vi "Control main.vi"(8 "New direction":string, 11 "Current Direction":string) -> ()   [LabVIEW 2015]
uses:
  <vilib>/myRIO/Instrument Drivers/Onboard IO/PWM/typedefs/PWM Reference.ctl
  <vilib>/myRIO/Common/Instrument Driver Framework/Utilities/typedefs/myRIO Generic Hardware Reference.ctl
  <vilib>/myRIO/Common/Instrument Driver Framework/Utilities/typedefs/Hardware Version Enum.ctl
  <vilib>/myRIO/Common/Instrument Driver Framework/Utilities/typedefs/myRIO v1.0 Reference.ctl
  <vilib>/myRIO/Common/Instrument Driver Framework/Utilities/typedefs/Generic FPGA Reference.ctl
  <vilib>/myRIO/Common/Instrument Driver Framework/myRIO v1.0/PWM/typedefs/PWM Channels Enum.ctl
  <vilib>/myRIO/Instrument Drivers/Onboard IO/PWM/typedefs/PWM Configuration.ctl
  <vilib>/userdefined/High Color/nirio_resource_hc.ctl
  <vilib>/myRIO/Common/Instrument Driver Framework/Utilities/vis/Is FPGA Ref Available.vi
  <vilib>/myRIO/Common/Instrument Driver Framework/myRIO v1.0/PWM/vis/myRIO v1.1 Open PWM.vi
  <vilib>/myRIO/Instrument Drivers/Onboard IO/PWM/vis/Set Duty Cycle and Frequency.vi
  <vilib>/myRIO/Common/Instrument Driver Framework/Utilities/vis/Validate Channels.vi
  <vilib>/myRIO/Common/Instrument Driver Framework/myRIO v1.0/PWM/vis/myRIO v1.0 Reserve PWM.vi
  <vilib>/myRIO/Common/Instrument Driver Framework/myRIO v1.0/PWM/vis/myRIO v1.0 Build MUX Configuration PWM.vi
  <vilib>/myRIO/Common/Instrument Driver Framework/myRIO v1.0/Resource Manager/vis/myRIO v1.0 Reserve Channel List.vi
  <vilib>/myRIO/Common/Instrument Driver Framework/myRIO v1.0/Resource Manager/vis/myRIO v1.0 Create Configuration List.vi
  <vilib>/myRIO/Common/Instrument Driver Framework/myRIO v1.0/Resource Manager/vis/myRIO v1.0 Reserve Channel.vi
  <vilib>/myRIO/Common/Instrument Driver Framework/myRIO v1.0/Resource Manager/vis/myRIO v1.0 Unreserve Channel.vi
  <vilib>/myRIO/Common/Instrument Driver Framework/myRIO v1.0/Resource Manager/vis/myRIO v1.0 Build Mutex Name.vi
  <vilib>/Utility/VariantDataType/GetNumericInfo.vi
  <vilib>/Utility/error.llb/Error Cluster From Error Code.vi
  <vilib>/myRIO/Common/Instrument Driver Framework/myRIO v1.0/myRIO v1.1 Open.vi
  <vilib>/myRIO/Common/Instrument Driver Framework/Utilities/vis/IO Manager.vi
  <vilib>/myRIO/Common/Instrument Driver Framework/Utilities/vis/Configuration Manager.vi
  <vilib>/myRIO/Common/Instrument Driver Framework/myRIO v1.0/Resource Manager/vis/myRIO v1.0 Configure IO.vi
  <vilib>/myRIO/Common/Instrument Driver Framework/myRIO v1.0/myRIO v1.0 Close.vi
  <vilib>/myRIO/Common/Instrument Driver Framework/myRIO v1.0/PWM/vis/myRIO v1.0 Write PWM.vi
  <vilib>/myRIO/Express VI/Onboard IO/PWM/PWM Express VI.xnode
  <vilib>/myRIO/Instrument Drivers/Onboard IO/PWM/vis/myRIO PWM Open.xnode
  <vilib>/myRIO/Instrument Drivers/Onboard IO/PWM/PWM.lvlib
panel:
  in  "error in (no error) 2":errorcluster
  out "error out 5":errorcluster
  out "error out 4":errorcluster
  out "Current location":dbl
  out "First location":dbl
  out "Final location":dbl
  out "remainder":dbl
  in  "chosen  distance":dbl
  out "error out":errorcluster
  in  "error in (no error)":errorcluster
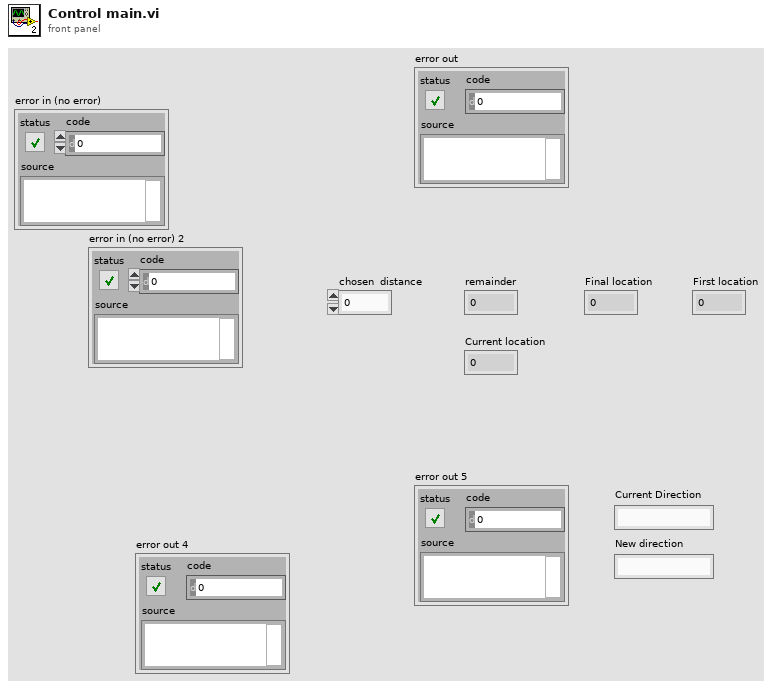
[diagram p1: front panel]
types:
  T1 = typedef "PWM.lvlib/PWM Reference.ctl" = cluster{"myRIO Reference":T2, "PWM Channels Enum":T6, "PWM Configuration":T7}
  T2 = typedef "myRIO Generic Hardware Reference.ctl" = cluster{"myRIO Model":T3, "myRIO Hardware Reference":T4}
  T3 = typedef "Hardware Version Enum.ctl" = enum16{"Unknown", "myRIO-1900", "myRIO-1950", "roboRIO"}
  T4 = typedef "myRIO v1.0 Reference.ctl" = cluster{"Generic FPGA Reference":T5, "Allow multiple opens":bool}
  T5 = typedef "Generic FPGA Reference.ctl" = refnum<k20>
  T6 = typedef "PWM Channels Enum.ctl" = enum16{"Not Connected", "C/PWM0", "C/PWM1", "A/PWM0", "A/PWM1", "A/PWM2", "B/PWM0", "B/PWM1", "B/PWM2", "PWM/PWM0", "PWM/PWM1", "PWM/PWM2", "PWM/PWM3", "PWM/PWM4", "PWM/PWM5", "PWM/PWM6", "PWM/PWM7", "PWM/PWM8", "PWM/PWM9"}
  T7 = typedef "PWM.lvlib/PWM Configuration.ctl" = cluster{"Frequency":dbl, "Duty Cycle":dbl}
  T8 = typedef "nirio_resource_hc.ctl" = tag
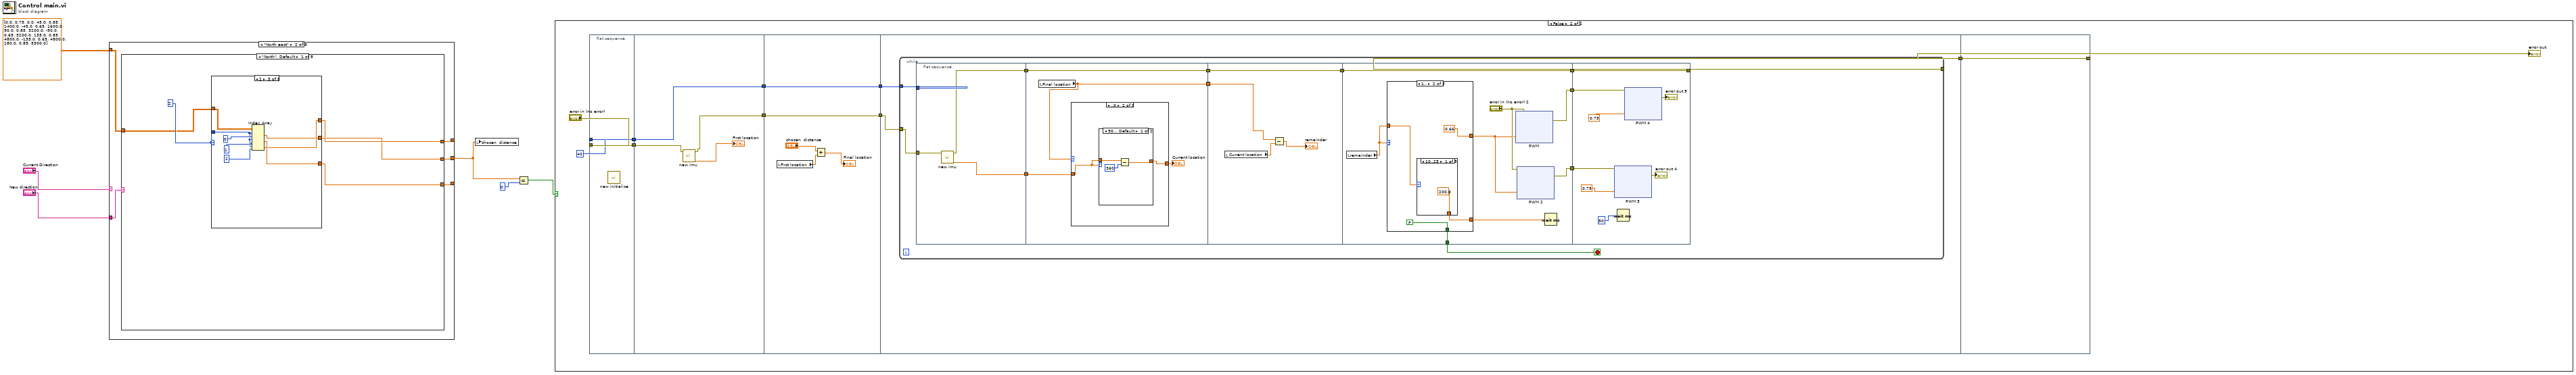
[diagram p0: block diagram]
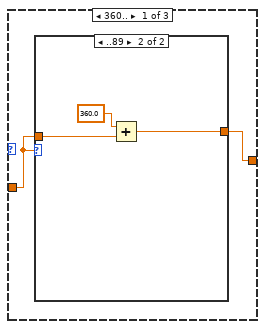
[diagram p3: hidden frame]
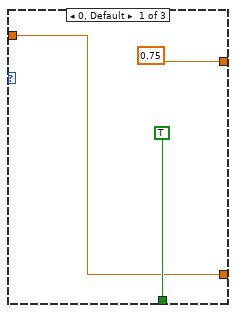
[diagram p7: hidden frame]
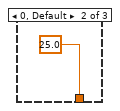
[diagram p8: hidden frame]
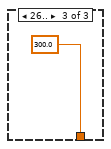
[diagram p9: hidden frame]
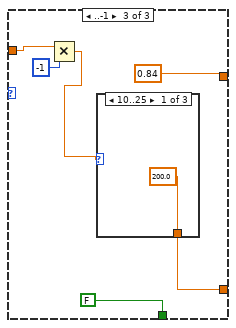
[diagram p10: hidden frame]
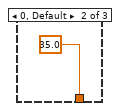
[diagram p11: hidden frame]
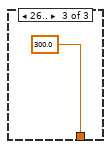
[diagram p12: hidden frame]
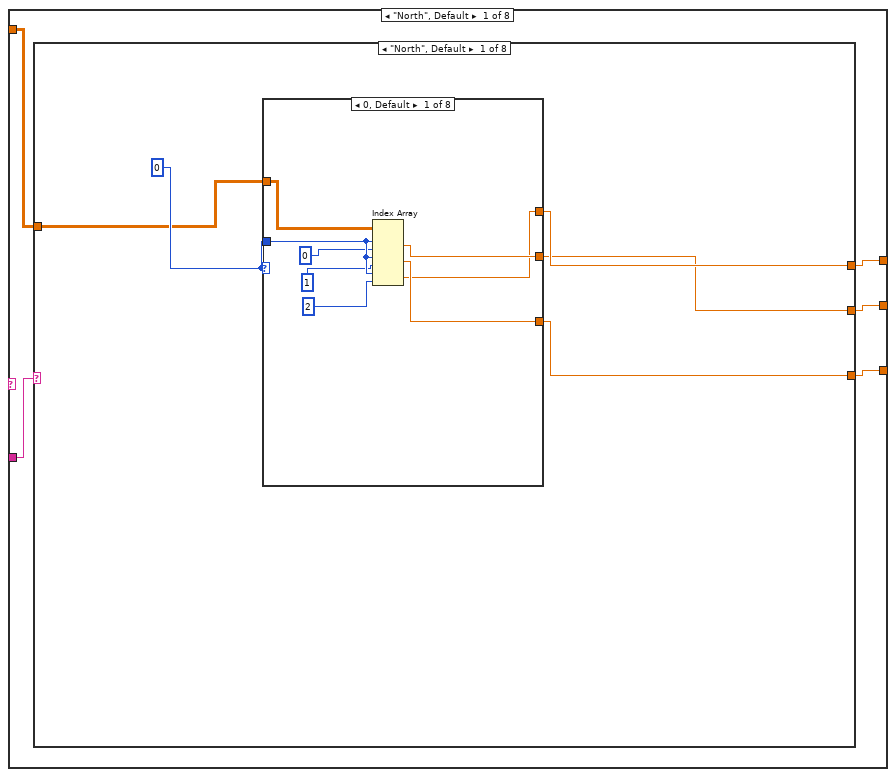
[diagram p13: hidden frame]
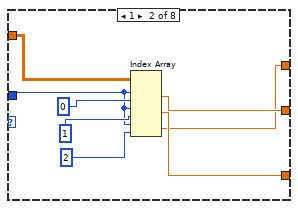
[diagram p14: hidden frame]
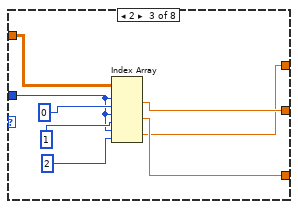
[diagram p15: hidden frame]
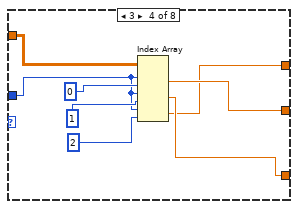
[diagram p16: hidden frame]
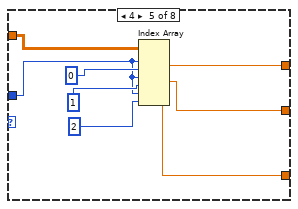
[diagram p17: hidden frame]
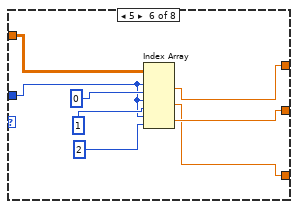
[diagram p18: hidden frame]
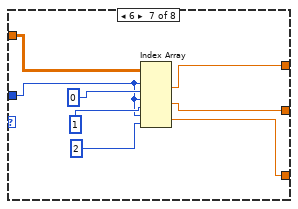
[diagram p19: hidden frame]
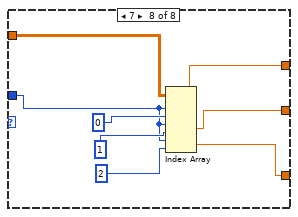
[diagram p20: hidden frame]
diagram:
  n1 = case shown="\"North east\"" "Current Direction" {
    tunnel: [w11 w568 w1125 w1682 w2239 w2796 w3353 w3910] -> _
    tunnel: [w10 w567 w1124 w1681 w2238 w2795 w3352 w3909] -> w2
    tunnel: [w9 w566 w1123 w1680 w2237 w2794 w3351 w3908] -> _
    tunnel: "New direction" -> [w7 w565 w1122 w1679 w2236 w2793 w3350 w3907]
    tunnel: dbl[][] [[0.0, 0.75, 0.0], [45.0, 0.85, 1400.0], [-45.0, 0.65, 1600.0], [90.0, 0.85, 3200.0], [-90.0, 0.65, 3200.0], [135.0, 0.85, 4800.0], [-135.0, 0.65, 4800.0], [180.0, 0.85, 5300.0]] -> [w8 w564 w1121 w1678 w2235 w2792 w3349 w3906]
    frame "North", Default {
      n2 = case shown="\"North\", Default" w7 {
        tunnel: [w15 w85 w153 w220 w290 w360 w428 w498] -> w11
        tunnel: [w14 w84 w152 w221 w289 w358 w427 w497] -> w10
        tunnel: [w13 w83 w151 w219 w288 w357 w426 w496] -> w9
        tunnel: w8 -> [w12 w81 w150 w222 w291 w359 w429 w495]
        frame "North", Default {
          w16 = 0
          n3 = case shown="0, Default" w16 {
            tunnel: [w20 w26 w34 w42 w50 w59 w66 w75] -> w15
            tunnel: [w22 w28 w36 w43 w52 w61 w68 w77] -> w14
            tunnel: [w21 w27 w35 w44 w51 w60 w67 w76] -> w13
            tunnel: w16 -> [w24 w29 w37 w45 w53 w58 w69 w74]
            tunnel: w12 -> [w17 w25 w33 w41 w49 w57 w65 w73]
            frame 0, Default {
              n4 = Index Array(array=w17, index (row) #1=w24, index (col) #1=0, index (row) #2=w24, index (col) #2=1, index (row) #3=w24, index (col) #3=2) -> (element #1=w22:dbl, element #2=w21:dbl, element #3=w20:dbl)
            }
            frame 1 {
              n5 = Index Array(array=w25, index (row) #1=w29, index (col) #1=0, index (row) #2=w29, index (col) #2=1, index (row) #3=w29, index (col) #3=2) -> (element #1=w28:dbl, element #2=w27:dbl, element #3=w26:dbl)
            }
            frame 2 {
              n6 = Index Array(array=w33, index (row) #1=w37, index (col) #1=0, index (row) #2=w37, index (col) #2=1, index (row) #3=w37, index (col) #3=2) -> (element #1=w36:dbl, element #2=w35:dbl, element #3=w34:dbl)
            }
            frame 3 {
              n7 = Index Array(array=w41, index (row) #1=w45, index (col) #1=0, index (row) #2=w45, index (col) #2=1, index (row) #3=w45, index (col) #3=2) -> (element #1=w43:dbl, element #2=w44:dbl, element #3=w42:dbl)
            }
            frame 4 {
              n8 = Index Array(array=w49, index (row) #1=w53, index (col) #1=0, index (row) #2=w53, index (col) #2=1, index (row) #3=w53, index (col) #3=2) -> (element #1=w50:dbl, element #2=w52:dbl, element #3=w51:dbl)
            }
            frame 5 {
              n9 = Index Array(array=w57, index (row) #1=w58, index (col) #1=0, index (row) #2=w58, index (col) #2=1, index (row) #3=w58, index (col) #3=2) -> (element #1=w59:dbl, element #2=w60:dbl, element #3=w61:dbl)
            }
            frame 6 {
              n10 = Index Array(array=w65, index (row) #1=w69, index (col) #1=0, index (row) #2=w69, index (col) #2=1, index (row) #3=w69, index (col) #3=2) -> (element #1=w66:dbl, element #2=w68:dbl, element #3=w67:dbl)
            }
            frame 7 {
              n11 = Index Array(array=w73, index (row) #1=w74, index (col) #1=0, index (row) #2=w74, index (col) #2=1, index (row) #3=w74, index (col) #3=2) -> (element #1=w75:dbl, element #2=w77:dbl, element #3=w76:dbl)
            }
          }
        }
        frame "North east" {
          w82 = 1
          n12 = case shown="2" w82 {
            tunnel: [w89 w95 w103 w111 w119 w128 w135 w144] -> w85
            tunnel: [w91 w97 w105 w112 w121 w130 w137 w146] -> w84
            tunnel: [w90 w96 w104 w113 w120 w129 w136 w145] -> w83
            tunnel: w82 -> [w93 w98 w106 w114 w122 w127 w138 w143]
            tunnel: w81 -> [w86 w94 w102 w110 w118 w126 w134 w142]
            frame 0, Default {
              n13 = Index Array(array=w86, index (row) #1=w93, index (col) #1=0, index (row) #2=w93, index (col) #2=1, index (row) #3=w93, index (col) #3=2) -> (element #1=w91:dbl, element #2=w90:dbl, element #3=w89:dbl)
            }
            frame 1 {
              n14 = Index Array(array=w94, index (row) #1=w98, index (col) #1=0, index (row) #2=w98, index (col) #2=1, index (row) #3=w98, index (col) #3=2) -> (element #1=w97:dbl, element #2=w96:dbl, element #3=w95:dbl)
            }
            frame 2 {
              n15 = Index Array(array=w102, index (row) #1=w106, index (col) #1=0, index (row) #2=w106, index (col) #2=1, index (row) #3=w106, index (col) #3=2) -> (element #1=w105:dbl, element #2=w104:dbl, element #3=w103:dbl)
            }
            frame 3 {
              n16 = Index Array(array=w110, index (row) #1=w114, index (col) #1=0, index (row) #2=w114, index (col) #2=1, index (row) #3=w114, index (col) #3=2) -> (element #1=w112:dbl, element #2=w113:dbl, element #3=w111:dbl)
            }
            frame 4 {
              n17 = Index Array(array=w118, index (row) #1=w122, index (col) #1=0, index (row) #2=w122, index (col) #2=1, index (row) #3=w122, index (col) #3=2) -> (element #1=w119:dbl, element #2=w121:dbl, element #3=w120:dbl)
            }
            frame 5 {
              n18 = Index Array(array=w126, index (row) #1=w127, index (col) #1=0, index (row) #2=w127, index (col) #2=1, index (row) #3=w127, index (col) #3=2) -> (element #1=w128:dbl, element #2=w129:dbl, element #3=w130:dbl)
            }
            frame 6 {
              n19 = Index Array(array=w134, index (row) #1=w138, index (col) #1=0, index (row) #2=w138, index (col) #2=1, index (row) #3=w138, index (col) #3=2) -> (element #1=w135:dbl, element #2=w137:dbl, element #3=w136:dbl)
            }
            frame 7 {
              n20 = Index Array(array=w142, index (row) #1=w143, index (col) #1=0, index (row) #2=w143, index (col) #2=1, index (row) #3=w143, index (col) #3=2) -> (element #1=w144:dbl, element #2=w146:dbl, element #3=w145:dbl)
            }
          }
        }
        frame "North west" {
          w154 = 2
          n21 = case shown="2" w154 {
            tunnel: [w158 w164 w172 w180 w188 w197 w204 w213] -> w153
            tunnel: [w160 w166 w174 w181 w190 w199 w206 w215] -> w152
            tunnel: [w159 w165 w173 w182 w189 w198 w205 w214] -> w151
            tunnel: w154 -> [w162 w167 w175 w183 w191 w196 w207 w212]
            tunnel: w150 -> [w155 w163 w171 w179 w187 w195 w203 w211]
            frame 0, Default {
              n22 = Index Array(array=w155, index (row) #1=w162, index (col) #1=0, index (row) #2=w162, index (col) #2=1, index (row) #3=w162, index (col) #3=2) -> (element #1=w160:dbl, element #2=w159:dbl, element #3=w158:dbl)
            }
            frame 1 {
              n23 = Index Array(array=w163, index (row) #1=w167, index (col) #1=0, index (row) #2=w167, index (col) #2=1, index (row) #3=w167, index (col) #3=2) -> (element #1=w166:dbl, element #2=w165:dbl, element #3=w164:dbl)
            }
            frame 2 {
              n24 = Index Array(array=w171, index (row) #1=w175, index (col) #1=0, index (row) #2=w175, index (col) #2=1, index (row) #3=w175, index (col) #3=2) -> (element #1=w174:dbl, element #2=w173:dbl, element #3=w172:dbl)
            }
            frame 3 {
              n25 = Index Array(array=w179, index (row) #1=w183, index (col) #1=0, index (row) #2=w183, index (col) #2=1, index (row) #3=w183, index (col) #3=2) -> (element #1=w181:dbl, element #2=w182:dbl, element #3=w180:dbl)
            }
            frame 4 {
              n26 = Index Array(array=w187, index (row) #1=w191, index (col) #1=0, index (row) #2=w191, index (col) #2=1, index (row) #3=w191, index (col) #3=2) -> (element #1=w188:dbl, element #2=w190:dbl, element #3=w189:dbl)
            }
            frame 5 {
              n27 = Index Array(array=w195, index (row) #1=w196, index (col) #1=0, index (row) #2=w196, index (col) #2=1, index (row) #3=w196, index (col) #3=2) -> (element #1=w197:dbl, element #2=w198:dbl, element #3=w199:dbl)
            }
            frame 6 {
              n28 = Index Array(array=w203, index (row) #1=w207, index (col) #1=0, index (row) #2=w207, index (col) #2=1, index (row) #3=w207, index (col) #3=2) -> (element #1=w204:dbl, element #2=w206:dbl, element #3=w205:dbl)
            }
            frame 7 {
              n29 = Index Array(array=w211, index (row) #1=w212, index (col) #1=0, index (row) #2=w212, index (col) #2=1, index (row) #3=w212, index (col) #3=2) -> (element #1=w213:dbl, element #2=w215:dbl, element #3=w214:dbl)
            }
          }
        }
        frame "West" {
          w223 = 4
          n30 = case shown="2" w223 {
            tunnel: [w227 w233 w241 w249 w257 w266 w273 w282] -> w220
            tunnel: [w229 w235 w243 w250 w259 w268 w275 w284] -> w221
            tunnel: [w228 w234 w242 w251 w258 w267 w274 w283] -> w219
            tunnel: w223 -> [w231 w236 w244 w252 w260 w265 w276 w281]
            tunnel: w222 -> [w224 w232 w240 w248 w256 w264 w272 w280]
            frame 0, Default {
              n31 = Index Array(array=w224, index (row) #1=w231, index (col) #1=0, index (row) #2=w231, index (col) #2=1, index (row) #3=w231, index (col) #3=2) -> (element #1=w229:dbl, element #2=w228:dbl, element #3=w227:dbl)
            }
            frame 1 {
              n32 = Index Array(array=w232, index (row) #1=w236, index (col) #1=0, index (row) #2=w236, index (col) #2=1, index (row) #3=w236, index (col) #3=2) -> (element #1=w235:dbl, element #2=w234:dbl, element #3=w233:dbl)
            }
            frame 2 {
              n33 = Index Array(array=w240, index (row) #1=w244, index (col) #1=0, index (row) #2=w244, index (col) #2=1, index (row) #3=w244, index (col) #3=2) -> (element #1=w243:dbl, element #2=w242:dbl, element #3=w241:dbl)
            }
            frame 3 {
              n34 = Index Array(array=w248, index (row) #1=w252, index (col) #1=0, index (row) #2=w252, index (col) #2=1, index (row) #3=w252, index (col) #3=2) -> (element #1=w250:dbl, element #2=w251:dbl, element #3=w249:dbl)
            }
            frame 4 {
              n35 = Index Array(array=w256, index (row) #1=w260, index (col) #1=0, index (row) #2=w260, index (col) #2=1, index (row) #3=w260, index (col) #3=2) -> (element #1=w257:dbl, element #2=w259:dbl, element #3=w258:dbl)
            }
            frame 5 {
              n36 = Index Array(array=w264, index (row) #1=w265, index (col) #1=0, index (row) #2=w265, index (col) #2=1, index (row) #3=w265, index (col) #3=2) -> (element #1=w266:dbl, element #2=w267:dbl, element #3=w268:dbl)
            }
            frame 6 {
              n37 = Index Array(array=w272, index (row) #1=w276, index (col) #1=0, index (row) #2=w276, index (col) #2=1, index (row) #3=w276, index (col) #3=2) -> (element #1=w273:dbl, element #2=w275:dbl, element #3=w274:dbl)
            }
            frame 7 {
              n38 = Index Array(array=w280, index (row) #1=w281, index (col) #1=0, index (row) #2=w281, index (col) #2=1, index (row) #3=w281, index (col) #3=2) -> (element #1=w282:dbl, element #2=w284:dbl, element #3=w283:dbl)
            }
          }
        }
        frame "East" {
          w292 = 3
          n39 = case shown="2" w292 {
            tunnel: [w296 w302 w310 w318 w326 w335 w342 w351] -> w290
            tunnel: [w298 w304 w312 w319 w328 w337 w344 w353] -> w289
            tunnel: [w297 w303 w311 w320 w327 w336 w343 w352] -> w288
            tunnel: w292 -> [w300 w305 w313 w321 w329 w334 w345 w350]
            tunnel: w291 -> [w293 w301 w309 w317 w325 w333 w341 w349]
            frame 0, Default {
              n40 = Index Array(array=w293, index (row) #1=w300, index (col) #1=0, index (row) #2=w300, index (col) #2=1, index (row) #3=w300, index (col) #3=2) -> (element #1=w298:dbl, element #2=w297:dbl, element #3=w296:dbl)
            }
            frame 1 {
              n41 = Index Array(array=w301, index (row) #1=w305, index (col) #1=0, index (row) #2=w305, index (col) #2=1, index (row) #3=w305, index (col) #3=2) -> (element #1=w304:dbl, element #2=w303:dbl, element #3=w302:dbl)
            }
            frame 2 {
              n42 = Index Array(array=w309, index (row) #1=w313, index (col) #1=0, index (row) #2=w313, index (col) #2=1, index (row) #3=w313, index (col) #3=2) -> (element #1=w312:dbl, element #2=w311:dbl, element #3=w310:dbl)
            }
            frame 3 {
              n43 = Index Array(array=w317, index (row) #1=w321, index (col) #1=0, index (row) #2=w321, index (col) #2=1, index (row) #3=w321, index (col) #3=2) -> (element #1=w319:dbl, element #2=w320:dbl, element #3=w318:dbl)
            }
            frame 4 {
              n44 = Index Array(array=w325, index (row) #1=w329, index (col) #1=0, index (row) #2=w329, index (col) #2=1, index (row) #3=w329, index (col) #3=2) -> (element #1=w326:dbl, element #2=w328:dbl, element #3=w327:dbl)
            }
            frame 5 {
              n45 = Index Array(array=w333, index (row) #1=w334, index (col) #1=0, index (row) #2=w334, index (col) #2=1, index (row) #3=w334, index (col) #3=2) -> (element #1=w335:dbl, element #2=w336:dbl, element #3=w337:dbl)
            }
            frame 6 {
              n46 = Index Array(array=w341, index (row) #1=w345, index (col) #1=0, index (row) #2=w345, index (col) #2=1, index (row) #3=w345, index (col) #3=2) -> (element #1=w342:dbl, element #2=w344:dbl, element #3=w343:dbl)
            }
            frame 7 {
              n47 = Index Array(array=w349, index (row) #1=w350, index (col) #1=0, index (row) #2=w350, index (col) #2=1, index (row) #3=w350, index (col) #3=2) -> (element #1=w351:dbl, element #2=w353:dbl, element #3=w352:dbl)
            }
          }
        }
        frame "South" {
          w361 = 7
          n48 = case shown="2" w361 {
            tunnel: [w365 w371 w379 w387 w395 w404 w411 w420] -> w360
            tunnel: [w367 w373 w381 w388 w397 w406 w413 w422] -> w358
            tunnel: [w366 w372 w380 w389 w396 w405 w412 w421] -> w357
            tunnel: w361 -> [w369 w374 w382 w390 w398 w403 w414 w419]
            tunnel: w359 -> [w362 w370 w378 w386 w394 w402 w410 w418]
            frame 0, Default {
              n49 = Index Array(array=w362, index (row) #1=w369, index (col) #1=0, index (row) #2=w369, index (col) #2=1, index (row) #3=w369, index (col) #3=2) -> (element #1=w367:dbl, element #2=w366:dbl, element #3=w365:dbl)
            }
            frame 1 {
              n50 = Index Array(array=w370, index (row) #1=w374, index (col) #1=0, index (row) #2=w374, index (col) #2=1, index (row) #3=w374, index (col) #3=2) -> (element #1=w373:dbl, element #2=w372:dbl, element #3=w371:dbl)
            }
            frame 2 {
              n51 = Index Array(array=w378, index (row) #1=w382, index (col) #1=0, index (row) #2=w382, index (col) #2=1, index (row) #3=w382, index (col) #3=2) -> (element #1=w381:dbl, element #2=w380:dbl, element #3=w379:dbl)
            }
            frame 3 {
              n52 = Index Array(array=w386, index (row) #1=w390, index (col) #1=0, index (row) #2=w390, index (col) #2=1, index (row) #3=w390, index (col) #3=2) -> (element #1=w388:dbl, element #2=w389:dbl, element #3=w387:dbl)
            }
            frame 4 {
              n53 = Index Array(array=w394, index (row) #1=w398, index (col) #1=0, index (row) #2=w398, index (col) #2=1, index (row) #3=w398, index (col) #3=2) -> (element #1=w395:dbl, element #2=w397:dbl, element #3=w396:dbl)
            }
            frame 5 {
              n54 = Index Array(array=w402, index (row) #1=w403, index (col) #1=0, index (row) #2=w403, index (col) #2=1, index (row) #3=w403, index (col) #3=2) -> (element #1=w404:dbl, element #2=w405:dbl, element #3=w406:dbl)
            }
            frame 6 {
              n55 = Index Array(array=w410, index (row) #1=w414, index (col) #1=0, index (row) #2=w414, index (col) #2=1, index (row) #3=w414, index (col) #3=2) -> (element #1=w411:dbl, element #2=w413:dbl, element #3=w412:dbl)
            }
            frame 7 {
              n56 = Index Array(array=w418, index (row) #1=w419, index (col) #1=0, index (row) #2=w419, index (col) #2=1, index (row) #3=w419, index (col) #3=2) -> (element #1=w420:dbl, element #2=w422:dbl, element #3=w421:dbl)
            }
          }
        }
        frame "South west" {
          w430 = 6
          n57 = case shown="2" w430 {
            tunnel: [w434 w440 w448 w456 w464 w473 w480 w489] -> w428
            tunnel: [w436 w442 w450 w457 w466 w475 w482 w491] -> w427
            tunnel: [w435 w441 w449 w458 w465 w474 w481 w490] -> w426
            tunnel: w430 -> [w438 w443 w451 w459 w467 w472 w483 w488]
            tunnel: w429 -> [w431 w439 w447 w455 w463 w471 w479 w487]
            frame 0, Default {
              n58 = Index Array(array=w431, index (row) #1=w438, index (col) #1=0, index (row) #2=w438, index (col) #2=1, index (row) #3=w438, index (col) #3=2) -> (element #1=w436:dbl, element #2=w435:dbl, element #3=w434:dbl)
            }
            frame 1 {
              n59 = Index Array(array=w439, index (row) #1=w443, index (col) #1=0, index (row) #2=w443, index (col) #2=1, index (row) #3=w443, index (col) #3=2) -> (element #1=w442:dbl, element #2=w441:dbl, element #3=w440:dbl)
            }
            frame 2 {
              n60 = Index Array(array=w447, index (row) #1=w451, index (col) #1=0, index (row) #2=w451, index (col) #2=1, index (row) #3=w451, index (col) #3=2) -> (element #1=w450:dbl, element #2=w449:dbl, element #3=w448:dbl)
            }
            frame 3 {
              n61 = Index Array(array=w455, index (row) #1=w459, index (col) #1=0, index (row) #2=w459, index (col) #2=1, index (row) #3=w459, index (col) #3=2) -> (element #1=w457:dbl, element #2=w458:dbl, element #3=w456:dbl)
            }
            frame 4 {
              n62 = Index Array(array=w463, index (row) #1=w467, index (col) #1=0, index (row) #2=w467, index (col) #2=1, index (row) #3=w467, index (col) #3=2) -> (element #1=w464:dbl, element #2=w466:dbl, element #3=w465:dbl)
            }
            frame 5 {
              n63 = Index Array(array=w471, index (row) #1=w472, index (col) #1=0, index (row) #2=w472, index (col) #2=1, index (row) #3=w472, index (col) #3=2) -> (element #1=w473:dbl, element #2=w474:dbl, element #3=w475:dbl)
            }
            frame 6 {
              n64 = Index Array(array=w479, index (row) #1=w483, index (col) #1=0, index (row) #2=w483, index (col) #2=1, index (row) #3=w483, index (col) #3=2) -> (element #1=w480:dbl, element #2=w482:dbl, element #3=w481:dbl)
            }
            frame 7 {
              n65 = Index Array(array=w487, index (row) #1=w488, index (col) #1=0, index (row) #2=w488, index (col) #2=1, index (row) #3=w488, index (col) #3=2) -> (element #1=w489:dbl, element #2=w491:dbl, element #3=w490:dbl)
            }
          }
        }
        frame "South east" {
          w499 = 5
          n66 = case shown="2" w499 {
            tunnel: [w503 w509 w517 w525 w533 w542 w549 w558] -> w498
            tunnel: [w505 w511 w519 w526 w535 w544 w551 w560] -> w497
            tunnel: [w504 w510 w518 w527 w534 w543 w550 w559] -> w496
            tunnel: w499 -> [w507 w512 w520 w528 w536 w541 w552 w557]
            tunnel: w495 -> [w500 w508 w516 w524 w532 w540 w548 w556]
            frame 0, Default {
              n67 = Index Array(array=w500, index (row) #1=w507, index (col) #1=0, index (row) #2=w507, index (col) #2=1, index (row) #3=w507, index (col) #3=2) -> (element #1=w505:dbl, element #2=w504:dbl, element #3=w503:dbl)
            }
            frame 1 {
              n68 = Index Array(array=w508, index (row) #1=w512, index (col) #1=0, index (row) #2=w512, index (col) #2=1, index (row) #3=w512, index (col) #3=2) -> (element #1=w511:dbl, element #2=w510:dbl, element #3=w509:dbl)
            }
            frame 2 {
              n69 = Index Array(array=w516, index (row) #1=w520, index (col) #1=0, index (row) #2=w520, index (col) #2=1, index (row) #3=w520, index (col) #3=2) -> (element #1=w519:dbl, element #2=w518:dbl, element #3=w517:dbl)
            }
            frame 3 {
              n70 = Index Array(array=w524, index (row) #1=w528, index (col) #1=0, index (row) #2=w528, index (col) #2=1, index (row) #3=w528, index (col) #3=2) -> (element #1=w526:dbl, element #2=w527:dbl, element #3=w525:dbl)
            }
            frame 4 {
              n71 = Index Array(array=w532, index (row) #1=w536, index (col) #1=0, index (row) #2=w536, index (col) #2=1, index (row) #3=w536, index (col) #3=2) -> (element #1=w533:dbl, element #2=w535:dbl, element #3=w534:dbl)
            }
            frame 5 {
              n72 = Index Array(array=w540, index (row) #1=w541, index (col) #1=0, index (row) #2=w541, index (col) #2=1, index (row) #3=w541, index (col) #3=2) -> (element #1=w542:dbl, element #2=w543:dbl, element #3=w544:dbl)
            }
            frame 6 {
              n73 = Index Array(array=w548, index (row) #1=w552, index (col) #1=0, index (row) #2=w552, index (col) #2=1, index (row) #3=w552, index (col) #3=2) -> (element #1=w549:dbl, element #2=w551:dbl, element #3=w550:dbl)
            }
            frame 7 {
              n74 = Index Array(array=w556, index (row) #1=w557, index (col) #1=0, index (row) #2=w557, index (col) #2=1, index (row) #3=w557, index (col) #3=2) -> (element #1=w558:dbl, element #2=w560:dbl, element #3=w559:dbl)
            }
          }
        }
      }
    }
    frame "North east" {
      n75 = case shown="\"North\", Default" w565 {
        tunnel: [w572 w642 w710 w777 w847 w917 w985 w1055] -> w568
        tunnel: [w571 w641 w709 w778 w846 w915 w984 w1054] -> w567
        tunnel: [w570 w640 w708 w776 w845 w914 w983 w1053] -> w566
        tunnel: w564 -> [w569 w638 w707 w779 w848 w916 w986 w1052]
        frame "North", Default {
          w573 = 2
          n76 = case shown="2" w573 {
            tunnel: [w577 w583 w591 w599 w607 w616 w623 w632] -> w572
            tunnel: [w579 w585 w593 w600 w609 w618 w625 w634] -> w571
            tunnel: [w578 w584 w592 w601 w608 w617 w624 w633] -> w570
            tunnel: w573 -> [w581 w586 w594 w602 w610 w615 w626 w631]
            tunnel: w569 -> [w574 w582 w590 w598 w606 w614 w622 w630]
            frame 0, Default {
              n77 = Index Array(array=w574, index (row) #1=w581, index (col) #1=0, index (row) #2=w581, index (col) #2=1, index (row) #3=w581, index (col) #3=2) -> (element #1=w579:dbl, element #2=w578:dbl, element #3=w577:dbl)
            }
            frame 1 {
              n78 = Index Array(array=w582, index (row) #1=w586, index (col) #1=0, index (row) #2=w586, index (col) #2=1, index (row) #3=w586, index (col) #3=2) -> (element #1=w585:dbl, element #2=w584:dbl, element #3=w583:dbl)
            }
            frame 2 {
              n79 = Index Array(array=w590, index (row) #1=w594, index (col) #1=0, index (row) #2=w594, index (col) #2=1, index (row) #3=w594, index (col) #3=2) -> (element #1=w593:dbl, element #2=w592:dbl, element #3=w591:dbl)
            }
            frame 3 {
              n80 = Index Array(array=w598, index (row) #1=w602, index (col) #1=0, index (row) #2=w602, index (col) #2=1, index (row) #3=w602, index (col) #3=2) -> (element #1=w600:dbl, element #2=w601:dbl, element #3=w599:dbl)
            }
            frame 4 {
              n81 = Index Array(array=w606, index (row) #1=w610, index (col) #1=0, index (row) #2=w610, index (col) #2=1, index (row) #3=w610, index (col) #3=2) -> (element #1=w607:dbl, element #2=w609:dbl, element #3=w608:dbl)
            }
            frame 5 {
              n82 = Index Array(array=w614, index (row) #1=w615, index (col) #1=0, index (row) #2=w615, index (col) #2=1, index (row) #3=w615, index (col) #3=2) -> (element #1=w616:dbl, element #2=w617:dbl, element #3=w618:dbl)
            }
            frame 6 {
              n83 = Index Array(array=w622, index (row) #1=w626, index (col) #1=0, index (row) #2=w626, index (col) #2=1, index (row) #3=w626, index (col) #3=2) -> (element #1=w623:dbl, element #2=w625:dbl, element #3=w624:dbl)
            }
            frame 7 {
              n84 = Index Array(array=w630, index (row) #1=w631, index (col) #1=0, index (row) #2=w631, index (col) #2=1, index (row) #3=w631, index (col) #3=2) -> (element #1=w632:dbl, element #2=w634:dbl, element #3=w633:dbl)
            }
          }
        }
        frame "North east" {
          w639 = 0
          n85 = case shown="2" w639 {
            tunnel: [w646 w652 w660 w668 w676 w685 w692 w701] -> w642
            tunnel: [w648 w654 w662 w669 w678 w687 w694 w703] -> w641
            tunnel: [w647 w653 w661 w670 w677 w686 w693 w702] -> w640
            tunnel: w639 -> [w650 w655 w663 w671 w679 w684 w695 w700]
            tunnel: w638 -> [w643 w651 w659 w667 w675 w683 w691 w699]
            frame 0, Default {
              n86 = Index Array(array=w643, index (row) #1=w650, index (col) #1=0, index (row) #2=w650, index (col) #2=1, index (row) #3=w650, index (col) #3=2) -> (element #1=w648:dbl, element #2=w647:dbl, element #3=w646:dbl)
            }
            frame 1 {
              n87 = Index Array(array=w651, index (row) #1=w655, index (col) #1=0, index (row) #2=w655, index (col) #2=1, index (row) #3=w655, index (col) #3=2) -> (element #1=w654:dbl, element #2=w653:dbl, element #3=w652:dbl)
            }
            frame 2 {
              n88 = Index Array(array=w659, index (row) #1=w663, index (col) #1=0, index (row) #2=w663, index (col) #2=1, index (row) #3=w663, index (col) #3=2) -> (element #1=w662:dbl, element #2=w661:dbl, element #3=w660:dbl)
            }
            frame 3 {
              n89 = Index Array(array=w667, index (row) #1=w671, index (col) #1=0, index (row) #2=w671, index (col) #2=1, index (row) #3=w671, index (col) #3=2) -> (element #1=w669:dbl, element #2=w670:dbl, element #3=w668:dbl)
            }
            frame 4 {
              n90 = Index Array(array=w675, index (row) #1=w679, index (col) #1=0, index (row) #2=w679, index (col) #2=1, index (row) #3=w679, index (col) #3=2) -> (element #1=w676:dbl, element #2=w678:dbl, element #3=w677:dbl)
            }
            frame 5 {
              n91 = Index Array(array=w683, index (row) #1=w684, index (col) #1=0, index (row) #2=w684, index (col) #2=1, index (row) #3=w684, index (col) #3=2) -> (element #1=w685:dbl, element #2=w686:dbl, element #3=w687:dbl)
            }
            frame 6 {
              n92 = Index Array(array=w691, index (row) #1=w695, index (col) #1=0, index (row) #2=w695, index (col) #2=1, index (row) #3=w695, index (col) #3=2) -> (element #1=w692:dbl, element #2=w694:dbl, element #3=w693:dbl)
            }
            frame 7 {
              n93 = Index Array(array=w699, index (row) #1=w700, index (col) #1=0, index (row) #2=w700, index (col) #2=1, index (row) #3=w700, index (col) #3=2) -> (element #1=w701:dbl, element #2=w703:dbl, element #3=w702:dbl)
            }
          }
        }
        frame "North west" {
          w711 = 4
          n94 = case shown="2" w711 {
            tunnel: [w715 w721 w729 w737 w745 w754 w761 w770] -> w710
            tunnel: [w717 w723 w731 w738 w747 w756 w763 w772] -> w709
            tunnel: [w716 w722 w730 w739 w746 w755 w762 w771] -> w708
            tunnel: w711 -> [w719 w724 w732 w740 w748 w753 w764 w769]
            tunnel: w707 -> [w712 w720 w728 w736 w744 w752 w760 w768]
            frame 0, Default {
              n95 = Index Array(array=w712, index (row) #1=w719, index (col) #1=0, index (row) #2=w719, index (col) #2=1, index (row) #3=w719, index (col) #3=2) -> (element #1=w717:dbl, element #2=w716:dbl, element #3=w715:dbl)
            }
            frame 1 {
              n96 = Index Array(array=w720, index (row) #1=w724, index (col) #1=0, index (row) #2=w724, index (col) #2=1, index (row) #3=w724, index (col) #3=2) -> (element #1=w723:dbl, element #2=w722:dbl, element #3=w721:dbl)
            }
            frame 2 {
              n97 = Index Array(array=w728, index (row) #1=w732, index (col) #1=0, index (row) #2=w732, index (col) #2=1, index (row) #3=w732, index (col) #3=2) -> (element #1=w731:dbl, element #2=w730:dbl, element #3=w729:dbl)
            }
            frame 3 {
              n98 = Index Array(array=w736, index (row) #1=w740, index (col) #1=0, index (row) #2=w740, index (col) #2=1, index (row) #3=w740, index (col) #3=2) -> (element #1=w738:dbl, element #2=w739:dbl, element #3=w737:dbl)
            }
            frame 4 {
              n99 = Index Array(array=w744, index (row) #1=w748, index (col) #1=0, index (row) #2=w748, index (col) #2=1, index (row) #3=w748, index (col) #3=2) -> (element #1=w745:dbl, element #2=w747:dbl, element #3=w746:dbl)
            }
            frame 5 {
              n100 = Index Array(array=w752, index (row) #1=w753, index (col) #1=0, index (row) #2=w753, index (col) #2=1, index (row) #3=w753, index (col) #3=2) -> (element #1=w754:dbl, element #2=w755:dbl, element #3=w756:dbl)
            }
            frame 6 {
              n101 = Index Array(array=w760, index (row) #1=w764, index (col) #1=0, index (row) #2=w764, index (col) #2=1, index (row) #3=w764, index (col) #3=2) -> (element #1=w761:dbl, element #2=w763:dbl, element #3=w762:dbl)
            }
            frame 7 {
              n102 = Index Array(array=w768, index (row) #1=w769, index (col) #1=0, index (row) #2=w769, index (col) #2=1, index (row) #3=w769, index (col) #3=2) -> (element #1=w770:dbl, element #2=w772:dbl, element #3=w771:dbl)
            }
          }
        }
        frame "West" {
          w780 = 6
          n103 = case shown="2" w780 {
            tunnel: [w784 w790 w798 w806 w814 w823 w830 w839] -> w777
            tunnel: [w786 w792 w800 w807 w816 w825 w832 w841] -> w778
            tunnel: [w785 w791 w799 w808 w815 w824 w831 w840] -> w776
            tunnel: w780 -> [w788 w793 w801 w809 w817 w822 w833 w838]
            tunnel: w779 -> [w781 w789 w797 w805 w813 w821 w829 w837]
            frame 0, Default {
              n104 = Index Array(array=w781, index (row) #1=w788, index (col) #1=0, index (row) #2=w788, index (col) #2=1, index (row) #3=w788, index (col) #3=2) -> (element #1=w786:dbl, element #2=w785:dbl, element #3=w784:dbl)
            }
            frame 1 {
              n105 = Index Array(array=w789, index (row) #1=w793, index (col) #1=0, index (row) #2=w793, index (col) #2=1, index (row) #3=w793, index (col) #3=2) -> (element #1=w792:dbl, element #2=w791:dbl, element #3=w790:dbl)
            }
            frame 2 {
              n106 = Index Array(array=w797, index (row) #1=w801, index (col) #1=0, index (row) #2=w801, index (col) #2=1, index (row) #3=w801, index (col) #3=2) -> (element #1=w800:dbl, element #2=w799:dbl, element #3=w798:dbl)
            }
            frame 3 {
              n107 = Index Array(array=w805, index (row) #1=w809, index (col) #1=0, index (row) #2=w809, index (col) #2=1, index (row) #3=w809, index (col) #3=2) -> (element #1=w807:dbl, element #2=w808:dbl, element #3=w806:dbl)
            }
            frame 4 {
              n108 = Index Array(array=w813, index (row) #1=w817, index (col) #1=0, index (row) #2=w817, index (col) #2=1, index (row) #3=w817, index (col) #3=2) -> (element #1=w814:dbl, element #2=w816:dbl, element #3=w815:dbl)
            }
            frame 5 {
              n109 = Index Array(array=w821, index (row) #1=w822, index (col) #1=0, index (row) #2=w822, index (col) #2=1, index (row) #3=w822, index (col) #3=2) -> (element #1=w823:dbl, element #2=w824:dbl, element #3=w825:dbl)
            }
            frame 6 {
              n110 = Index Array(array=w829, index (row) #1=w833, index (col) #1=0, index (row) #2=w833, index (col) #2=1, index (row) #3=w833, index (col) #3=2) -> (element #1=w830:dbl, element #2=w832:dbl, element #3=w831:dbl)
            }
            frame 7 {
              n111 = Index Array(array=w837, index (row) #1=w838, index (col) #1=0, index (row) #2=w838, index (col) #2=1, index (row) #3=w838, index (col) #3=2) -> (element #1=w839:dbl, element #2=w841:dbl, element #3=w840:dbl)
            }
          }
        }
        frame "East" {
          w849 = 1
          n112 = case shown="2" w849 {
            tunnel: [w853 w859 w867 w875 w883 w892 w899 w908] -> w847
            tunnel: [w855 w861 w869 w876 w885 w894 w901 w910] -> w846
            tunnel: [w854 w860 w868 w877 w884 w893 w900 w909] -> w845
            tunnel: w849 -> [w857 w862 w870 w878 w886 w891 w902 w907]
            tunnel: w848 -> [w850 w858 w866 w874 w882 w890 w898 w906]
            frame 0, Default {
              n113 = Index Array(array=w850, index (row) #1=w857, index (col) #1=0, index (row) #2=w857, index (col) #2=1, index (row) #3=w857, index (col) #3=2) -> (element #1=w855:dbl, element #2=w854:dbl, element #3=w853:dbl)
            }
            frame 1 {
              n114 = Index Array(array=w858, index (row) #1=w862, index (col) #1=0, index (row) #2=w862, index (col) #2=1, index (row) #3=w862, index (col) #3=2) -> (element #1=w861:dbl, element #2=w860:dbl, element #3=w859:dbl)
            }
            frame 2 {
              n115 = Index Array(array=w866, index (row) #1=w870, index (col) #1=0, index (row) #2=w870, index (col) #2=1, index (row) #3=w870, index (col) #3=2) -> (element #1=w869:dbl, element #2=w868:dbl, element #3=w867:dbl)
            }
            frame 3 {
              n116 = Index Array(array=w874, index (row) #1=w878, index (col) #1=0, index (row) #2=w878, index (col) #2=1, index (row) #3=w878, index (col) #3=2) -> (element #1=w876:dbl, element #2=w877:dbl, element #3=w875:dbl)
            }
            frame 4 {
              n117 = Index Array(array=w882, index (row) #1=w886, index (col) #1=0, index (row) #2=w886, index (col) #2=1, index (row) #3=w886, index (col) #3=2) -> (element #1=w883:dbl, element #2=w885:dbl, element #3=w884:dbl)
            }
            frame 5 {
              n118 = Index Array(array=w890, index (row) #1=w891, index (col) #1=0, index (row) #2=w891, index (col) #2=1, index (row) #3=w891, index (col) #3=2) -> (element #1=w892:dbl, element #2=w893:dbl, element #3=w894:dbl)
            }
            frame 6 {
              n119 = Index Array(array=w898, index (row) #1=w902, index (col) #1=0, index (row) #2=w902, index (col) #2=1, index (row) #3=w902, index (col) #3=2) -> (element #1=w899:dbl, element #2=w901:dbl, element #3=w900:dbl)
            }
            frame 7 {
              n120 = Index Array(array=w906, index (row) #1=w907, index (col) #1=0, index (row) #2=w907, index (col) #2=1, index (row) #3=w907, index (col) #3=2) -> (element #1=w908:dbl, element #2=w910:dbl, element #3=w909:dbl)
            }
          }
        }
        frame "South" {
          w918 = 5
          n121 = case shown="2" w918 {
            tunnel: [w922 w928 w936 w944 w952 w961 w968 w977] -> w917
            tunnel: [w924 w930 w938 w945 w954 w963 w970 w979] -> w915
            tunnel: [w923 w929 w937 w946 w953 w962 w969 w978] -> w914
            tunnel: w918 -> [w926 w931 w939 w947 w955 w960 w971 w976]
            tunnel: w916 -> [w919 w927 w935 w943 w951 w959 w967 w975]
            frame 0, Default {
              n122 = Index Array(array=w919, index (row) #1=w926, index (col) #1=0, index (row) #2=w926, index (col) #2=1, index (row) #3=w926, index (col) #3=2) -> (element #1=w924:dbl, element #2=w923:dbl, element #3=w922:dbl)
            }
            frame 1 {
              n123 = Index Array(array=w927, index (row) #1=w931, index (col) #1=0, index (row) #2=w931, index (col) #2=1, index (row) #3=w931, index (col) #3=2) -> (element #1=w930:dbl, element #2=w929:dbl, element #3=w928:dbl)
            }
            frame 2 {
              n124 = Index Array(array=w935, index (row) #1=w939, index (col) #1=0, index (row) #2=w939, index (col) #2=1, index (row) #3=w939, index (col) #3=2) -> (element #1=w938:dbl, element #2=w937:dbl, element #3=w936:dbl)
            }
            frame 3 {
              n125 = Index Array(array=w943, index (row) #1=w947, index (col) #1=0, index (row) #2=w947, index (col) #2=1, index (row) #3=w947, index (col) #3=2) -> (element #1=w945:dbl, element #2=w946:dbl, element #3=w944:dbl)
            }
            frame 4 {
              n126 = Index Array(array=w951, index (row) #1=w955, index (col) #1=0, index (row) #2=w955, index (col) #2=1, index (row) #3=w955, index (col) #3=2) -> (element #1=w952:dbl, element #2=w954:dbl, element #3=w953:dbl)
            }
            frame 5 {
              n127 = Index Array(array=w959, index (row) #1=w960, index (col) #1=0, index (row) #2=w960, index (col) #2=1, index (row) #3=w960, index (col) #3=2) -> (element #1=w961:dbl, element #2=w962:dbl, element #3=w963:dbl)
            }
            frame 6 {
              n128 = Index Array(array=w967, index (row) #1=w971, index (col) #1=0, index (row) #2=w971, index (col) #2=1, index (row) #3=w971, index (col) #3=2) -> (element #1=w968:dbl, element #2=w970:dbl, element #3=w969:dbl)
            }
            frame 7 {
              n129 = Index Array(array=w975, index (row) #1=w976, index (col) #1=0, index (row) #2=w976, index (col) #2=1, index (row) #3=w976, index (col) #3=2) -> (element #1=w977:dbl, element #2=w979:dbl, element #3=w978:dbl)
            }
          }
        }
        frame "South west" {
          w987 = 7
          n130 = case shown="2" w987 {
            tunnel: [w991 w997 w1005 w1013 w1021 w1030 w1037 w1046] -> w985
            tunnel: [w993 w999 w1007 w1014 w1023 w1032 w1039 w1048] -> w984
            tunnel: [w992 w998 w1006 w1015 w1022 w1031 w1038 w1047] -> w983
            tunnel: w987 -> [w995 w1000 w1008 w1016 w1024 w1029 w1040 w1045]
            tunnel: w986 -> [w988 w996 w1004 w1012 w1020 w1028 w1036 w1044]
            frame 0, Default {
              n131 = Index Array(array=w988, index (row) #1=w995, index (col) #1=0, index (row) #2=w995, index (col) #2=1, index (row) #3=w995, index (col) #3=2) -> (element #1=w993:dbl, element #2=w992:dbl, element #3=w991:dbl)
            }
            frame 1 {
              n132 = Index Array(array=w996, index (row) #1=w1000, index (col) #1=0, index (row) #2=w1000, index (col) #2=1, index (row) #3=w1000, index (col) #3=2) -> (element #1=w999:dbl, element #2=w998:dbl, element #3=w997:dbl)
            }
            frame 2 {
              n133 = Index Array(array=w1004, index (row) #1=w1008, index (col) #1=0, index (row) #2=w1008, index (col) #2=1, index (row) #3=w1008, index (col) #3=2) -> (element #1=w1007:dbl, element #2=w1006:dbl, element #3=w1005:dbl)
            }
            frame 3 {
              n134 = Index Array(array=w1012, index (row) #1=w1016, index (col) #1=0, index (row) #2=w1016, index (col) #2=1, index (row) #3=w1016, index (col) #3=2) -> (element #1=w1014:dbl, element #2=w1015:dbl, element #3=w1013:dbl)
            }
            frame 4 {
              n135 = Index Array(array=w1020, index (row) #1=w1024, index (col) #1=0, index (row) #2=w1024, index (col) #2=1, index (row) #3=w1024, index (col) #3=2) -> (element #1=w1021:dbl, element #2=w1023:dbl, element #3=w1022:dbl)
            }
            frame 5 {
              n136 = Index Array(array=w1028, index (row) #1=w1029, index (col) #1=0, index (row) #2=w1029, index (col) #2=1, index (row) #3=w1029, index (col) #3=2) -> (element #1=w1030:dbl, element #2=w1031:dbl, element #3=w1032:dbl)
            }
            frame 6 {
              n137 = Index Array(array=w1036, index (row) #1=w1040, index (col) #1=0, index (row) #2=w1040, index (col) #2=1, index (row) #3=w1040, index (col) #3=2) -> (element #1=w1037:dbl, element #2=w1039:dbl, element #3=w1038:dbl)
            }
            frame 7 {
              n138 = Index Array(array=w1044, index (row) #1=w1045, index (col) #1=0, index (row) #2=w1045, index (col) #2=1, index (row) #3=w1045, index (col) #3=2) -> (element #1=w1046:dbl, element #2=w1048:dbl, element #3=w1047:dbl)
            }
          }
        }
        frame "South east" {
          w1056 = 3
          n139 = case shown="2" w1056 {
            tunnel: [w1060 w1066 w1074 w1082 w1090 w1099 w1106 w1115] -> w1055
            tunnel: [w1062 w1068 w1076 w1083 w1092 w1101 w1108 w1117] -> w1054
            tunnel: [w1061 w1067 w1075 w1084 w1091 w1100 w1107 w1116] -> w1053
            tunnel: w1056 -> [w1064 w1069 w1077 w1085 w1093 w1098 w1109 w1114]
            tunnel: w1052 -> [w1057 w1065 w1073 w1081 w1089 w1097 w1105 w1113]
            frame 0, Default {
              n140 = Index Array(array=w1057, index (row) #1=w1064, index (col) #1=0, index (row) #2=w1064, index (col) #2=1, index (row) #3=w1064, index (col) #3=2) -> (element #1=w1062:dbl, element #2=w1061:dbl, element #3=w1060:dbl)
            }
            frame 1 {
              n141 = Index Array(array=w1065, index (row) #1=w1069, index (col) #1=0, index (row) #2=w1069, index (col) #2=1, index (row) #3=w1069, index (col) #3=2) -> (element #1=w1068:dbl, element #2=w1067:dbl, element #3=w1066:dbl)
            }
            frame 2 {
              n142 = Index Array(array=w1073, index (row) #1=w1077, index (col) #1=0, index (row) #2=w1077, index (col) #2=1, index (row) #3=w1077, index (col) #3=2) -> (element #1=w1076:dbl, element #2=w1075:dbl, element #3=w1074:dbl)
            }
            frame 3 {
              n143 = Index Array(array=w1081, index (row) #1=w1085, index (col) #1=0, index (row) #2=w1085, index (col) #2=1, index (row) #3=w1085, index (col) #3=2) -> (element #1=w1083:dbl, element #2=w1084:dbl, element #3=w1082:dbl)
            }
            frame 4 {
              n144 = Index Array(array=w1089, index (row) #1=w1093, index (col) #1=0, index (row) #2=w1093, index (col) #2=1, index (row) #3=w1093, index (col) #3=2) -> (element #1=w1090:dbl, element #2=w1092:dbl, element #3=w1091:dbl)
            }
            frame 5 {
              n145 = Index Array(array=w1097, index (row) #1=w1098, index (col) #1=0, index (row) #2=w1098, index (col) #2=1, index (row) #3=w1098, index (col) #3=2) -> (element #1=w1099:dbl, element #2=w1100:dbl, element #3=w1101:dbl)
            }
            frame 6 {
              n146 = Index Array(array=w1105, index (row) #1=w1109, index (col) #1=0, index (row) #2=w1109, index (col) #2=1, index (row) #3=w1109, index (col) #3=2) -> (element #1=w1106:dbl, element #2=w1108:dbl, element #3=w1107:dbl)
            }
            frame 7 {
              n147 = Index Array(array=w1113, index (row) #1=w1114, index (col) #1=0, index (row) #2=w1114, index (col) #2=1, index (row) #3=w1114, index (col) #3=2) -> (element #1=w1115:dbl, element #2=w1117:dbl, element #3=w1116:dbl)
            }
          }
        }
      }
    }
    frame "North west" {
      n148 = case shown="\"South east\"" w1122 {
        tunnel: [w1129 w1199 w1267 w1334 w1404 w1474 w1542 w1612] -> w1125
        tunnel: [w1128 w1198 w1266 w1335 w1403 w1472 w1541 w1611] -> w1124
        tunnel: [w1127 w1197 w1265 w1333 w1402 w1471 w1540 w1610] -> w1123
        tunnel: w1121 -> [w1126 w1195 w1264 w1336 w1405 w1473 w1543 w1609]
        frame "North", Default {
          w1130 = 1
          n149 = case shown="2" w1130 {
            tunnel: [w1134 w1140 w1148 w1156 w1164 w1173 w1180 w1189] -> w1129
            tunnel: [w1136 w1142 w1150 w1157 w1166 w1175 w1182 w1191] -> w1128
            tunnel: [w1135 w1141 w1149 w1158 w1165 w1174 w1181 w1190] -> w1127
            tunnel: w1130 -> [w1138 w1143 w1151 w1159 w1167 w1172 w1183 w1188]
            tunnel: w1126 -> [w1131 w1139 w1147 w1155 w1163 w1171 w1179 w1187]
            frame 0, Default {
              n150 = Index Array(array=w1131, index (row) #1=w1138, index (col) #1=0, index (row) #2=w1138, index (col) #2=1, index (row) #3=w1138, index (col) #3=2) -> (element #1=w1136:dbl, element #2=w1135:dbl, element #3=w1134:dbl)
            }
            frame 1 {
              n151 = Index Array(array=w1139, index (row) #1=w1143, index (col) #1=0, index (row) #2=w1143, index (col) #2=1, index (row) #3=w1143, index (col) #3=2) -> (element #1=w1142:dbl, element #2=w1141:dbl, element #3=w1140:dbl)
            }
            frame 2 {
              n152 = Index Array(array=w1147, index (row) #1=w1151, index (col) #1=0, index (row) #2=w1151, index (col) #2=1, index (row) #3=w1151, index (col) #3=2) -> (element #1=w1150:dbl, element #2=w1149:dbl, element #3=w1148:dbl)
            }
            frame 3 {
              n153 = Index Array(array=w1155, index (row) #1=w1159, index (col) #1=0, index (row) #2=w1159, index (col) #2=1, index (row) #3=w1159, index (col) #3=2) -> (element #1=w1157:dbl, element #2=w1158:dbl, element #3=w1156:dbl)
            }
            frame 4 {
              n154 = Index Array(array=w1163, index (row) #1=w1167, index (col) #1=0, index (row) #2=w1167, index (col) #2=1, index (row) #3=w1167, index (col) #3=2) -> (element #1=w1164:dbl, element #2=w1166:dbl, element #3=w1165:dbl)
            }
            frame 5 {
              n155 = Index Array(array=w1171, index (row) #1=w1172, index (col) #1=0, index (row) #2=w1172, index (col) #2=1, index (row) #3=w1172, index (col) #3=2) -> (element #1=w1173:dbl, element #2=w1174:dbl, element #3=w1175:dbl)
            }
            frame 6 {
              n156 = Index Array(array=w1179, index (row) #1=w1183, index (col) #1=0, index (row) #2=w1183, index (col) #2=1, index (row) #3=w1183, index (col) #3=2) -> (element #1=w1180:dbl, element #2=w1182:dbl, element #3=w1181:dbl)
            }
            frame 7 {
              n157 = Index Array(array=w1187, index (row) #1=w1188, index (col) #1=0, index (row) #2=w1188, index (col) #2=1, index (row) #3=w1188, index (col) #3=2) -> (element #1=w1189:dbl, element #2=w1191:dbl, element #3=w1190:dbl)
            }
          }
        }
        frame "North east" {
          w1196 = 3
          n158 = case shown="2" w1196 {
            tunnel: [w1203 w1209 w1217 w1225 w1233 w1242 w1249 w1258] -> w1199
            tunnel: [w1205 w1211 w1219 w1226 w1235 w1244 w1251 w1260] -> w1198
            tunnel: [w1204 w1210 w1218 w1227 w1234 w1243 w1250 w1259] -> w1197
            tunnel: w1196 -> [w1207 w1212 w1220 w1228 w1236 w1241 w1252 w1257]
            tunnel: w1195 -> [w1200 w1208 w1216 w1224 w1232 w1240 w1248 w1256]
            frame 0, Default {
              n159 = Index Array(array=w1200, index (row) #1=w1207, index (col) #1=0, index (row) #2=w1207, index (col) #2=1, index (row) #3=w1207, index (col) #3=2) -> (element #1=w1205:dbl, element #2=w1204:dbl, element #3=w1203:dbl)
            }
            frame 1 {
              n160 = Index Array(array=w1208, index (row) #1=w1212, index (col) #1=0, index (row) #2=w1212, index (col) #2=1, index (row) #3=w1212, index (col) #3=2) -> (element #1=w1211:dbl, element #2=w1210:dbl, element #3=w1209:dbl)
            }
            frame 2 {
              n161 = Index Array(array=w1216, index (row) #1=w1220, index (col) #1=0, index (row) #2=w1220, index (col) #2=1, index (row) #3=w1220, index (col) #3=2) -> (element #1=w1219:dbl, element #2=w1218:dbl, element #3=w1217:dbl)
            }
            frame 3 {
              n162 = Index Array(array=w1224, index (row) #1=w1228, index (col) #1=0, index (row) #2=w1228, index (col) #2=1, index (row) #3=w1228, index (col) #3=2) -> (element #1=w1226:dbl, element #2=w1227:dbl, element #3=w1225:dbl)
            }
            frame 4 {
              n163 = Index Array(array=w1232, index (row) #1=w1236, index (col) #1=0, index (row) #2=w1236, index (col) #2=1, index (row) #3=w1236, index (col) #3=2) -> (element #1=w1233:dbl, element #2=w1235:dbl, element #3=w1234:dbl)
            }
            frame 5 {
              n164 = Index Array(array=w1240, index (row) #1=w1241, index (col) #1=0, index (row) #2=w1241, index (col) #2=1, index (row) #3=w1241, index (col) #3=2) -> (element #1=w1242:dbl, element #2=w1243:dbl, element #3=w1244:dbl)
            }
            frame 6 {
              n165 = Index Array(array=w1248, index (row) #1=w1252, index (col) #1=0, index (row) #2=w1252, index (col) #2=1, index (row) #3=w1252, index (col) #3=2) -> (element #1=w1249:dbl, element #2=w1251:dbl, element #3=w1250:dbl)
            }
            frame 7 {
              n166 = Index Array(array=w1256, index (row) #1=w1257, index (col) #1=0, index (row) #2=w1257, index (col) #2=1, index (row) #3=w1257, index (col) #3=2) -> (element #1=w1258:dbl, element #2=w1260:dbl, element #3=w1259:dbl)
            }
          }
        }
        frame "North west" {
          w1268 = 0
          n167 = case shown="2" w1268 {
            tunnel: [w1272 w1278 w1286 w1294 w1302 w1311 w1318 w1327] -> w1267
            tunnel: [w1274 w1280 w1288 w1295 w1304 w1313 w1320 w1329] -> w1266
            tunnel: [w1273 w1279 w1287 w1296 w1303 w1312 w1319 w1328] -> w1265
            tunnel: w1268 -> [w1276 w1281 w1289 w1297 w1305 w1310 w1321 w1326]
            tunnel: w1264 -> [w1269 w1277 w1285 w1293 w1301 w1309 w1317 w1325]
            frame 0, Default {
              n168 = Index Array(array=w1269, index (row) #1=w1276, index (col) #1=0, index (row) #2=w1276, index (col) #2=1, index (row) #3=w1276, index (col) #3=2) -> (element #1=w1274:dbl, element #2=w1273:dbl, element #3=w1272:dbl)
            }
            frame 1 {
              n169 = Index Array(array=w1277, index (row) #1=w1281, index (col) #1=0, index (row) #2=w1281, index (col) #2=1, index (row) #3=w1281, index (col) #3=2) -> (element #1=w1280:dbl, element #2=w1279:dbl, element #3=w1278:dbl)
            }
            frame 2 {
              n170 = Index Array(array=w1285, index (row) #1=w1289, index (col) #1=0, index (row) #2=w1289, index (col) #2=1, index (row) #3=w1289, index (col) #3=2) -> (element #1=w1288:dbl, element #2=w1287:dbl, element #3=w1286:dbl)
            }
            frame 3 {
              n171 = Index Array(array=w1293, index (row) #1=w1297, index (col) #1=0, index (row) #2=w1297, index (col) #2=1, index (row) #3=w1297, index (col) #3=2) -> (element #1=w1295:dbl, element #2=w1296:dbl, element #3=w1294:dbl)
            }
            frame 4 {
              n172 = Index Array(array=w1301, index (row) #1=w1305, index (col) #1=0, index (row) #2=w1305, index (col) #2=1, index (row) #3=w1305, index (col) #3=2) -> (element #1=w1302:dbl, element #2=w1304:dbl, element #3=w1303:dbl)
            }
            frame 5 {
              n173 = Index Array(array=w1309, index (row) #1=w1310, index (col) #1=0, index (row) #2=w1310, index (col) #2=1, index (row) #3=w1310, index (col) #3=2) -> (element #1=w1311:dbl, element #2=w1312:dbl, element #3=w1313:dbl)
            }
            frame 6 {
              n174 = Index Array(array=w1317, index (row) #1=w1321, index (col) #1=0, index (row) #2=w1321, index (col) #2=1, index (row) #3=w1321, index (col) #3=2) -> (element #1=w1318:dbl, element #2=w1320:dbl, element #3=w1319:dbl)
            }
            frame 7 {
              n175 = Index Array(array=w1325, index (row) #1=w1326, index (col) #1=0, index (row) #2=w1326, index (col) #2=1, index (row) #3=w1326, index (col) #3=2) -> (element #1=w1327:dbl, element #2=w1329:dbl, element #3=w1328:dbl)
            }
          }
        }
        frame "West" {
          w1337 = 2
          n176 = case shown="2" w1337 {
            tunnel: [w1341 w1347 w1355 w1363 w1371 w1380 w1387 w1396] -> w1334
            tunnel: [w1343 w1349 w1357 w1364 w1373 w1382 w1389 w1398] -> w1335
            tunnel: [w1342 w1348 w1356 w1365 w1372 w1381 w1388 w1397] -> w1333
            tunnel: w1337 -> [w1345 w1350 w1358 w1366 w1374 w1379 w1390 w1395]
            tunnel: w1336 -> [w1338 w1346 w1354 w1362 w1370 w1378 w1386 w1394]
            frame 0, Default {
              n177 = Index Array(array=w1338, index (row) #1=w1345, index (col) #1=0, index (row) #2=w1345, index (col) #2=1, index (row) #3=w1345, index (col) #3=2) -> (element #1=w1343:dbl, element #2=w1342:dbl, element #3=w1341:dbl)
            }
            frame 1 {
              n178 = Index Array(array=w1346, index (row) #1=w1350, index (col) #1=0, index (row) #2=w1350, index (col) #2=1, index (row) #3=w1350, index (col) #3=2) -> (element #1=w1349:dbl, element #2=w1348:dbl, element #3=w1347:dbl)
            }
            frame 2 {
              n179 = Index Array(array=w1354, index (row) #1=w1358, index (col) #1=0, index (row) #2=w1358, index (col) #2=1, index (row) #3=w1358, index (col) #3=2) -> (element #1=w1357:dbl, element #2=w1356:dbl, element #3=w1355:dbl)
            }
            frame 3 {
              n180 = Index Array(array=w1362, index (row) #1=w1366, index (col) #1=0, index (row) #2=w1366, index (col) #2=1, index (row) #3=w1366, index (col) #3=2) -> (element #1=w1364:dbl, element #2=w1365:dbl, element #3=w1363:dbl)
            }
            frame 4 {
              n181 = Index Array(array=w1370, index (row) #1=w1374, index (col) #1=0, index (row) #2=w1374, index (col) #2=1, index (row) #3=w1374, index (col) #3=2) -> (element #1=w1371:dbl, element #2=w1373:dbl, element #3=w1372:dbl)
            }
            frame 5 {
              n182 = Index Array(array=w1378, index (row) #1=w1379, index (col) #1=0, index (row) #2=w1379, index (col) #2=1, index (row) #3=w1379, index (col) #3=2) -> (element #1=w1380:dbl, element #2=w1381:dbl, element #3=w1382:dbl)
            }
            frame 6 {
              n183 = Index Array(array=w1386, index (row) #1=w1390, index (col) #1=0, index (row) #2=w1390, index (col) #2=1, index (row) #3=w1390, index (col) #3=2) -> (element #1=w1387:dbl, element #2=w1389:dbl, element #3=w1388:dbl)
            }
            frame 7 {
              n184 = Index Array(array=w1394, index (row) #1=w1395, index (col) #1=0, index (row) #2=w1395, index (col) #2=1, index (row) #3=w1395, index (col) #3=2) -> (element #1=w1396:dbl, element #2=w1398:dbl, element #3=w1397:dbl)
            }
          }
        }
        frame "East" {
          w1406 = 5
          n185 = case shown="2" w1406 {
            tunnel: [w1410 w1416 w1424 w1432 w1440 w1449 w1456 w1465] -> w1404
            tunnel: [w1412 w1418 w1426 w1433 w1442 w1451 w1458 w1467] -> w1403
            tunnel: [w1411 w1417 w1425 w1434 w1441 w1450 w1457 w1466] -> w1402
            tunnel: w1406 -> [w1414 w1419 w1427 w1435 w1443 w1448 w1459 w1464]
            tunnel: w1405 -> [w1407 w1415 w1423 w1431 w1439 w1447 w1455 w1463]
            frame 0, Default {
              n186 = Index Array(array=w1407, index (row) #1=w1414, index (col) #1=0, index (row) #2=w1414, index (col) #2=1, index (row) #3=w1414, index (col) #3=2) -> (element #1=w1412:dbl, element #2=w1411:dbl, element #3=w1410:dbl)
            }
            frame 1 {
              n187 = Index Array(array=w1415, index (row) #1=w1419, index (col) #1=0, index (row) #2=w1419, index (col) #2=1, index (row) #3=w1419, index (col) #3=2) -> (element #1=w1418:dbl, element #2=w1417:dbl, element #3=w1416:dbl)
            }
            frame 2 {
              n188 = Index Array(array=w1423, index (row) #1=w1427, index (col) #1=0, index (row) #2=w1427, index (col) #2=1, index (row) #3=w1427, index (col) #3=2) -> (element #1=w1426:dbl, element #2=w1425:dbl, element #3=w1424:dbl)
            }
            frame 3 {
              n189 = Index Array(array=w1431, index (row) #1=w1435, index (col) #1=0, index (row) #2=w1435, index (col) #2=1, index (row) #3=w1435, index (col) #3=2) -> (element #1=w1433:dbl, element #2=w1434:dbl, element #3=w1432:dbl)
            }
            frame 4 {
              n190 = Index Array(array=w1439, index (row) #1=w1443, index (col) #1=0, index (row) #2=w1443, index (col) #2=1, index (row) #3=w1443, index (col) #3=2) -> (element #1=w1440:dbl, element #2=w1442:dbl, element #3=w1441:dbl)
            }
            frame 5 {
              n191 = Index Array(array=w1447, index (row) #1=w1448, index (col) #1=0, index (row) #2=w1448, index (col) #2=1, index (row) #3=w1448, index (col) #3=2) -> (element #1=w1449:dbl, element #2=w1450:dbl, element #3=w1451:dbl)
            }
            frame 6 {
              n192 = Index Array(array=w1455, index (row) #1=w1459, index (col) #1=0, index (row) #2=w1459, index (col) #2=1, index (row) #3=w1459, index (col) #3=2) -> (element #1=w1456:dbl, element #2=w1458:dbl, element #3=w1457:dbl)
            }
            frame 7 {
              n193 = Index Array(array=w1463, index (row) #1=w1464, index (col) #1=0, index (row) #2=w1464, index (col) #2=1, index (row) #3=w1464, index (col) #3=2) -> (element #1=w1465:dbl, element #2=w1467:dbl, element #3=w1466:dbl)
            }
          }
        }
        frame "South" {
          w1475 = 6
          n194 = case shown="2" w1475 {
            tunnel: [w1479 w1485 w1493 w1501 w1509 w1518 w1525 w1534] -> w1474
            tunnel: [w1481 w1487 w1495 w1502 w1511 w1520 w1527 w1536] -> w1472
            tunnel: [w1480 w1486 w1494 w1503 w1510 w1519 w1526 w1535] -> w1471
            tunnel: w1475 -> [w1483 w1488 w1496 w1504 w1512 w1517 w1528 w1533]
            tunnel: w1473 -> [w1476 w1484 w1492 w1500 w1508 w1516 w1524 w1532]
            frame 0, Default {
              n195 = Index Array(array=w1476, index (row) #1=w1483, index (col) #1=0, index (row) #2=w1483, index (col) #2=1, index (row) #3=w1483, index (col) #3=2) -> (element #1=w1481:dbl, element #2=w1480:dbl, element #3=w1479:dbl)
            }
            frame 1 {
              n196 = Index Array(array=w1484, index (row) #1=w1488, index (col) #1=0, index (row) #2=w1488, index (col) #2=1, index (row) #3=w1488, index (col) #3=2) -> (element #1=w1487:dbl, element #2=w1486:dbl, element #3=w1485:dbl)
            }
            frame 2 {
              n197 = Index Array(array=w1492, index (row) #1=w1496, index (col) #1=0, index (row) #2=w1496, index (col) #2=1, index (row) #3=w1496, index (col) #3=2) -> (element #1=w1495:dbl, element #2=w1494:dbl, element #3=w1493:dbl)
            }
            frame 3 {
              n198 = Index Array(array=w1500, index (row) #1=w1504, index (col) #1=0, index (row) #2=w1504, index (col) #2=1, index (row) #3=w1504, index (col) #3=2) -> (element #1=w1502:dbl, element #2=w1503:dbl, element #3=w1501:dbl)
            }
            frame 4 {
              n199 = Index Array(array=w1508, index (row) #1=w1512, index (col) #1=0, index (row) #2=w1512, index (col) #2=1, index (row) #3=w1512, index (col) #3=2) -> (element #1=w1509:dbl, element #2=w1511:dbl, element #3=w1510:dbl)
            }
            frame 5 {
              n200 = Index Array(array=w1516, index (row) #1=w1517, index (col) #1=0, index (row) #2=w1517, index (col) #2=1, index (row) #3=w1517, index (col) #3=2) -> (element #1=w1518:dbl, element #2=w1519:dbl, element #3=w1520:dbl)
            }
            frame 6 {
              n201 = Index Array(array=w1524, index (row) #1=w1528, index (col) #1=0, index (row) #2=w1528, index (col) #2=1, index (row) #3=w1528, index (col) #3=2) -> (element #1=w1525:dbl, element #2=w1527:dbl, element #3=w1526:dbl)
            }
            frame 7 {
              n202 = Index Array(array=w1532, index (row) #1=w1533, index (col) #1=0, index (row) #2=w1533, index (col) #2=1, index (row) #3=w1533, index (col) #3=2) -> (element #1=w1534:dbl, element #2=w1536:dbl, element #3=w1535:dbl)
            }
          }
        }
        frame "South west" {
          w1544 = 4
          n203 = case shown="2" w1544 {
            tunnel: [w1548 w1554 w1562 w1570 w1578 w1587 w1594 w1603] -> w1542
            tunnel: [w1550 w1556 w1564 w1571 w1580 w1589 w1596 w1605] -> w1541
            tunnel: [w1549 w1555 w1563 w1572 w1579 w1588 w1595 w1604] -> w1540
            tunnel: w1544 -> [w1552 w1557 w1565 w1573 w1581 w1586 w1597 w1602]
            tunnel: w1543 -> [w1545 w1553 w1561 w1569 w1577 w1585 w1593 w1601]
            frame 0, Default {
              n204 = Index Array(array=w1545, index (row) #1=w1552, index (col) #1=0, index (row) #2=w1552, index (col) #2=1, index (row) #3=w1552, index (col) #3=2) -> (element #1=w1550:dbl, element #2=w1549:dbl, element #3=w1548:dbl)
            }
            frame 1 {
              n205 = Index Array(array=w1553, index (row) #1=w1557, index (col) #1=0, index (row) #2=w1557, index (col) #2=1, index (row) #3=w1557, index (col) #3=2) -> (element #1=w1556:dbl, element #2=w1555:dbl, element #3=w1554:dbl)
            }
            frame 2 {
              n206 = Index Array(array=w1561, index (row) #1=w1565, index (col) #1=0, index (row) #2=w1565, index (col) #2=1, index (row) #3=w1565, index (col) #3=2) -> (element #1=w1564:dbl, element #2=w1563:dbl, element #3=w1562:dbl)
            }
            frame 3 {
              n207 = Index Array(array=w1569, index (row) #1=w1573, index (col) #1=0, index (row) #2=w1573, index (col) #2=1, index (row) #3=w1573, index (col) #3=2) -> (element #1=w1571:dbl, element #2=w1572:dbl, element #3=w1570:dbl)
            }
            frame 4 {
              n208 = Index Array(array=w1577, index (row) #1=w1581, index (col) #1=0, index (row) #2=w1581, index (col) #2=1, index (row) #3=w1581, index (col) #3=2) -> (element #1=w1578:dbl, element #2=w1580:dbl, element #3=w1579:dbl)
            }
            frame 5 {
              n209 = Index Array(array=w1585, index (row) #1=w1586, index (col) #1=0, index (row) #2=w1586, index (col) #2=1, index (row) #3=w1586, index (col) #3=2) -> (element #1=w1587:dbl, element #2=w1588:dbl, element #3=w1589:dbl)
            }
            frame 6 {
              n210 = Index Array(array=w1593, index (row) #1=w1597, index (col) #1=0, index (row) #2=w1597, index (col) #2=1, index (row) #3=w1597, index (col) #3=2) -> (element #1=w1594:dbl, element #2=w1596:dbl, element #3=w1595:dbl)
            }
            frame 7 {
              n211 = Index Array(array=w1601, index (row) #1=w1602, index (col) #1=0, index (row) #2=w1602, index (col) #2=1, index (row) #3=w1602, index (col) #3=2) -> (element #1=w1603:dbl, element #2=w1605:dbl, element #3=w1604:dbl)
            }
          }
        }
        frame "South east" {
          w1613 = 7
          n212 = case shown="2" w1613 {
            tunnel: [w1617 w1623 w1631 w1639 w1647 w1656 w1663 w1672] -> w1612
            tunnel: [w1619 w1625 w1633 w1640 w1649 w1658 w1665 w1674] -> w1611
            tunnel: [w1618 w1624 w1632 w1641 w1648 w1657 w1664 w1673] -> w1610
            tunnel: w1613 -> [w1621 w1626 w1634 w1642 w1650 w1655 w1666 w1671]
            tunnel: w1609 -> [w1614 w1622 w1630 w1638 w1646 w1654 w1662 w1670]
            frame 0, Default {
              n213 = Index Array(array=w1614, index (row) #1=w1621, index (col) #1=0, index (row) #2=w1621, index (col) #2=1, index (row) #3=w1621, index (col) #3=2) -> (element #1=w1619:dbl, element #2=w1618:dbl, element #3=w1617:dbl)
            }
            frame 1 {
              n214 = Index Array(array=w1622, index (row) #1=w1626, index (col) #1=0, index (row) #2=w1626, index (col) #2=1, index (row) #3=w1626, index (col) #3=2) -> (element #1=w1625:dbl, element #2=w1624:dbl, element #3=w1623:dbl)
            }
            frame 2 {
              n215 = Index Array(array=w1630, index (row) #1=w1634, index (col) #1=0, index (row) #2=w1634, index (col) #2=1, index (row) #3=w1634, index (col) #3=2) -> (element #1=w1633:dbl, element #2=w1632:dbl, element #3=w1631:dbl)
            }
            frame 3 {
              n216 = Index Array(array=w1638, index (row) #1=w1642, index (col) #1=0, index (row) #2=w1642, index (col) #2=1, index (row) #3=w1642, index (col) #3=2) -> (element #1=w1640:dbl, element #2=w1641:dbl, element #3=w1639:dbl)
            }
            frame 4 {
              n217 = Index Array(array=w1646, index (row) #1=w1650, index (col) #1=0, index (row) #2=w1650, index (col) #2=1, index (row) #3=w1650, index (col) #3=2) -> (element #1=w1647:dbl, element #2=w1649:dbl, element #3=w1648:dbl)
            }
            frame 5 {
              n218 = Index Array(array=w1654, index (row) #1=w1655, index (col) #1=0, index (row) #2=w1655, index (col) #2=1, index (row) #3=w1655, index (col) #3=2) -> (element #1=w1656:dbl, element #2=w1657:dbl, element #3=w1658:dbl)
            }
            frame 6 {
              n219 = Index Array(array=w1662, index (row) #1=w1666, index (col) #1=0, index (row) #2=w1666, index (col) #2=1, index (row) #3=w1666, index (col) #3=2) -> (element #1=w1663:dbl, element #2=w1665:dbl, element #3=w1664:dbl)
            }
            frame 7 {
              n220 = Index Array(array=w1670, index (row) #1=w1671, index (col) #1=0, index (row) #2=w1671, index (col) #2=1, index (row) #3=w1671, index (col) #3=2) -> (element #1=w1672:dbl, element #2=w1674:dbl, element #3=w1673:dbl)
            }
          }
        }
      }
    }
    frame "West" {
      n221 = case shown="\"North\", Default" w1679 {
        tunnel: [w1686 w1756 w1824 w1891 w1961 w2031 w2099 w2169] -> w1682
        tunnel: [w1685 w1755 w1823 w1892 w1960 w2029 w2098 w2168] -> w1681
        tunnel: [w1684 w1754 w1822 w1890 w1959 w2028 w2097 w2167] -> w1680
        tunnel: w1678 -> [w1683 w1752 w1821 w1893 w1962 w2030 w2100 w2166]
        frame "North", Default {
          w1687 = 3
          n222 = case shown="2" w1687 {
            tunnel: [w1691 w1697 w1705 w1713 w1721 w1730 w1737 w1746] -> w1686
            tunnel: [w1693 w1699 w1707 w1714 w1723 w1732 w1739 w1748] -> w1685
            tunnel: [w1692 w1698 w1706 w1715 w1722 w1731 w1738 w1747] -> w1684
            tunnel: w1687 -> [w1695 w1700 w1708 w1716 w1724 w1729 w1740 w1745]
            tunnel: w1683 -> [w1688 w1696 w1704 w1712 w1720 w1728 w1736 w1744]
            frame 0, Default {
              n223 = Index Array(array=w1688, index (row) #1=w1695, index (col) #1=0, index (row) #2=w1695, index (col) #2=1, index (row) #3=w1695, index (col) #3=2) -> (element #1=w1693:dbl, element #2=w1692:dbl, element #3=w1691:dbl)
            }
            frame 1 {
              n224 = Index Array(array=w1696, index (row) #1=w1700, index (col) #1=0, index (row) #2=w1700, index (col) #2=1, index (row) #3=w1700, index (col) #3=2) -> (element #1=w1699:dbl, element #2=w1698:dbl, element #3=w1697:dbl)
            }
            frame 2 {
              n225 = Index Array(array=w1704, index (row) #1=w1708, index (col) #1=0, index (row) #2=w1708, index (col) #2=1, index (row) #3=w1708, index (col) #3=2) -> (element #1=w1707:dbl, element #2=w1706:dbl, element #3=w1705:dbl)
            }
            frame 3 {
              n226 = Index Array(array=w1712, index (row) #1=w1716, index (col) #1=0, index (row) #2=w1716, index (col) #2=1, index (row) #3=w1716, index (col) #3=2) -> (element #1=w1714:dbl, element #2=w1715:dbl, element #3=w1713:dbl)
            }
            frame 4 {
              n227 = Index Array(array=w1720, index (row) #1=w1724, index (col) #1=0, index (row) #2=w1724, index (col) #2=1, index (row) #3=w1724, index (col) #3=2) -> (element #1=w1721:dbl, element #2=w1723:dbl, element #3=w1722:dbl)
            }
            frame 5 {
              n228 = Index Array(array=w1728, index (row) #1=w1729, index (col) #1=0, index (row) #2=w1729, index (col) #2=1, index (row) #3=w1729, index (col) #3=2) -> (element #1=w1730:dbl, element #2=w1731:dbl, element #3=w1732:dbl)
            }
            frame 6 {
              n229 = Index Array(array=w1736, index (row) #1=w1740, index (col) #1=0, index (row) #2=w1740, index (col) #2=1, index (row) #3=w1740, index (col) #3=2) -> (element #1=w1737:dbl, element #2=w1739:dbl, element #3=w1738:dbl)
            }
            frame 7 {
              n230 = Index Array(array=w1744, index (row) #1=w1745, index (col) #1=0, index (row) #2=w1745, index (col) #2=1, index (row) #3=w1745, index (col) #3=2) -> (element #1=w1746:dbl, element #2=w1748:dbl, element #3=w1747:dbl)
            }
          }
        }
        frame "North east" {
          w1753 = 5
          n231 = case shown="2" w1753 {
            tunnel: [w1760 w1766 w1774 w1782 w1790 w1799 w1806 w1815] -> w1756
            tunnel: [w1762 w1768 w1776 w1783 w1792 w1801 w1808 w1817] -> w1755
            tunnel: [w1761 w1767 w1775 w1784 w1791 w1800 w1807 w1816] -> w1754
            tunnel: w1753 -> [w1764 w1769 w1777 w1785 w1793 w1798 w1809 w1814]
            tunnel: w1752 -> [w1757 w1765 w1773 w1781 w1789 w1797 w1805 w1813]
            frame 0, Default {
              n232 = Index Array(array=w1757, index (row) #1=w1764, index (col) #1=0, index (row) #2=w1764, index (col) #2=1, index (row) #3=w1764, index (col) #3=2) -> (element #1=w1762:dbl, element #2=w1761:dbl, element #3=w1760:dbl)
            }
            frame 1 {
              n233 = Index Array(array=w1765, index (row) #1=w1769, index (col) #1=0, index (row) #2=w1769, index (col) #2=1, index (row) #3=w1769, index (col) #3=2) -> (element #1=w1768:dbl, element #2=w1767:dbl, element #3=w1766:dbl)
            }
            frame 2 {
              n234 = Index Array(array=w1773, index (row) #1=w1777, index (col) #1=0, index (row) #2=w1777, index (col) #2=1, index (row) #3=w1777, index (col) #3=2) -> (element #1=w1776:dbl, element #2=w1775:dbl, element #3=w1774:dbl)
            }
            frame 3 {
              n235 = Index Array(array=w1781, index (row) #1=w1785, index (col) #1=0, index (row) #2=w1785, index (col) #2=1, index (row) #3=w1785, index (col) #3=2) -> (element #1=w1783:dbl, element #2=w1784:dbl, element #3=w1782:dbl)
            }
            frame 4 {
              n236 = Index Array(array=w1789, index (row) #1=w1793, index (col) #1=0, index (row) #2=w1793, index (col) #2=1, index (row) #3=w1793, index (col) #3=2) -> (element #1=w1790:dbl, element #2=w1792:dbl, element #3=w1791:dbl)
            }
            frame 5 {
              n237 = Index Array(array=w1797, index (row) #1=w1798, index (col) #1=0, index (row) #2=w1798, index (col) #2=1, index (row) #3=w1798, index (col) #3=2) -> (element #1=w1799:dbl, element #2=w1800:dbl, element #3=w1801:dbl)
            }
            frame 6 {
              n238 = Index Array(array=w1805, index (row) #1=w1809, index (col) #1=0, index (row) #2=w1809, index (col) #2=1, index (row) #3=w1809, index (col) #3=2) -> (element #1=w1806:dbl, element #2=w1808:dbl, element #3=w1807:dbl)
            }
            frame 7 {
              n239 = Index Array(array=w1813, index (row) #1=w1814, index (col) #1=0, index (row) #2=w1814, index (col) #2=1, index (row) #3=w1814, index (col) #3=2) -> (element #1=w1815:dbl, element #2=w1817:dbl, element #3=w1816:dbl)
            }
          }
        }
        frame "North west" {
          w1825 = 1
          n240 = case shown="2" w1825 {
            tunnel: [w1829 w1835 w1843 w1851 w1859 w1868 w1875 w1884] -> w1824
            tunnel: [w1831 w1837 w1845 w1852 w1861 w1870 w1877 w1886] -> w1823
            tunnel: [w1830 w1836 w1844 w1853 w1860 w1869 w1876 w1885] -> w1822
            tunnel: w1825 -> [w1833 w1838 w1846 w1854 w1862 w1867 w1878 w1883]
            tunnel: w1821 -> [w1826 w1834 w1842 w1850 w1858 w1866 w1874 w1882]
            frame 0, Default {
              n241 = Index Array(array=w1826, index (row) #1=w1833, index (col) #1=0, index (row) #2=w1833, index (col) #2=1, index (row) #3=w1833, index (col) #3=2) -> (element #1=w1831:dbl, element #2=w1830:dbl, element #3=w1829:dbl)
            }
            frame 1 {
              n242 = Index Array(array=w1834, index (row) #1=w1838, index (col) #1=0, index (row) #2=w1838, index (col) #2=1, index (row) #3=w1838, index (col) #3=2) -> (element #1=w1837:dbl, element #2=w1836:dbl, element #3=w1835:dbl)
            }
            frame 2 {
              n243 = Index Array(array=w1842, index (row) #1=w1846, index (col) #1=0, index (row) #2=w1846, index (col) #2=1, index (row) #3=w1846, index (col) #3=2) -> (element #1=w1845:dbl, element #2=w1844:dbl, element #3=w1843:dbl)
            }
            frame 3 {
              n244 = Index Array(array=w1850, index (row) #1=w1854, index (col) #1=0, index (row) #2=w1854, index (col) #2=1, index (row) #3=w1854, index (col) #3=2) -> (element #1=w1852:dbl, element #2=w1853:dbl, element #3=w1851:dbl)
            }
            frame 4 {
              n245 = Index Array(array=w1858, index (row) #1=w1862, index (col) #1=0, index (row) #2=w1862, index (col) #2=1, index (row) #3=w1862, index (col) #3=2) -> (element #1=w1859:dbl, element #2=w1861:dbl, element #3=w1860:dbl)
            }
            frame 5 {
              n246 = Index Array(array=w1866, index (row) #1=w1867, index (col) #1=0, index (row) #2=w1867, index (col) #2=1, index (row) #3=w1867, index (col) #3=2) -> (element #1=w1868:dbl, element #2=w1869:dbl, element #3=w1870:dbl)
            }
            frame 6 {
              n247 = Index Array(array=w1874, index (row) #1=w1878, index (col) #1=0, index (row) #2=w1878, index (col) #2=1, index (row) #3=w1878, index (col) #3=2) -> (element #1=w1875:dbl, element #2=w1877:dbl, element #3=w1876:dbl)
            }
            frame 7 {
              n248 = Index Array(array=w1882, index (row) #1=w1883, index (col) #1=0, index (row) #2=w1883, index (col) #2=1, index (row) #3=w1883, index (col) #3=2) -> (element #1=w1884:dbl, element #2=w1886:dbl, element #3=w1885:dbl)
            }
          }
        }
        frame "West" {
          w1894 = 0
          n249 = case shown="2" w1894 {
            tunnel: [w1898 w1904 w1912 w1920 w1928 w1937 w1944 w1953] -> w1891
            tunnel: [w1900 w1906 w1914 w1921 w1930 w1939 w1946 w1955] -> w1892
            tunnel: [w1899 w1905 w1913 w1922 w1929 w1938 w1945 w1954] -> w1890
            tunnel: w1894 -> [w1902 w1907 w1915 w1923 w1931 w1936 w1947 w1952]
            tunnel: w1893 -> [w1895 w1903 w1911 w1919 w1927 w1935 w1943 w1951]
            frame 0, Default {
              n250 = Index Array(array=w1895, index (row) #1=w1902, index (col) #1=0, index (row) #2=w1902, index (col) #2=1, index (row) #3=w1902, index (col) #3=2) -> (element #1=w1900:dbl, element #2=w1899:dbl, element #3=w1898:dbl)
            }
            frame 1 {
              n251 = Index Array(array=w1903, index (row) #1=w1907, index (col) #1=0, index (row) #2=w1907, index (col) #2=1, index (row) #3=w1907, index (col) #3=2) -> (element #1=w1906:dbl, element #2=w1905:dbl, element #3=w1904:dbl)
            }
            frame 2 {
              n252 = Index Array(array=w1911, index (row) #1=w1915, index (col) #1=0, index (row) #2=w1915, index (col) #2=1, index (row) #3=w1915, index (col) #3=2) -> (element #1=w1914:dbl, element #2=w1913:dbl, element #3=w1912:dbl)
            }
            frame 3 {
              n253 = Index Array(array=w1919, index (row) #1=w1923, index (col) #1=0, index (row) #2=w1923, index (col) #2=1, index (row) #3=w1923, index (col) #3=2) -> (element #1=w1921:dbl, element #2=w1922:dbl, element #3=w1920:dbl)
            }
            frame 4 {
              n254 = Index Array(array=w1927, index (row) #1=w1931, index (col) #1=0, index (row) #2=w1931, index (col) #2=1, index (row) #3=w1931, index (col) #3=2) -> (element #1=w1928:dbl, element #2=w1930:dbl, element #3=w1929:dbl)
            }
            frame 5 {
              n255 = Index Array(array=w1935, index (row) #1=w1936, index (col) #1=0, index (row) #2=w1936, index (col) #2=1, index (row) #3=w1936, index (col) #3=2) -> (element #1=w1937:dbl, element #2=w1938:dbl, element #3=w1939:dbl)
            }
            frame 6 {
              n256 = Index Array(array=w1943, index (row) #1=w1947, index (col) #1=0, index (row) #2=w1947, index (col) #2=1, index (row) #3=w1947, index (col) #3=2) -> (element #1=w1944:dbl, element #2=w1946:dbl, element #3=w1945:dbl)
            }
            frame 7 {
              n257 = Index Array(array=w1951, index (row) #1=w1952, index (col) #1=0, index (row) #2=w1952, index (col) #2=1, index (row) #3=w1952, index (col) #3=2) -> (element #1=w1953:dbl, element #2=w1955:dbl, element #3=w1954:dbl)
            }
          }
        }
        frame "East" {
          w1963 = 7
          n258 = case shown="2" w1963 {
            tunnel: [w1967 w1973 w1981 w1989 w1997 w2006 w2013 w2022] -> w1961
            tunnel: [w1969 w1975 w1983 w1990 w1999 w2008 w2015 w2024] -> w1960
            tunnel: [w1968 w1974 w1982 w1991 w1998 w2007 w2014 w2023] -> w1959
            tunnel: w1963 -> [w1971 w1976 w1984 w1992 w2000 w2005 w2016 w2021]
            tunnel: w1962 -> [w1964 w1972 w1980 w1988 w1996 w2004 w2012 w2020]
            frame 0, Default {
              n259 = Index Array(array=w1964, index (row) #1=w1971, index (col) #1=0, index (row) #2=w1971, index (col) #2=1, index (row) #3=w1971, index (col) #3=2) -> (element #1=w1969:dbl, element #2=w1968:dbl, element #3=w1967:dbl)
            }
            frame 1 {
              n260 = Index Array(array=w1972, index (row) #1=w1976, index (col) #1=0, index (row) #2=w1976, index (col) #2=1, index (row) #3=w1976, index (col) #3=2) -> (element #1=w1975:dbl, element #2=w1974:dbl, element #3=w1973:dbl)
            }
            frame 2 {
              n261 = Index Array(array=w1980, index (row) #1=w1984, index (col) #1=0, index (row) #2=w1984, index (col) #2=1, index (row) #3=w1984, index (col) #3=2) -> (element #1=w1983:dbl, element #2=w1982:dbl, element #3=w1981:dbl)
            }
            frame 3 {
              n262 = Index Array(array=w1988, index (row) #1=w1992, index (col) #1=0, index (row) #2=w1992, index (col) #2=1, index (row) #3=w1992, index (col) #3=2) -> (element #1=w1990:dbl, element #2=w1991:dbl, element #3=w1989:dbl)
            }
            frame 4 {
              n263 = Index Array(array=w1996, index (row) #1=w2000, index (col) #1=0, index (row) #2=w2000, index (col) #2=1, index (row) #3=w2000, index (col) #3=2) -> (element #1=w1997:dbl, element #2=w1999:dbl, element #3=w1998:dbl)
            }
            frame 5 {
              n264 = Index Array(array=w2004, index (row) #1=w2005, index (col) #1=0, index (row) #2=w2005, index (col) #2=1, index (row) #3=w2005, index (col) #3=2) -> (element #1=w2006:dbl, element #2=w2007:dbl, element #3=w2008:dbl)
            }
            frame 6 {
              n265 = Index Array(array=w2012, index (row) #1=w2016, index (col) #1=0, index (row) #2=w2016, index (col) #2=1, index (row) #3=w2016, index (col) #3=2) -> (element #1=w2013:dbl, element #2=w2015:dbl, element #3=w2014:dbl)
            }
            frame 7 {
              n266 = Index Array(array=w2020, index (row) #1=w2021, index (col) #1=0, index (row) #2=w2021, index (col) #2=1, index (row) #3=w2021, index (col) #3=2) -> (element #1=w2022:dbl, element #2=w2024:dbl, element #3=w2023:dbl)
            }
          }
        }
        frame "South" {
          w2032 = 4
          n267 = case shown="2" w2032 {
            tunnel: [w2036 w2042 w2050 w2058 w2066 w2075 w2082 w2091] -> w2031
            tunnel: [w2038 w2044 w2052 w2059 w2068 w2077 w2084 w2093] -> w2029
            tunnel: [w2037 w2043 w2051 w2060 w2067 w2076 w2083 w2092] -> w2028
            tunnel: w2032 -> [w2040 w2045 w2053 w2061 w2069 w2074 w2085 w2090]
            tunnel: w2030 -> [w2033 w2041 w2049 w2057 w2065 w2073 w2081 w2089]
            frame 0, Default {
              n268 = Index Array(array=w2033, index (row) #1=w2040, index (col) #1=0, index (row) #2=w2040, index (col) #2=1, index (row) #3=w2040, index (col) #3=2) -> (element #1=w2038:dbl, element #2=w2037:dbl, element #3=w2036:dbl)
            }
            frame 1 {
              n269 = Index Array(array=w2041, index (row) #1=w2045, index (col) #1=0, index (row) #2=w2045, index (col) #2=1, index (row) #3=w2045, index (col) #3=2) -> (element #1=w2044:dbl, element #2=w2043:dbl, element #3=w2042:dbl)
            }
            frame 2 {
              n270 = Index Array(array=w2049, index (row) #1=w2053, index (col) #1=0, index (row) #2=w2053, index (col) #2=1, index (row) #3=w2053, index (col) #3=2) -> (element #1=w2052:dbl, element #2=w2051:dbl, element #3=w2050:dbl)
            }
            frame 3 {
              n271 = Index Array(array=w2057, index (row) #1=w2061, index (col) #1=0, index (row) #2=w2061, index (col) #2=1, index (row) #3=w2061, index (col) #3=2) -> (element #1=w2059:dbl, element #2=w2060:dbl, element #3=w2058:dbl)
            }
            frame 4 {
              n272 = Index Array(array=w2065, index (row) #1=w2069, index (col) #1=0, index (row) #2=w2069, index (col) #2=1, index (row) #3=w2069, index (col) #3=2) -> (element #1=w2066:dbl, element #2=w2068:dbl, element #3=w2067:dbl)
            }
            frame 5 {
              n273 = Index Array(array=w2073, index (row) #1=w2074, index (col) #1=0, index (row) #2=w2074, index (col) #2=1, index (row) #3=w2074, index (col) #3=2) -> (element #1=w2075:dbl, element #2=w2076:dbl, element #3=w2077:dbl)
            }
            frame 6 {
              n274 = Index Array(array=w2081, index (row) #1=w2085, index (col) #1=0, index (row) #2=w2085, index (col) #2=1, index (row) #3=w2085, index (col) #3=2) -> (element #1=w2082:dbl, element #2=w2084:dbl, element #3=w2083:dbl)
            }
            frame 7 {
              n275 = Index Array(array=w2089, index (row) #1=w2090, index (col) #1=0, index (row) #2=w2090, index (col) #2=1, index (row) #3=w2090, index (col) #3=2) -> (element #1=w2091:dbl, element #2=w2093:dbl, element #3=w2092:dbl)
            }
          }
        }
        frame "South west" {
          w2101 = 2
          n276 = case shown="2" w2101 {
            tunnel: [w2105 w2111 w2119 w2127 w2135 w2144 w2151 w2160] -> w2099
            tunnel: [w2107 w2113 w2121 w2128 w2137 w2146 w2153 w2162] -> w2098
            tunnel: [w2106 w2112 w2120 w2129 w2136 w2145 w2152 w2161] -> w2097
            tunnel: w2101 -> [w2109 w2114 w2122 w2130 w2138 w2143 w2154 w2159]
            tunnel: w2100 -> [w2102 w2110 w2118 w2126 w2134 w2142 w2150 w2158]
            frame 0, Default {
              n277 = Index Array(array=w2102, index (row) #1=w2109, index (col) #1=0, index (row) #2=w2109, index (col) #2=1, index (row) #3=w2109, index (col) #3=2) -> (element #1=w2107:dbl, element #2=w2106:dbl, element #3=w2105:dbl)
            }
            frame 1 {
              n278 = Index Array(array=w2110, index (row) #1=w2114, index (col) #1=0, index (row) #2=w2114, index (col) #2=1, index (row) #3=w2114, index (col) #3=2) -> (element #1=w2113:dbl, element #2=w2112:dbl, element #3=w2111:dbl)
            }
            frame 2 {
              n279 = Index Array(array=w2118, index (row) #1=w2122, index (col) #1=0, index (row) #2=w2122, index (col) #2=1, index (row) #3=w2122, index (col) #3=2) -> (element #1=w2121:dbl, element #2=w2120:dbl, element #3=w2119:dbl)
            }
            frame 3 {
              n280 = Index Array(array=w2126, index (row) #1=w2130, index (col) #1=0, index (row) #2=w2130, index (col) #2=1, index (row) #3=w2130, index (col) #3=2) -> (element #1=w2128:dbl, element #2=w2129:dbl, element #3=w2127:dbl)
            }
            frame 4 {
              n281 = Index Array(array=w2134, index (row) #1=w2138, index (col) #1=0, index (row) #2=w2138, index (col) #2=1, index (row) #3=w2138, index (col) #3=2) -> (element #1=w2135:dbl, element #2=w2137:dbl, element #3=w2136:dbl)
            }
            frame 5 {
              n282 = Index Array(array=w2142, index (row) #1=w2143, index (col) #1=0, index (row) #2=w2143, index (col) #2=1, index (row) #3=w2143, index (col) #3=2) -> (element #1=w2144:dbl, element #2=w2145:dbl, element #3=w2146:dbl)
            }
            frame 6 {
              n283 = Index Array(array=w2150, index (row) #1=w2154, index (col) #1=0, index (row) #2=w2154, index (col) #2=1, index (row) #3=w2154, index (col) #3=2) -> (element #1=w2151:dbl, element #2=w2153:dbl, element #3=w2152:dbl)
            }
            frame 7 {
              n284 = Index Array(array=w2158, index (row) #1=w2159, index (col) #1=0, index (row) #2=w2159, index (col) #2=1, index (row) #3=w2159, index (col) #3=2) -> (element #1=w2160:dbl, element #2=w2162:dbl, element #3=w2161:dbl)
            }
          }
        }
        frame "South east" {
          w2170 = 6
          n285 = case shown="2" w2170 {
            tunnel: [w2174 w2180 w2188 w2196 w2204 w2213 w2220 w2229] -> w2169
            tunnel: [w2176 w2182 w2190 w2197 w2206 w2215 w2222 w2231] -> w2168
            tunnel: [w2175 w2181 w2189 w2198 w2205 w2214 w2221 w2230] -> w2167
            tunnel: w2170 -> [w2178 w2183 w2191 w2199 w2207 w2212 w2223 w2228]
            tunnel: w2166 -> [w2171 w2179 w2187 w2195 w2203 w2211 w2219 w2227]
            frame 0, Default {
              n286 = Index Array(array=w2171, index (row) #1=w2178, index (col) #1=0, index (row) #2=w2178, index (col) #2=1, index (row) #3=w2178, index (col) #3=2) -> (element #1=w2176:dbl, element #2=w2175:dbl, element #3=w2174:dbl)
            }
            frame 1 {
              n287 = Index Array(array=w2179, index (row) #1=w2183, index (col) #1=0, index (row) #2=w2183, index (col) #2=1, index (row) #3=w2183, index (col) #3=2) -> (element #1=w2182:dbl, element #2=w2181:dbl, element #3=w2180:dbl)
            }
            frame 2 {
              n288 = Index Array(array=w2187, index (row) #1=w2191, index (col) #1=0, index (row) #2=w2191, index (col) #2=1, index (row) #3=w2191, index (col) #3=2) -> (element #1=w2190:dbl, element #2=w2189:dbl, element #3=w2188:dbl)
            }
            frame 3 {
              n289 = Index Array(array=w2195, index (row) #1=w2199, index (col) #1=0, index (row) #2=w2199, index (col) #2=1, index (row) #3=w2199, index (col) #3=2) -> (element #1=w2197:dbl, element #2=w2198:dbl, element #3=w2196:dbl)
            }
            frame 4 {
              n290 = Index Array(array=w2203, index (row) #1=w2207, index (col) #1=0, index (row) #2=w2207, index (col) #2=1, index (row) #3=w2207, index (col) #3=2) -> (element #1=w2204:dbl, element #2=w2206:dbl, element #3=w2205:dbl)
            }
            frame 5 {
              n291 = Index Array(array=w2211, index (row) #1=w2212, index (col) #1=0, index (row) #2=w2212, index (col) #2=1, index (row) #3=w2212, index (col) #3=2) -> (element #1=w2213:dbl, element #2=w2214:dbl, element #3=w2215:dbl)
            }
            frame 6 {
              n292 = Index Array(array=w2219, index (row) #1=w2223, index (col) #1=0, index (row) #2=w2223, index (col) #2=1, index (row) #3=w2223, index (col) #3=2) -> (element #1=w2220:dbl, element #2=w2222:dbl, element #3=w2221:dbl)
            }
            frame 7 {
              n293 = Index Array(array=w2227, index (row) #1=w2228, index (col) #1=0, index (row) #2=w2228, index (col) #2=1, index (row) #3=w2228, index (col) #3=2) -> (element #1=w2229:dbl, element #2=w2231:dbl, element #3=w2230:dbl)
            }
          }
        }
      }
    }
    frame "East" {
      n294 = case shown="\"North\", Default" w2236 {
        tunnel: [w2243 w2313 w2381 w2448 w2518 w2588 w2656 w2726] -> w2239
        tunnel: [w2242 w2312 w2380 w2449 w2517 w2586 w2655 w2725] -> w2238
        tunnel: [w2241 w2311 w2379 w2447 w2516 w2585 w2654 w2724] -> w2237
        tunnel: w2235 -> [w2240 w2309 w2378 w2450 w2519 w2587 w2657 w2723]
        frame "North", Default {
          w2244 = 4
          n295 = case shown="2" w2244 {
            tunnel: [w2248 w2254 w2262 w2270 w2278 w2287 w2294 w2303] -> w2243
            tunnel: [w2250 w2256 w2264 w2271 w2280 w2289 w2296 w2305] -> w2242
            tunnel: [w2249 w2255 w2263 w2272 w2279 w2288 w2295 w2304] -> w2241
            tunnel: w2244 -> [w2252 w2257 w2265 w2273 w2281 w2286 w2297 w2302]
            tunnel: w2240 -> [w2245 w2253 w2261 w2269 w2277 w2285 w2293 w2301]
            frame 0, Default {
              n296 = Index Array(array=w2245, index (row) #1=w2252, index (col) #1=0, index (row) #2=w2252, index (col) #2=1, index (row) #3=w2252, index (col) #3=2) -> (element #1=w2250:dbl, element #2=w2249:dbl, element #3=w2248:dbl)
            }
            frame 1 {
              n297 = Index Array(array=w2253, index (row) #1=w2257, index (col) #1=0, index (row) #2=w2257, index (col) #2=1, index (row) #3=w2257, index (col) #3=2) -> (element #1=w2256:dbl, element #2=w2255:dbl, element #3=w2254:dbl)
            }
            frame 2 {
              n298 = Index Array(array=w2261, index (row) #1=w2265, index (col) #1=0, index (row) #2=w2265, index (col) #2=1, index (row) #3=w2265, index (col) #3=2) -> (element #1=w2264:dbl, element #2=w2263:dbl, element #3=w2262:dbl)
            }
            frame 3 {
              n299 = Index Array(array=w2269, index (row) #1=w2273, index (col) #1=0, index (row) #2=w2273, index (col) #2=1, index (row) #3=w2273, index (col) #3=2) -> (element #1=w2271:dbl, element #2=w2272:dbl, element #3=w2270:dbl)
            }
            frame 4 {
              n300 = Index Array(array=w2277, index (row) #1=w2281, index (col) #1=0, index (row) #2=w2281, index (col) #2=1, index (row) #3=w2281, index (col) #3=2) -> (element #1=w2278:dbl, element #2=w2280:dbl, element #3=w2279:dbl)
            }
            frame 5 {
              n301 = Index Array(array=w2285, index (row) #1=w2286, index (col) #1=0, index (row) #2=w2286, index (col) #2=1, index (row) #3=w2286, index (col) #3=2) -> (element #1=w2287:dbl, element #2=w2288:dbl, element #3=w2289:dbl)
            }
            frame 6 {
              n302 = Index Array(array=w2293, index (row) #1=w2297, index (col) #1=0, index (row) #2=w2297, index (col) #2=1, index (row) #3=w2297, index (col) #3=2) -> (element #1=w2294:dbl, element #2=w2296:dbl, element #3=w2295:dbl)
            }
            frame 7 {
              n303 = Index Array(array=w2301, index (row) #1=w2302, index (col) #1=0, index (row) #2=w2302, index (col) #2=1, index (row) #3=w2302, index (col) #3=2) -> (element #1=w2303:dbl, element #2=w2305:dbl, element #3=w2304:dbl)
            }
          }
        }
        frame "North east" {
          w2310 = 2
          n304 = case shown="2" w2310 {
            tunnel: [w2317 w2323 w2331 w2339 w2347 w2356 w2363 w2372] -> w2313
            tunnel: [w2319 w2325 w2333 w2340 w2349 w2358 w2365 w2374] -> w2312
            tunnel: [w2318 w2324 w2332 w2341 w2348 w2357 w2364 w2373] -> w2311
            tunnel: w2310 -> [w2321 w2326 w2334 w2342 w2350 w2355 w2366 w2371]
            tunnel: w2309 -> [w2314 w2322 w2330 w2338 w2346 w2354 w2362 w2370]
            frame 0, Default {
              n305 = Index Array(array=w2314, index (row) #1=w2321, index (col) #1=0, index (row) #2=w2321, index (col) #2=1, index (row) #3=w2321, index (col) #3=2) -> (element #1=w2319:dbl, element #2=w2318:dbl, element #3=w2317:dbl)
            }
            frame 1 {
              n306 = Index Array(array=w2322, index (row) #1=w2326, index (col) #1=0, index (row) #2=w2326, index (col) #2=1, index (row) #3=w2326, index (col) #3=2) -> (element #1=w2325:dbl, element #2=w2324:dbl, element #3=w2323:dbl)
            }
            frame 2 {
              n307 = Index Array(array=w2330, index (row) #1=w2334, index (col) #1=0, index (row) #2=w2334, index (col) #2=1, index (row) #3=w2334, index (col) #3=2) -> (element #1=w2333:dbl, element #2=w2332:dbl, element #3=w2331:dbl)
            }
            frame 3 {
              n308 = Index Array(array=w2338, index (row) #1=w2342, index (col) #1=0, index (row) #2=w2342, index (col) #2=1, index (row) #3=w2342, index (col) #3=2) -> (element #1=w2340:dbl, element #2=w2341:dbl, element #3=w2339:dbl)
            }
            frame 4 {
              n309 = Index Array(array=w2346, index (row) #1=w2350, index (col) #1=0, index (row) #2=w2350, index (col) #2=1, index (row) #3=w2350, index (col) #3=2) -> (element #1=w2347:dbl, element #2=w2349:dbl, element #3=w2348:dbl)
            }
            frame 5 {
              n310 = Index Array(array=w2354, index (row) #1=w2355, index (col) #1=0, index (row) #2=w2355, index (col) #2=1, index (row) #3=w2355, index (col) #3=2) -> (element #1=w2356:dbl, element #2=w2357:dbl, element #3=w2358:dbl)
            }
            frame 6 {
              n311 = Index Array(array=w2362, index (row) #1=w2366, index (col) #1=0, index (row) #2=w2366, index (col) #2=1, index (row) #3=w2366, index (col) #3=2) -> (element #1=w2363:dbl, element #2=w2365:dbl, element #3=w2364:dbl)
            }
            frame 7 {
              n312 = Index Array(array=w2370, index (row) #1=w2371, index (col) #1=0, index (row) #2=w2371, index (col) #2=1, index (row) #3=w2371, index (col) #3=2) -> (element #1=w2372:dbl, element #2=w2374:dbl, element #3=w2373:dbl)
            }
          }
        }
        frame "North west" {
          w2382 = 6
          n313 = case shown="2" w2382 {
            tunnel: [w2386 w2392 w2400 w2408 w2416 w2425 w2432 w2441] -> w2381
            tunnel: [w2388 w2394 w2402 w2409 w2418 w2427 w2434 w2443] -> w2380
            tunnel: [w2387 w2393 w2401 w2410 w2417 w2426 w2433 w2442] -> w2379
            tunnel: w2382 -> [w2390 w2395 w2403 w2411 w2419 w2424 w2435 w2440]
            tunnel: w2378 -> [w2383 w2391 w2399 w2407 w2415 w2423 w2431 w2439]
            frame 0, Default {
              n314 = Index Array(array=w2383, index (row) #1=w2390, index (col) #1=0, index (row) #2=w2390, index (col) #2=1, index (row) #3=w2390, index (col) #3=2) -> (element #1=w2388:dbl, element #2=w2387:dbl, element #3=w2386:dbl)
            }
            frame 1 {
              n315 = Index Array(array=w2391, index (row) #1=w2395, index (col) #1=0, index (row) #2=w2395, index (col) #2=1, index (row) #3=w2395, index (col) #3=2) -> (element #1=w2394:dbl, element #2=w2393:dbl, element #3=w2392:dbl)
            }
            frame 2 {
              n316 = Index Array(array=w2399, index (row) #1=w2403, index (col) #1=0, index (row) #2=w2403, index (col) #2=1, index (row) #3=w2403, index (col) #3=2) -> (element #1=w2402:dbl, element #2=w2401:dbl, element #3=w2400:dbl)
            }
            frame 3 {
              n317 = Index Array(array=w2407, index (row) #1=w2411, index (col) #1=0, index (row) #2=w2411, index (col) #2=1, index (row) #3=w2411, index (col) #3=2) -> (element #1=w2409:dbl, element #2=w2410:dbl, element #3=w2408:dbl)
            }
            frame 4 {
              n318 = Index Array(array=w2415, index (row) #1=w2419, index (col) #1=0, index (row) #2=w2419, index (col) #2=1, index (row) #3=w2419, index (col) #3=2) -> (element #1=w2416:dbl, element #2=w2418:dbl, element #3=w2417:dbl)
            }
            frame 5 {
              n319 = Index Array(array=w2423, index (row) #1=w2424, index (col) #1=0, index (row) #2=w2424, index (col) #2=1, index (row) #3=w2424, index (col) #3=2) -> (element #1=w2425:dbl, element #2=w2426:dbl, element #3=w2427:dbl)
            }
            frame 6 {
              n320 = Index Array(array=w2431, index (row) #1=w2435, index (col) #1=0, index (row) #2=w2435, index (col) #2=1, index (row) #3=w2435, index (col) #3=2) -> (element #1=w2432:dbl, element #2=w2434:dbl, element #3=w2433:dbl)
            }
            frame 7 {
              n321 = Index Array(array=w2439, index (row) #1=w2440, index (col) #1=0, index (row) #2=w2440, index (col) #2=1, index (row) #3=w2440, index (col) #3=2) -> (element #1=w2441:dbl, element #2=w2443:dbl, element #3=w2442:dbl)
            }
          }
        }
        frame "West" {
          w2451 = 7
          n322 = case shown="2" w2451 {
            tunnel: [w2455 w2461 w2469 w2477 w2485 w2494 w2501 w2510] -> w2448
            tunnel: [w2457 w2463 w2471 w2478 w2487 w2496 w2503 w2512] -> w2449
            tunnel: [w2456 w2462 w2470 w2479 w2486 w2495 w2502 w2511] -> w2447
            tunnel: w2451 -> [w2459 w2464 w2472 w2480 w2488 w2493 w2504 w2509]
            tunnel: w2450 -> [w2452 w2460 w2468 w2476 w2484 w2492 w2500 w2508]
            frame 0, Default {
              n323 = Index Array(array=w2452, index (row) #1=w2459, index (col) #1=0, index (row) #2=w2459, index (col) #2=1, index (row) #3=w2459, index (col) #3=2) -> (element #1=w2457:dbl, element #2=w2456:dbl, element #3=w2455:dbl)
            }
            frame 1 {
              n324 = Index Array(array=w2460, index (row) #1=w2464, index (col) #1=0, index (row) #2=w2464, index (col) #2=1, index (row) #3=w2464, index (col) #3=2) -> (element #1=w2463:dbl, element #2=w2462:dbl, element #3=w2461:dbl)
            }
            frame 2 {
              n325 = Index Array(array=w2468, index (row) #1=w2472, index (col) #1=0, index (row) #2=w2472, index (col) #2=1, index (row) #3=w2472, index (col) #3=2) -> (element #1=w2471:dbl, element #2=w2470:dbl, element #3=w2469:dbl)
            }
            frame 3 {
              n326 = Index Array(array=w2476, index (row) #1=w2480, index (col) #1=0, index (row) #2=w2480, index (col) #2=1, index (row) #3=w2480, index (col) #3=2) -> (element #1=w2478:dbl, element #2=w2479:dbl, element #3=w2477:dbl)
            }
            frame 4 {
              n327 = Index Array(array=w2484, index (row) #1=w2488, index (col) #1=0, index (row) #2=w2488, index (col) #2=1, index (row) #3=w2488, index (col) #3=2) -> (element #1=w2485:dbl, element #2=w2487:dbl, element #3=w2486:dbl)
            }
            frame 5 {
              n328 = Index Array(array=w2492, index (row) #1=w2493, index (col) #1=0, index (row) #2=w2493, index (col) #2=1, index (row) #3=w2493, index (col) #3=2) -> (element #1=w2494:dbl, element #2=w2495:dbl, element #3=w2496:dbl)
            }
            frame 6 {
              n329 = Index Array(array=w2500, index (row) #1=w2504, index (col) #1=0, index (row) #2=w2504, index (col) #2=1, index (row) #3=w2504, index (col) #3=2) -> (element #1=w2501:dbl, element #2=w2503:dbl, element #3=w2502:dbl)
            }
            frame 7 {
              n330 = Index Array(array=w2508, index (row) #1=w2509, index (col) #1=0, index (row) #2=w2509, index (col) #2=1, index (row) #3=w2509, index (col) #3=2) -> (element #1=w2510:dbl, element #2=w2512:dbl, element #3=w2511:dbl)
            }
          }
        }
        frame "East" {
          w2520 = 0
          n331 = case shown="2" w2520 {
            tunnel: [w2524 w2530 w2538 w2546 w2554 w2563 w2570 w2579] -> w2518
            tunnel: [w2526 w2532 w2540 w2547 w2556 w2565 w2572 w2581] -> w2517
            tunnel: [w2525 w2531 w2539 w2548 w2555 w2564 w2571 w2580] -> w2516
            tunnel: w2520 -> [w2528 w2533 w2541 w2549 w2557 w2562 w2573 w2578]
            tunnel: w2519 -> [w2521 w2529 w2537 w2545 w2553 w2561 w2569 w2577]
            frame 0, Default {
              n332 = Index Array(array=w2521, index (row) #1=w2528, index (col) #1=0, index (row) #2=w2528, index (col) #2=1, index (row) #3=w2528, index (col) #3=2) -> (element #1=w2526:dbl, element #2=w2525:dbl, element #3=w2524:dbl)
            }
            frame 1 {
              n333 = Index Array(array=w2529, index (row) #1=w2533, index (col) #1=0, index (row) #2=w2533, index (col) #2=1, index (row) #3=w2533, index (col) #3=2) -> (element #1=w2532:dbl, element #2=w2531:dbl, element #3=w2530:dbl)
            }
            frame 2 {
              n334 = Index Array(array=w2537, index (row) #1=w2541, index (col) #1=0, index (row) #2=w2541, index (col) #2=1, index (row) #3=w2541, index (col) #3=2) -> (element #1=w2540:dbl, element #2=w2539:dbl, element #3=w2538:dbl)
            }
            frame 3 {
              n335 = Index Array(array=w2545, index (row) #1=w2549, index (col) #1=0, index (row) #2=w2549, index (col) #2=1, index (row) #3=w2549, index (col) #3=2) -> (element #1=w2547:dbl, element #2=w2548:dbl, element #3=w2546:dbl)
            }
            frame 4 {
              n336 = Index Array(array=w2553, index (row) #1=w2557, index (col) #1=0, index (row) #2=w2557, index (col) #2=1, index (row) #3=w2557, index (col) #3=2) -> (element #1=w2554:dbl, element #2=w2556:dbl, element #3=w2555:dbl)
            }
            frame 5 {
              n337 = Index Array(array=w2561, index (row) #1=w2562, index (col) #1=0, index (row) #2=w2562, index (col) #2=1, index (row) #3=w2562, index (col) #3=2) -> (element #1=w2563:dbl, element #2=w2564:dbl, element #3=w2565:dbl)
            }
            frame 6 {
              n338 = Index Array(array=w2569, index (row) #1=w2573, index (col) #1=0, index (row) #2=w2573, index (col) #2=1, index (row) #3=w2573, index (col) #3=2) -> (element #1=w2570:dbl, element #2=w2572:dbl, element #3=w2571:dbl)
            }
            frame 7 {
              n339 = Index Array(array=w2577, index (row) #1=w2578, index (col) #1=0, index (row) #2=w2578, index (col) #2=1, index (row) #3=w2578, index (col) #3=2) -> (element #1=w2579:dbl, element #2=w2581:dbl, element #3=w2580:dbl)
            }
          }
        }
        frame "South" {
          w2589 = 3
          n340 = case shown="2" w2589 {
            tunnel: [w2593 w2599 w2607 w2615 w2623 w2632 w2639 w2648] -> w2588
            tunnel: [w2595 w2601 w2609 w2616 w2625 w2634 w2641 w2650] -> w2586
            tunnel: [w2594 w2600 w2608 w2617 w2624 w2633 w2640 w2649] -> w2585
            tunnel: w2589 -> [w2597 w2602 w2610 w2618 w2626 w2631 w2642 w2647]
            tunnel: w2587 -> [w2590 w2598 w2606 w2614 w2622 w2630 w2638 w2646]
            frame 0, Default {
              n341 = Index Array(array=w2590, index (row) #1=w2597, index (col) #1=0, index (row) #2=w2597, index (col) #2=1, index (row) #3=w2597, index (col) #3=2) -> (element #1=w2595:dbl, element #2=w2594:dbl, element #3=w2593:dbl)
            }
            frame 1 {
              n342 = Index Array(array=w2598, index (row) #1=w2602, index (col) #1=0, index (row) #2=w2602, index (col) #2=1, index (row) #3=w2602, index (col) #3=2) -> (element #1=w2601:dbl, element #2=w2600:dbl, element #3=w2599:dbl)
            }
            frame 2 {
              n343 = Index Array(array=w2606, index (row) #1=w2610, index (col) #1=0, index (row) #2=w2610, index (col) #2=1, index (row) #3=w2610, index (col) #3=2) -> (element #1=w2609:dbl, element #2=w2608:dbl, element #3=w2607:dbl)
            }
            frame 3 {
              n344 = Index Array(array=w2614, index (row) #1=w2618, index (col) #1=0, index (row) #2=w2618, index (col) #2=1, index (row) #3=w2618, index (col) #3=2) -> (element #1=w2616:dbl, element #2=w2617:dbl, element #3=w2615:dbl)
            }
            frame 4 {
              n345 = Index Array(array=w2622, index (row) #1=w2626, index (col) #1=0, index (row) #2=w2626, index (col) #2=1, index (row) #3=w2626, index (col) #3=2) -> (element #1=w2623:dbl, element #2=w2625:dbl, element #3=w2624:dbl)
            }
            frame 5 {
              n346 = Index Array(array=w2630, index (row) #1=w2631, index (col) #1=0, index (row) #2=w2631, index (col) #2=1, index (row) #3=w2631, index (col) #3=2) -> (element #1=w2632:dbl, element #2=w2633:dbl, element #3=w2634:dbl)
            }
            frame 6 {
              n347 = Index Array(array=w2638, index (row) #1=w2642, index (col) #1=0, index (row) #2=w2642, index (col) #2=1, index (row) #3=w2642, index (col) #3=2) -> (element #1=w2639:dbl, element #2=w2641:dbl, element #3=w2640:dbl)
            }
            frame 7 {
              n348 = Index Array(array=w2646, index (row) #1=w2647, index (col) #1=0, index (row) #2=w2647, index (col) #2=1, index (row) #3=w2647, index (col) #3=2) -> (element #1=w2648:dbl, element #2=w2650:dbl, element #3=w2649:dbl)
            }
          }
        }
        frame "South west" {
          w2658 = 5
          n349 = case shown="2" w2658 {
            tunnel: [w2662 w2668 w2676 w2684 w2692 w2701 w2708 w2717] -> w2656
            tunnel: [w2664 w2670 w2678 w2685 w2694 w2703 w2710 w2719] -> w2655
            tunnel: [w2663 w2669 w2677 w2686 w2693 w2702 w2709 w2718] -> w2654
            tunnel: w2658 -> [w2666 w2671 w2679 w2687 w2695 w2700 w2711 w2716]
            tunnel: w2657 -> [w2659 w2667 w2675 w2683 w2691 w2699 w2707 w2715]
            frame 0, Default {
              n350 = Index Array(array=w2659, index (row) #1=w2666, index (col) #1=0, index (row) #2=w2666, index (col) #2=1, index (row) #3=w2666, index (col) #3=2) -> (element #1=w2664:dbl, element #2=w2663:dbl, element #3=w2662:dbl)
            }
            frame 1 {
              n351 = Index Array(array=w2667, index (row) #1=w2671, index (col) #1=0, index (row) #2=w2671, index (col) #2=1, index (row) #3=w2671, index (col) #3=2) -> (element #1=w2670:dbl, element #2=w2669:dbl, element #3=w2668:dbl)
            }
            frame 2 {
              n352 = Index Array(array=w2675, index (row) #1=w2679, index (col) #1=0, index (row) #2=w2679, index (col) #2=1, index (row) #3=w2679, index (col) #3=2) -> (element #1=w2678:dbl, element #2=w2677:dbl, element #3=w2676:dbl)
            }
            frame 3 {
              n353 = Index Array(array=w2683, index (row) #1=w2687, index (col) #1=0, index (row) #2=w2687, index (col) #2=1, index (row) #3=w2687, index (col) #3=2) -> (element #1=w2685:dbl, element #2=w2686:dbl, element #3=w2684:dbl)
            }
            frame 4 {
              n354 = Index Array(array=w2691, index (row) #1=w2695, index (col) #1=0, index (row) #2=w2695, index (col) #2=1, index (row) #3=w2695, index (col) #3=2) -> (element #1=w2692:dbl, element #2=w2694:dbl, element #3=w2693:dbl)
            }
            frame 5 {
              n355 = Index Array(array=w2699, index (row) #1=w2700, index (col) #1=0, index (row) #2=w2700, index (col) #2=1, index (row) #3=w2700, index (col) #3=2) -> (element #1=w2701:dbl, element #2=w2702:dbl, element #3=w2703:dbl)
            }
            frame 6 {
              n356 = Index Array(array=w2707, index (row) #1=w2711, index (col) #1=0, index (row) #2=w2711, index (col) #2=1, index (row) #3=w2711, index (col) #3=2) -> (element #1=w2708:dbl, element #2=w2710:dbl, element #3=w2709:dbl)
            }
            frame 7 {
              n357 = Index Array(array=w2715, index (row) #1=w2716, index (col) #1=0, index (row) #2=w2716, index (col) #2=1, index (row) #3=w2716, index (col) #3=2) -> (element #1=w2717:dbl, element #2=w2719:dbl, element #3=w2718:dbl)
            }
          }
        }
        frame "South east" {
          w2727 = 1
          n358 = case shown="2" w2727 {
            tunnel: [w2731 w2737 w2745 w2753 w2761 w2770 w2777 w2786] -> w2726
            tunnel: [w2733 w2739 w2747 w2754 w2763 w2772 w2779 w2788] -> w2725
            tunnel: [w2732 w2738 w2746 w2755 w2762 w2771 w2778 w2787] -> w2724
            tunnel: w2727 -> [w2735 w2740 w2748 w2756 w2764 w2769 w2780 w2785]
            tunnel: w2723 -> [w2728 w2736 w2744 w2752 w2760 w2768 w2776 w2784]
            frame 0, Default {
              n359 = Index Array(array=w2728, index (row) #1=w2735, index (col) #1=0, index (row) #2=w2735, index (col) #2=1, index (row) #3=w2735, index (col) #3=2) -> (element #1=w2733:dbl, element #2=w2732:dbl, element #3=w2731:dbl)
            }
            frame 1 {
              n360 = Index Array(array=w2736, index (row) #1=w2740, index (col) #1=0, index (row) #2=w2740, index (col) #2=1, index (row) #3=w2740, index (col) #3=2) -> (element #1=w2739:dbl, element #2=w2738:dbl, element #3=w2737:dbl)
            }
            frame 2 {
              n361 = Index Array(array=w2744, index (row) #1=w2748, index (col) #1=0, index (row) #2=w2748, index (col) #2=1, index (row) #3=w2748, index (col) #3=2) -> (element #1=w2747:dbl, element #2=w2746:dbl, element #3=w2745:dbl)
            }
            frame 3 {
              n362 = Index Array(array=w2752, index (row) #1=w2756, index (col) #1=0, index (row) #2=w2756, index (col) #2=1, index (row) #3=w2756, index (col) #3=2) -> (element #1=w2754:dbl, element #2=w2755:dbl, element #3=w2753:dbl)
            }
            frame 4 {
              n363 = Index Array(array=w2760, index (row) #1=w2764, index (col) #1=0, index (row) #2=w2764, index (col) #2=1, index (row) #3=w2764, index (col) #3=2) -> (element #1=w2761:dbl, element #2=w2763:dbl, element #3=w2762:dbl)
            }
            frame 5 {
              n364 = Index Array(array=w2768, index (row) #1=w2769, index (col) #1=0, index (row) #2=w2769, index (col) #2=1, index (row) #3=w2769, index (col) #3=2) -> (element #1=w2770:dbl, element #2=w2771:dbl, element #3=w2772:dbl)
            }
            frame 6 {
              n365 = Index Array(array=w2776, index (row) #1=w2780, index (col) #1=0, index (row) #2=w2780, index (col) #2=1, index (row) #3=w2780, index (col) #3=2) -> (element #1=w2777:dbl, element #2=w2779:dbl, element #3=w2778:dbl)
            }
            frame 7 {
              n366 = Index Array(array=w2784, index (row) #1=w2785, index (col) #1=0, index (row) #2=w2785, index (col) #2=1, index (row) #3=w2785, index (col) #3=2) -> (element #1=w2786:dbl, element #2=w2788:dbl, element #3=w2787:dbl)
            }
          }
        }
      }
    }
    frame "South" {
      n367 = case shown="\"North\", Default" w2793 {
        tunnel: [w2800 w2870 w2938 w3005 w3075 w3145 w3213 w3283] -> w2796
        tunnel: [w2799 w2869 w2937 w3006 w3074 w3143 w3212 w3282] -> w2795
        tunnel: [w2798 w2868 w2936 w3004 w3073 w3142 w3211 w3281] -> w2794
        tunnel: w2792 -> [w2797 w2866 w2935 w3007 w3076 w3144 w3214 w3280]
        frame "North", Default {
          w2801 = 7
          n368 = case shown="2" w2801 {
            tunnel: [w2805 w2811 w2819 w2827 w2835 w2844 w2851 w2860] -> w2800
            tunnel: [w2807 w2813 w2821 w2828 w2837 w2846 w2853 w2862] -> w2799
            tunnel: [w2806 w2812 w2820 w2829 w2836 w2845 w2852 w2861] -> w2798
            tunnel: w2801 -> [w2809 w2814 w2822 w2830 w2838 w2843 w2854 w2859]
            tunnel: w2797 -> [w2802 w2810 w2818 w2826 w2834 w2842 w2850 w2858]
            frame 0, Default {
              n369 = Index Array(array=w2802, index (row) #1=w2809, index (col) #1=0, index (row) #2=w2809, index (col) #2=1, index (row) #3=w2809, index (col) #3=2) -> (element #1=w2807:dbl, element #2=w2806:dbl, element #3=w2805:dbl)
            }
            frame 1 {
              n370 = Index Array(array=w2810, index (row) #1=w2814, index (col) #1=0, index (row) #2=w2814, index (col) #2=1, index (row) #3=w2814, index (col) #3=2) -> (element #1=w2813:dbl, element #2=w2812:dbl, element #3=w2811:dbl)
            }
            frame 2 {
              n371 = Index Array(array=w2818, index (row) #1=w2822, index (col) #1=0, index (row) #2=w2822, index (col) #2=1, index (row) #3=w2822, index (col) #3=2) -> (element #1=w2821:dbl, element #2=w2820:dbl, element #3=w2819:dbl)
            }
            frame 3 {
              n372 = Index Array(array=w2826, index (row) #1=w2830, index (col) #1=0, index (row) #2=w2830, index (col) #2=1, index (row) #3=w2830, index (col) #3=2) -> (element #1=w2828:dbl, element #2=w2829:dbl, element #3=w2827:dbl)
            }
            frame 4 {
              n373 = Index Array(array=w2834, index (row) #1=w2838, index (col) #1=0, index (row) #2=w2838, index (col) #2=1, index (row) #3=w2838, index (col) #3=2) -> (element #1=w2835:dbl, element #2=w2837:dbl, element #3=w2836:dbl)
            }
            frame 5 {
              n374 = Index Array(array=w2842, index (row) #1=w2843, index (col) #1=0, index (row) #2=w2843, index (col) #2=1, index (row) #3=w2843, index (col) #3=2) -> (element #1=w2844:dbl, element #2=w2845:dbl, element #3=w2846:dbl)
            }
            frame 6 {
              n375 = Index Array(array=w2850, index (row) #1=w2854, index (col) #1=0, index (row) #2=w2854, index (col) #2=1, index (row) #3=w2854, index (col) #3=2) -> (element #1=w2851:dbl, element #2=w2853:dbl, element #3=w2852:dbl)
            }
            frame 7 {
              n376 = Index Array(array=w2858, index (row) #1=w2859, index (col) #1=0, index (row) #2=w2859, index (col) #2=1, index (row) #3=w2859, index (col) #3=2) -> (element #1=w2860:dbl, element #2=w2862:dbl, element #3=w2861:dbl)
            }
          }
        }
        frame "North east" {
          w2867 = 6
          n377 = case shown="2" w2867 {
            tunnel: [w2874 w2880 w2888 w2896 w2904 w2913 w2920 w2929] -> w2870
            tunnel: [w2876 w2882 w2890 w2897 w2906 w2915 w2922 w2931] -> w2869
            tunnel: [w2875 w2881 w2889 w2898 w2905 w2914 w2921 w2930] -> w2868
            tunnel: w2867 -> [w2878 w2883 w2891 w2899 w2907 w2912 w2923 w2928]
            tunnel: w2866 -> [w2871 w2879 w2887 w2895 w2903 w2911 w2919 w2927]
            frame 0, Default {
              n378 = Index Array(array=w2871, index (row) #1=w2878, index (col) #1=0, index (row) #2=w2878, index (col) #2=1, index (row) #3=w2878, index (col) #3=2) -> (element #1=w2876:dbl, element #2=w2875:dbl, element #3=w2874:dbl)
            }
            frame 1 {
              n379 = Index Array(array=w2879, index (row) #1=w2883, index (col) #1=0, index (row) #2=w2883, index (col) #2=1, index (row) #3=w2883, index (col) #3=2) -> (element #1=w2882:dbl, element #2=w2881:dbl, element #3=w2880:dbl)
            }
            frame 2 {
              n380 = Index Array(array=w2887, index (row) #1=w2891, index (col) #1=0, index (row) #2=w2891, index (col) #2=1, index (row) #3=w2891, index (col) #3=2) -> (element #1=w2890:dbl, element #2=w2889:dbl, element #3=w2888:dbl)
            }
            frame 3 {
              n381 = Index Array(array=w2895, index (row) #1=w2899, index (col) #1=0, index (row) #2=w2899, index (col) #2=1, index (row) #3=w2899, index (col) #3=2) -> (element #1=w2897:dbl, element #2=w2898:dbl, element #3=w2896:dbl)
            }
            frame 4 {
              n382 = Index Array(array=w2903, index (row) #1=w2907, index (col) #1=0, index (row) #2=w2907, index (col) #2=1, index (row) #3=w2907, index (col) #3=2) -> (element #1=w2904:dbl, element #2=w2906:dbl, element #3=w2905:dbl)
            }
            frame 5 {
              n383 = Index Array(array=w2911, index (row) #1=w2912, index (col) #1=0, index (row) #2=w2912, index (col) #2=1, index (row) #3=w2912, index (col) #3=2) -> (element #1=w2913:dbl, element #2=w2914:dbl, element #3=w2915:dbl)
            }
            frame 6 {
              n384 = Index Array(array=w2919, index (row) #1=w2923, index (col) #1=0, index (row) #2=w2923, index (col) #2=1, index (row) #3=w2923, index (col) #3=2) -> (element #1=w2920:dbl, element #2=w2922:dbl, element #3=w2921:dbl)
            }
            frame 7 {
              n385 = Index Array(array=w2927, index (row) #1=w2928, index (col) #1=0, index (row) #2=w2928, index (col) #2=1, index (row) #3=w2928, index (col) #3=2) -> (element #1=w2929:dbl, element #2=w2931:dbl, element #3=w2930:dbl)
            }
          }
        }
        frame "North west" {
          w2939 = 5
          n386 = case shown="2" w2939 {
            tunnel: [w2943 w2949 w2957 w2965 w2973 w2982 w2989 w2998] -> w2938
            tunnel: [w2945 w2951 w2959 w2966 w2975 w2984 w2991 w3000] -> w2937
            tunnel: [w2944 w2950 w2958 w2967 w2974 w2983 w2990 w2999] -> w2936
            tunnel: w2939 -> [w2947 w2952 w2960 w2968 w2976 w2981 w2992 w2997]
            tunnel: w2935 -> [w2940 w2948 w2956 w2964 w2972 w2980 w2988 w2996]
            frame 0, Default {
              n387 = Index Array(array=w2940, index (row) #1=w2947, index (col) #1=0, index (row) #2=w2947, index (col) #2=1, index (row) #3=w2947, index (col) #3=2) -> (element #1=w2945:dbl, element #2=w2944:dbl, element #3=w2943:dbl)
            }
            frame 1 {
              n388 = Index Array(array=w2948, index (row) #1=w2952, index (col) #1=0, index (row) #2=w2952, index (col) #2=1, index (row) #3=w2952, index (col) #3=2) -> (element #1=w2951:dbl, element #2=w2950:dbl, element #3=w2949:dbl)
            }
            frame 2 {
              n389 = Index Array(array=w2956, index (row) #1=w2960, index (col) #1=0, index (row) #2=w2960, index (col) #2=1, index (row) #3=w2960, index (col) #3=2) -> (element #1=w2959:dbl, element #2=w2958:dbl, element #3=w2957:dbl)
            }
            frame 3 {
              n390 = Index Array(array=w2964, index (row) #1=w2968, index (col) #1=0, index (row) #2=w2968, index (col) #2=1, index (row) #3=w2968, index (col) #3=2) -> (element #1=w2966:dbl, element #2=w2967:dbl, element #3=w2965:dbl)
            }
            frame 4 {
              n391 = Index Array(array=w2972, index (row) #1=w2976, index (col) #1=0, index (row) #2=w2976, index (col) #2=1, index (row) #3=w2976, index (col) #3=2) -> (element #1=w2973:dbl, element #2=w2975:dbl, element #3=w2974:dbl)
            }
            frame 5 {
              n392 = Index Array(array=w2980, index (row) #1=w2981, index (col) #1=0, index (row) #2=w2981, index (col) #2=1, index (row) #3=w2981, index (col) #3=2) -> (element #1=w2982:dbl, element #2=w2983:dbl, element #3=w2984:dbl)
            }
            frame 6 {
              n393 = Index Array(array=w2988, index (row) #1=w2992, index (col) #1=0, index (row) #2=w2992, index (col) #2=1, index (row) #3=w2992, index (col) #3=2) -> (element #1=w2989:dbl, element #2=w2991:dbl, element #3=w2990:dbl)
            }
            frame 7 {
              n394 = Index Array(array=w2996, index (row) #1=w2997, index (col) #1=0, index (row) #2=w2997, index (col) #2=1, index (row) #3=w2997, index (col) #3=2) -> (element #1=w2998:dbl, element #2=w3000:dbl, element #3=w2999:dbl)
            }
          }
        }
        frame "West" {
          w3008 = 3
          n395 = case shown="2" w3008 {
            tunnel: [w3012 w3018 w3026 w3034 w3042 w3051 w3058 w3067] -> w3005
            tunnel: [w3014 w3020 w3028 w3035 w3044 w3053 w3060 w3069] -> w3006
            tunnel: [w3013 w3019 w3027 w3036 w3043 w3052 w3059 w3068] -> w3004
            tunnel: w3008 -> [w3016 w3021 w3029 w3037 w3045 w3050 w3061 w3066]
            tunnel: w3007 -> [w3009 w3017 w3025 w3033 w3041 w3049 w3057 w3065]
            frame 0, Default {
              n396 = Index Array(array=w3009, index (row) #1=w3016, index (col) #1=0, index (row) #2=w3016, index (col) #2=1, index (row) #3=w3016, index (col) #3=2) -> (element #1=w3014:dbl, element #2=w3013:dbl, element #3=w3012:dbl)
            }
            frame 1 {
              n397 = Index Array(array=w3017, index (row) #1=w3021, index (col) #1=0, index (row) #2=w3021, index (col) #2=1, index (row) #3=w3021, index (col) #3=2) -> (element #1=w3020:dbl, element #2=w3019:dbl, element #3=w3018:dbl)
            }
            frame 2 {
              n398 = Index Array(array=w3025, index (row) #1=w3029, index (col) #1=0, index (row) #2=w3029, index (col) #2=1, index (row) #3=w3029, index (col) #3=2) -> (element #1=w3028:dbl, element #2=w3027:dbl, element #3=w3026:dbl)
            }
            frame 3 {
              n399 = Index Array(array=w3033, index (row) #1=w3037, index (col) #1=0, index (row) #2=w3037, index (col) #2=1, index (row) #3=w3037, index (col) #3=2) -> (element #1=w3035:dbl, element #2=w3036:dbl, element #3=w3034:dbl)
            }
            frame 4 {
              n400 = Index Array(array=w3041, index (row) #1=w3045, index (col) #1=0, index (row) #2=w3045, index (col) #2=1, index (row) #3=w3045, index (col) #3=2) -> (element #1=w3042:dbl, element #2=w3044:dbl, element #3=w3043:dbl)
            }
            frame 5 {
              n401 = Index Array(array=w3049, index (row) #1=w3050, index (col) #1=0, index (row) #2=w3050, index (col) #2=1, index (row) #3=w3050, index (col) #3=2) -> (element #1=w3051:dbl, element #2=w3052:dbl, element #3=w3053:dbl)
            }
            frame 6 {
              n402 = Index Array(array=w3057, index (row) #1=w3061, index (col) #1=0, index (row) #2=w3061, index (col) #2=1, index (row) #3=w3061, index (col) #3=2) -> (element #1=w3058:dbl, element #2=w3060:dbl, element #3=w3059:dbl)
            }
            frame 7 {
              n403 = Index Array(array=w3065, index (row) #1=w3066, index (col) #1=0, index (row) #2=w3066, index (col) #2=1, index (row) #3=w3066, index (col) #3=2) -> (element #1=w3067:dbl, element #2=w3069:dbl, element #3=w3068:dbl)
            }
          }
        }
        frame "East" {
          w3077 = 4
          n404 = case shown="2" w3077 {
            tunnel: [w3081 w3087 w3095 w3103 w3111 w3120 w3127 w3136] -> w3075
            tunnel: [w3083 w3089 w3097 w3104 w3113 w3122 w3129 w3138] -> w3074
            tunnel: [w3082 w3088 w3096 w3105 w3112 w3121 w3128 w3137] -> w3073
            tunnel: w3077 -> [w3085 w3090 w3098 w3106 w3114 w3119 w3130 w3135]
            tunnel: w3076 -> [w3078 w3086 w3094 w3102 w3110 w3118 w3126 w3134]
            frame 0, Default {
              n405 = Index Array(array=w3078, index (row) #1=w3085, index (col) #1=0, index (row) #2=w3085, index (col) #2=1, index (row) #3=w3085, index (col) #3=2) -> (element #1=w3083:dbl, element #2=w3082:dbl, element #3=w3081:dbl)
            }
            frame 1 {
              n406 = Index Array(array=w3086, index (row) #1=w3090, index (col) #1=0, index (row) #2=w3090, index (col) #2=1, index (row) #3=w3090, index (col) #3=2) -> (element #1=w3089:dbl, element #2=w3088:dbl, element #3=w3087:dbl)
            }
            frame 2 {
              n407 = Index Array(array=w3094, index (row) #1=w3098, index (col) #1=0, index (row) #2=w3098, index (col) #2=1, index (row) #3=w3098, index (col) #3=2) -> (element #1=w3097:dbl, element #2=w3096:dbl, element #3=w3095:dbl)
            }
            frame 3 {
              n408 = Index Array(array=w3102, index (row) #1=w3106, index (col) #1=0, index (row) #2=w3106, index (col) #2=1, index (row) #3=w3106, index (col) #3=2) -> (element #1=w3104:dbl, element #2=w3105:dbl, element #3=w3103:dbl)
            }
            frame 4 {
              n409 = Index Array(array=w3110, index (row) #1=w3114, index (col) #1=0, index (row) #2=w3114, index (col) #2=1, index (row) #3=w3114, index (col) #3=2) -> (element #1=w3111:dbl, element #2=w3113:dbl, element #3=w3112:dbl)
            }
            frame 5 {
              n410 = Index Array(array=w3118, index (row) #1=w3119, index (col) #1=0, index (row) #2=w3119, index (col) #2=1, index (row) #3=w3119, index (col) #3=2) -> (element #1=w3120:dbl, element #2=w3121:dbl, element #3=w3122:dbl)
            }
            frame 6 {
              n411 = Index Array(array=w3126, index (row) #1=w3130, index (col) #1=0, index (row) #2=w3130, index (col) #2=1, index (row) #3=w3130, index (col) #3=2) -> (element #1=w3127:dbl, element #2=w3129:dbl, element #3=w3128:dbl)
            }
            frame 7 {
              n412 = Index Array(array=w3134, index (row) #1=w3135, index (col) #1=0, index (row) #2=w3135, index (col) #2=1, index (row) #3=w3135, index (col) #3=2) -> (element #1=w3136:dbl, element #2=w3138:dbl, element #3=w3137:dbl)
            }
          }
        }
        frame "South" {
          w3146 = 0
          n413 = case shown="2" w3146 {
            tunnel: [w3150 w3156 w3164 w3172 w3180 w3189 w3196 w3205] -> w3145
            tunnel: [w3152 w3158 w3166 w3173 w3182 w3191 w3198 w3207] -> w3143
            tunnel: [w3151 w3157 w3165 w3174 w3181 w3190 w3197 w3206] -> w3142
            tunnel: w3146 -> [w3154 w3159 w3167 w3175 w3183 w3188 w3199 w3204]
            tunnel: w3144 -> [w3147 w3155 w3163 w3171 w3179 w3187 w3195 w3203]
            frame 0, Default {
              n414 = Index Array(array=w3147, index (row) #1=w3154, index (col) #1=0, index (row) #2=w3154, index (col) #2=1, index (row) #3=w3154, index (col) #3=2) -> (element #1=w3152:dbl, element #2=w3151:dbl, element #3=w3150:dbl)
            }
            frame 1 {
              n415 = Index Array(array=w3155, index (row) #1=w3159, index (col) #1=0, index (row) #2=w3159, index (col) #2=1, index (row) #3=w3159, index (col) #3=2) -> (element #1=w3158:dbl, element #2=w3157:dbl, element #3=w3156:dbl)
            }
            frame 2 {
              n416 = Index Array(array=w3163, index (row) #1=w3167, index (col) #1=0, index (row) #2=w3167, index (col) #2=1, index (row) #3=w3167, index (col) #3=2) -> (element #1=w3166:dbl, element #2=w3165:dbl, element #3=w3164:dbl)
            }
            frame 3 {
              n417 = Index Array(array=w3171, index (row) #1=w3175, index (col) #1=0, index (row) #2=w3175, index (col) #2=1, index (row) #3=w3175, index (col) #3=2) -> (element #1=w3173:dbl, element #2=w3174:dbl, element #3=w3172:dbl)
            }
            frame 4 {
              n418 = Index Array(array=w3179, index (row) #1=w3183, index (col) #1=0, index (row) #2=w3183, index (col) #2=1, index (row) #3=w3183, index (col) #3=2) -> (element #1=w3180:dbl, element #2=w3182:dbl, element #3=w3181:dbl)
            }
            frame 5 {
              n419 = Index Array(array=w3187, index (row) #1=w3188, index (col) #1=0, index (row) #2=w3188, index (col) #2=1, index (row) #3=w3188, index (col) #3=2) -> (element #1=w3189:dbl, element #2=w3190:dbl, element #3=w3191:dbl)
            }
            frame 6 {
              n420 = Index Array(array=w3195, index (row) #1=w3199, index (col) #1=0, index (row) #2=w3199, index (col) #2=1, index (row) #3=w3199, index (col) #3=2) -> (element #1=w3196:dbl, element #2=w3198:dbl, element #3=w3197:dbl)
            }
            frame 7 {
              n421 = Index Array(array=w3203, index (row) #1=w3204, index (col) #1=0, index (row) #2=w3204, index (col) #2=1, index (row) #3=w3204, index (col) #3=2) -> (element #1=w3205:dbl, element #2=w3207:dbl, element #3=w3206:dbl)
            }
          }
        }
        frame "South west" {
          w3215 = 1
          n422 = case shown="2" w3215 {
            tunnel: [w3219 w3225 w3233 w3241 w3249 w3258 w3265 w3274] -> w3213
            tunnel: [w3221 w3227 w3235 w3242 w3251 w3260 w3267 w3276] -> w3212
            tunnel: [w3220 w3226 w3234 w3243 w3250 w3259 w3266 w3275] -> w3211
            tunnel: w3215 -> [w3223 w3228 w3236 w3244 w3252 w3257 w3268 w3273]
            tunnel: w3214 -> [w3216 w3224 w3232 w3240 w3248 w3256 w3264 w3272]
            frame 0, Default {
              n423 = Index Array(array=w3216, index (row) #1=w3223, index (col) #1=0, index (row) #2=w3223, index (col) #2=1, index (row) #3=w3223, index (col) #3=2) -> (element #1=w3221:dbl, element #2=w3220:dbl, element #3=w3219:dbl)
            }
            frame 1 {
              n424 = Index Array(array=w3224, index (row) #1=w3228, index (col) #1=0, index (row) #2=w3228, index (col) #2=1, index (row) #3=w3228, index (col) #3=2) -> (element #1=w3227:dbl, element #2=w3226:dbl, element #3=w3225:dbl)
            }
            frame 2 {
              n425 = Index Array(array=w3232, index (row) #1=w3236, index (col) #1=0, index (row) #2=w3236, index (col) #2=1, index (row) #3=w3236, index (col) #3=2) -> (element #1=w3235:dbl, element #2=w3234:dbl, element #3=w3233:dbl)
            }
            frame 3 {
              n426 = Index Array(array=w3240, index (row) #1=w3244, index (col) #1=0, index (row) #2=w3244, index (col) #2=1, index (row) #3=w3244, index (col) #3=2) -> (element #1=w3242:dbl, element #2=w3243:dbl, element #3=w3241:dbl)
            }
            frame 4 {
              n427 = Index Array(array=w3248, index (row) #1=w3252, index (col) #1=0, index (row) #2=w3252, index (col) #2=1, index (row) #3=w3252, index (col) #3=2) -> (element #1=w3249:dbl, element #2=w3251:dbl, element #3=w3250:dbl)
            }
            frame 5 {
              n428 = Index Array(array=w3256, index (row) #1=w3257, index (col) #1=0, index (row) #2=w3257, index (col) #2=1, index (row) #3=w3257, index (col) #3=2) -> (element #1=w3258:dbl, element #2=w3259:dbl, element #3=w3260:dbl)
            }
            frame 6 {
              n429 = Index Array(array=w3264, index (row) #1=w3268, index (col) #1=0, index (row) #2=w3268, index (col) #2=1, index (row) #3=w3268, index (col) #3=2) -> (element #1=w3265:dbl, element #2=w3267:dbl, element #3=w3266:dbl)
            }
            frame 7 {
              n430 = Index Array(array=w3272, index (row) #1=w3273, index (col) #1=0, index (row) #2=w3273, index (col) #2=1, index (row) #3=w3273, index (col) #3=2) -> (element #1=w3274:dbl, element #2=w3276:dbl, element #3=w3275:dbl)
            }
          }
        }
        frame "South east" {
          w3284 = 2
          n431 = case shown="2" w3284 {
            tunnel: [w3288 w3294 w3302 w3310 w3318 w3327 w3334 w3343] -> w3283
            tunnel: [w3290 w3296 w3304 w3311 w3320 w3329 w3336 w3345] -> w3282
            tunnel: [w3289 w3295 w3303 w3312 w3319 w3328 w3335 w3344] -> w3281
            tunnel: w3284 -> [w3292 w3297 w3305 w3313 w3321 w3326 w3337 w3342]
            tunnel: w3280 -> [w3285 w3293 w3301 w3309 w3317 w3325 w3333 w3341]
            frame 0, Default {
              n432 = Index Array(array=w3285, index (row) #1=w3292, index (col) #1=0, index (row) #2=w3292, index (col) #2=1, index (row) #3=w3292, index (col) #3=2) -> (element #1=w3290:dbl, element #2=w3289:dbl, element #3=w3288:dbl)
            }
            frame 1 {
              n433 = Index Array(array=w3293, index (row) #1=w3297, index (col) #1=0, index (row) #2=w3297, index (col) #2=1, index (row) #3=w3297, index (col) #3=2) -> (element #1=w3296:dbl, element #2=w3295:dbl, element #3=w3294:dbl)
            }
            frame 2 {
              n434 = Index Array(array=w3301, index (row) #1=w3305, index (col) #1=0, index (row) #2=w3305, index (col) #2=1, index (row) #3=w3305, index (col) #3=2) -> (element #1=w3304:dbl, element #2=w3303:dbl, element #3=w3302:dbl)
            }
            frame 3 {
              n435 = Index Array(array=w3309, index (row) #1=w3313, index (col) #1=0, index (row) #2=w3313, index (col) #2=1, index (row) #3=w3313, index (col) #3=2) -> (element #1=w3311:dbl, element #2=w3312:dbl, element #3=w3310:dbl)
            }
            frame 4 {
              n436 = Index Array(array=w3317, index (row) #1=w3321, index (col) #1=0, index (row) #2=w3321, index (col) #2=1, index (row) #3=w3321, index (col) #3=2) -> (element #1=w3318:dbl, element #2=w3320:dbl, element #3=w3319:dbl)
            }
            frame 5 {
              n437 = Index Array(array=w3325, index (row) #1=w3326, index (col) #1=0, index (row) #2=w3326, index (col) #2=1, index (row) #3=w3326, index (col) #3=2) -> (element #1=w3327:dbl, element #2=w3328:dbl, element #3=w3329:dbl)
            }
            frame 6 {
              n438 = Index Array(array=w3333, index (row) #1=w3337, index (col) #1=0, index (row) #2=w3337, index (col) #2=1, index (row) #3=w3337, index (col) #3=2) -> (element #1=w3334:dbl, element #2=w3336:dbl, element #3=w3335:dbl)
            }
            frame 7 {
              n439 = Index Array(array=w3341, index (row) #1=w3342, index (col) #1=0, index (row) #2=w3342, index (col) #2=1, index (row) #3=w3342, index (col) #3=2) -> (element #1=w3343:dbl, element #2=w3345:dbl, element #3=w3344:dbl)
            }
          }
        }
      }
    }
    frame "South west" {
      n440 = case shown="\"North\", Default" w3350 {
        tunnel: [w3357 w3427 w3495 w3562 w3632 w3702 w3770 w3840] -> w3353
        tunnel: [w3356 w3426 w3494 w3563 w3631 w3700 w3769 w3839] -> w3352
        tunnel: [w3355 w3425 w3493 w3561 w3630 w3699 w3768 w3838] -> w3351
        tunnel: w3349 -> [w3354 w3423 w3492 w3564 w3633 w3701 w3771 w3837]
        frame "North", Default {
          w3358 = 6
          n441 = case shown="2" w3358 {
            tunnel: [w3362 w3368 w3376 w3384 w3392 w3401 w3408 w3417] -> w3357
            tunnel: [w3364 w3370 w3378 w3385 w3394 w3403 w3410 w3419] -> w3356
            tunnel: [w3363 w3369 w3377 w3386 w3393 w3402 w3409 w3418] -> w3355
            tunnel: w3358 -> [w3366 w3371 w3379 w3387 w3395 w3400 w3411 w3416]
            tunnel: w3354 -> [w3359 w3367 w3375 w3383 w3391 w3399 w3407 w3415]
            frame 0, Default {
              n442 = Index Array(array=w3359, index (row) #1=w3366, index (col) #1=0, index (row) #2=w3366, index (col) #2=1, index (row) #3=w3366, index (col) #3=2) -> (element #1=w3364:dbl, element #2=w3363:dbl, element #3=w3362:dbl)
            }
            frame 1 {
              n443 = Index Array(array=w3367, index (row) #1=w3371, index (col) #1=0, index (row) #2=w3371, index (col) #2=1, index (row) #3=w3371, index (col) #3=2) -> (element #1=w3370:dbl, element #2=w3369:dbl, element #3=w3368:dbl)
            }
            frame 2 {
              n444 = Index Array(array=w3375, index (row) #1=w3379, index (col) #1=0, index (row) #2=w3379, index (col) #2=1, index (row) #3=w3379, index (col) #3=2) -> (element #1=w3378:dbl, element #2=w3377:dbl, element #3=w3376:dbl)
            }
            frame 3 {
              n445 = Index Array(array=w3383, index (row) #1=w3387, index (col) #1=0, index (row) #2=w3387, index (col) #2=1, index (row) #3=w3387, index (col) #3=2) -> (element #1=w3385:dbl, element #2=w3386:dbl, element #3=w3384:dbl)
            }
            frame 4 {
              n446 = Index Array(array=w3391, index (row) #1=w3395, index (col) #1=0, index (row) #2=w3395, index (col) #2=1, index (row) #3=w3395, index (col) #3=2) -> (element #1=w3392:dbl, element #2=w3394:dbl, element #3=w3393:dbl)
            }
            frame 5 {
              n447 = Index Array(array=w3399, index (row) #1=w3400, index (col) #1=0, index (row) #2=w3400, index (col) #2=1, index (row) #3=w3400, index (col) #3=2) -> (element #1=w3401:dbl, element #2=w3402:dbl, element #3=w3403:dbl)
            }
            frame 6 {
              n448 = Index Array(array=w3407, index (row) #1=w3411, index (col) #1=0, index (row) #2=w3411, index (col) #2=1, index (row) #3=w3411, index (col) #3=2) -> (element #1=w3408:dbl, element #2=w3410:dbl, element #3=w3409:dbl)
            }
            frame 7 {
              n449 = Index Array(array=w3415, index (row) #1=w3416, index (col) #1=0, index (row) #2=w3416, index (col) #2=1, index (row) #3=w3416, index (col) #3=2) -> (element #1=w3417:dbl, element #2=w3419:dbl, element #3=w3418:dbl)
            }
          }
        }
        frame "North east" {
          w3424 = 7
          n450 = case shown="2" w3424 {
            tunnel: [w3431 w3437 w3445 w3453 w3461 w3470 w3477 w3486] -> w3427
            tunnel: [w3433 w3439 w3447 w3454 w3463 w3472 w3479 w3488] -> w3426
            tunnel: [w3432 w3438 w3446 w3455 w3462 w3471 w3478 w3487] -> w3425
            tunnel: w3424 -> [w3435 w3440 w3448 w3456 w3464 w3469 w3480 w3485]
            tunnel: w3423 -> [w3428 w3436 w3444 w3452 w3460 w3468 w3476 w3484]
            frame 0, Default {
              n451 = Index Array(array=w3428, index (row) #1=w3435, index (col) #1=0, index (row) #2=w3435, index (col) #2=1, index (row) #3=w3435, index (col) #3=2) -> (element #1=w3433:dbl, element #2=w3432:dbl, element #3=w3431:dbl)
            }
            frame 1 {
              n452 = Index Array(array=w3436, index (row) #1=w3440, index (col) #1=0, index (row) #2=w3440, index (col) #2=1, index (row) #3=w3440, index (col) #3=2) -> (element #1=w3439:dbl, element #2=w3438:dbl, element #3=w3437:dbl)
            }
            frame 2 {
              n453 = Index Array(array=w3444, index (row) #1=w3448, index (col) #1=0, index (row) #2=w3448, index (col) #2=1, index (row) #3=w3448, index (col) #3=2) -> (element #1=w3447:dbl, element #2=w3446:dbl, element #3=w3445:dbl)
            }
            frame 3 {
              n454 = Index Array(array=w3452, index (row) #1=w3456, index (col) #1=0, index (row) #2=w3456, index (col) #2=1, index (row) #3=w3456, index (col) #3=2) -> (element #1=w3454:dbl, element #2=w3455:dbl, element #3=w3453:dbl)
            }
            frame 4 {
              n455 = Index Array(array=w3460, index (row) #1=w3464, index (col) #1=0, index (row) #2=w3464, index (col) #2=1, index (row) #3=w3464, index (col) #3=2) -> (element #1=w3461:dbl, element #2=w3463:dbl, element #3=w3462:dbl)
            }
            frame 5 {
              n456 = Index Array(array=w3468, index (row) #1=w3469, index (col) #1=0, index (row) #2=w3469, index (col) #2=1, index (row) #3=w3469, index (col) #3=2) -> (element #1=w3470:dbl, element #2=w3471:dbl, element #3=w3472:dbl)
            }
            frame 6 {
              n457 = Index Array(array=w3476, index (row) #1=w3480, index (col) #1=0, index (row) #2=w3480, index (col) #2=1, index (row) #3=w3480, index (col) #3=2) -> (element #1=w3477:dbl, element #2=w3479:dbl, element #3=w3478:dbl)
            }
            frame 7 {
              n458 = Index Array(array=w3484, index (row) #1=w3485, index (col) #1=0, index (row) #2=w3485, index (col) #2=1, index (row) #3=w3485, index (col) #3=2) -> (element #1=w3486:dbl, element #2=w3488:dbl, element #3=w3487:dbl)
            }
          }
        }
        frame "North west" {
          w3496 = 4
          n459 = case shown="2" w3496 {
            tunnel: [w3500 w3506 w3514 w3522 w3530 w3539 w3546 w3555] -> w3495
            tunnel: [w3502 w3508 w3516 w3523 w3532 w3541 w3548 w3557] -> w3494
            tunnel: [w3501 w3507 w3515 w3524 w3531 w3540 w3547 w3556] -> w3493
            tunnel: w3496 -> [w3504 w3509 w3517 w3525 w3533 w3538 w3549 w3554]
            tunnel: w3492 -> [w3497 w3505 w3513 w3521 w3529 w3537 w3545 w3553]
            frame 0, Default {
              n460 = Index Array(array=w3497, index (row) #1=w3504, index (col) #1=0, index (row) #2=w3504, index (col) #2=1, index (row) #3=w3504, index (col) #3=2) -> (element #1=w3502:dbl, element #2=w3501:dbl, element #3=w3500:dbl)
            }
            frame 1 {
              n461 = Index Array(array=w3505, index (row) #1=w3509, index (col) #1=0, index (row) #2=w3509, index (col) #2=1, index (row) #3=w3509, index (col) #3=2) -> (element #1=w3508:dbl, element #2=w3507:dbl, element #3=w3506:dbl)
            }
            frame 2 {
              n462 = Index Array(array=w3513, index (row) #1=w3517, index (col) #1=0, index (row) #2=w3517, index (col) #2=1, index (row) #3=w3517, index (col) #3=2) -> (element #1=w3516:dbl, element #2=w3515:dbl, element #3=w3514:dbl)
            }
            frame 3 {
              n463 = Index Array(array=w3521, index (row) #1=w3525, index (col) #1=0, index (row) #2=w3525, index (col) #2=1, index (row) #3=w3525, index (col) #3=2) -> (element #1=w3523:dbl, element #2=w3524:dbl, element #3=w3522:dbl)
            }
            frame 4 {
              n464 = Index Array(array=w3529, index (row) #1=w3533, index (col) #1=0, index (row) #2=w3533, index (col) #2=1, index (row) #3=w3533, index (col) #3=2) -> (element #1=w3530:dbl, element #2=w3532:dbl, element #3=w3531:dbl)
            }
            frame 5 {
              n465 = Index Array(array=w3537, index (row) #1=w3538, index (col) #1=0, index (row) #2=w3538, index (col) #2=1, index (row) #3=w3538, index (col) #3=2) -> (element #1=w3539:dbl, element #2=w3540:dbl, element #3=w3541:dbl)
            }
            frame 6 {
              n466 = Index Array(array=w3545, index (row) #1=w3549, index (col) #1=0, index (row) #2=w3549, index (col) #2=1, index (row) #3=w3549, index (col) #3=2) -> (element #1=w3546:dbl, element #2=w3548:dbl, element #3=w3547:dbl)
            }
            frame 7 {
              n467 = Index Array(array=w3553, index (row) #1=w3554, index (col) #1=0, index (row) #2=w3554, index (col) #2=1, index (row) #3=w3554, index (col) #3=2) -> (element #1=w3555:dbl, element #2=w3557:dbl, element #3=w3556:dbl)
            }
          }
        }
        frame "West" {
          w3565 = 2
          n468 = case shown="2" w3565 {
            tunnel: [w3569 w3575 w3583 w3591 w3599 w3608 w3615 w3624] -> w3562
            tunnel: [w3571 w3577 w3585 w3592 w3601 w3610 w3617 w3626] -> w3563
            tunnel: [w3570 w3576 w3584 w3593 w3600 w3609 w3616 w3625] -> w3561
            tunnel: w3565 -> [w3573 w3578 w3586 w3594 w3602 w3607 w3618 w3623]
            tunnel: w3564 -> [w3566 w3574 w3582 w3590 w3598 w3606 w3614 w3622]
            frame 0, Default {
              n469 = Index Array(array=w3566, index (row) #1=w3573, index (col) #1=0, index (row) #2=w3573, index (col) #2=1, index (row) #3=w3573, index (col) #3=2) -> (element #1=w3571:dbl, element #2=w3570:dbl, element #3=w3569:dbl)
            }
            frame 1 {
              n470 = Index Array(array=w3574, index (row) #1=w3578, index (col) #1=0, index (row) #2=w3578, index (col) #2=1, index (row) #3=w3578, index (col) #3=2) -> (element #1=w3577:dbl, element #2=w3576:dbl, element #3=w3575:dbl)
            }
            frame 2 {
              n471 = Index Array(array=w3582, index (row) #1=w3586, index (col) #1=0, index (row) #2=w3586, index (col) #2=1, index (row) #3=w3586, index (col) #3=2) -> (element #1=w3585:dbl, element #2=w3584:dbl, element #3=w3583:dbl)
            }
            frame 3 {
              n472 = Index Array(array=w3590, index (row) #1=w3594, index (col) #1=0, index (row) #2=w3594, index (col) #2=1, index (row) #3=w3594, index (col) #3=2) -> (element #1=w3592:dbl, element #2=w3593:dbl, element #3=w3591:dbl)
            }
            frame 4 {
              n473 = Index Array(array=w3598, index (row) #1=w3602, index (col) #1=0, index (row) #2=w3602, index (col) #2=1, index (row) #3=w3602, index (col) #3=2) -> (element #1=w3599:dbl, element #2=w3601:dbl, element #3=w3600:dbl)
            }
            frame 5 {
              n474 = Index Array(array=w3606, index (row) #1=w3607, index (col) #1=0, index (row) #2=w3607, index (col) #2=1, index (row) #3=w3607, index (col) #3=2) -> (element #1=w3608:dbl, element #2=w3609:dbl, element #3=w3610:dbl)
            }
            frame 6 {
              n475 = Index Array(array=w3614, index (row) #1=w3618, index (col) #1=0, index (row) #2=w3618, index (col) #2=1, index (row) #3=w3618, index (col) #3=2) -> (element #1=w3615:dbl, element #2=w3617:dbl, element #3=w3616:dbl)
            }
            frame 7 {
              n476 = Index Array(array=w3622, index (row) #1=w3623, index (col) #1=0, index (row) #2=w3623, index (col) #2=1, index (row) #3=w3623, index (col) #3=2) -> (element #1=w3624:dbl, element #2=w3626:dbl, element #3=w3625:dbl)
            }
          }
        }
        frame "East" {
          w3634 = 5
          n477 = case shown="2" w3634 {
            tunnel: [w3638 w3644 w3652 w3660 w3668 w3677 w3684 w3693] -> w3632
            tunnel: [w3640 w3646 w3654 w3661 w3670 w3679 w3686 w3695] -> w3631
            tunnel: [w3639 w3645 w3653 w3662 w3669 w3678 w3685 w3694] -> w3630
            tunnel: w3634 -> [w3642 w3647 w3655 w3663 w3671 w3676 w3687 w3692]
            tunnel: w3633 -> [w3635 w3643 w3651 w3659 w3667 w3675 w3683 w3691]
            frame 0, Default {
              n478 = Index Array(array=w3635, index (row) #1=w3642, index (col) #1=0, index (row) #2=w3642, index (col) #2=1, index (row) #3=w3642, index (col) #3=2) -> (element #1=w3640:dbl, element #2=w3639:dbl, element #3=w3638:dbl)
            }
            frame 1 {
              n479 = Index Array(array=w3643, index (row) #1=w3647, index (col) #1=0, index (row) #2=w3647, index (col) #2=1, index (row) #3=w3647, index (col) #3=2) -> (element #1=w3646:dbl, element #2=w3645:dbl, element #3=w3644:dbl)
            }
            frame 2 {
              n480 = Index Array(array=w3651, index (row) #1=w3655, index (col) #1=0, index (row) #2=w3655, index (col) #2=1, index (row) #3=w3655, index (col) #3=2) -> (element #1=w3654:dbl, element #2=w3653:dbl, element #3=w3652:dbl)
            }
            frame 3 {
              n481 = Index Array(array=w3659, index (row) #1=w3663, index (col) #1=0, index (row) #2=w3663, index (col) #2=1, index (row) #3=w3663, index (col) #3=2) -> (element #1=w3661:dbl, element #2=w3662:dbl, element #3=w3660:dbl)
            }
            frame 4 {
              n482 = Index Array(array=w3667, index (row) #1=w3671, index (col) #1=0, index (row) #2=w3671, index (col) #2=1, index (row) #3=w3671, index (col) #3=2) -> (element #1=w3668:dbl, element #2=w3670:dbl, element #3=w3669:dbl)
            }
            frame 5 {
              n483 = Index Array(array=w3675, index (row) #1=w3676, index (col) #1=0, index (row) #2=w3676, index (col) #2=1, index (row) #3=w3676, index (col) #3=2) -> (element #1=w3677:dbl, element #2=w3678:dbl, element #3=w3679:dbl)
            }
            frame 6 {
              n484 = Index Array(array=w3683, index (row) #1=w3687, index (col) #1=0, index (row) #2=w3687, index (col) #2=1, index (row) #3=w3687, index (col) #3=2) -> (element #1=w3684:dbl, element #2=w3686:dbl, element #3=w3685:dbl)
            }
            frame 7 {
              n485 = Index Array(array=w3691, index (row) #1=w3692, index (col) #1=0, index (row) #2=w3692, index (col) #2=1, index (row) #3=w3692, index (col) #3=2) -> (element #1=w3693:dbl, element #2=w3695:dbl, element #3=w3694:dbl)
            }
          }
        }
        frame "South" {
          w3703 = 1
          n486 = case shown="2" w3703 {
            tunnel: [w3707 w3713 w3721 w3729 w3737 w3746 w3753 w3762] -> w3702
            tunnel: [w3709 w3715 w3723 w3730 w3739 w3748 w3755 w3764] -> w3700
            tunnel: [w3708 w3714 w3722 w3731 w3738 w3747 w3754 w3763] -> w3699
            tunnel: w3703 -> [w3711 w3716 w3724 w3732 w3740 w3745 w3756 w3761]
            tunnel: w3701 -> [w3704 w3712 w3720 w3728 w3736 w3744 w3752 w3760]
            frame 0, Default {
              n487 = Index Array(array=w3704, index (row) #1=w3711, index (col) #1=0, index (row) #2=w3711, index (col) #2=1, index (row) #3=w3711, index (col) #3=2) -> (element #1=w3709:dbl, element #2=w3708:dbl, element #3=w3707:dbl)
            }
            frame 1 {
              n488 = Index Array(array=w3712, index (row) #1=w3716, index (col) #1=0, index (row) #2=w3716, index (col) #2=1, index (row) #3=w3716, index (col) #3=2) -> (element #1=w3715:dbl, element #2=w3714:dbl, element #3=w3713:dbl)
            }
            frame 2 {
              n489 = Index Array(array=w3720, index (row) #1=w3724, index (col) #1=0, index (row) #2=w3724, index (col) #2=1, index (row) #3=w3724, index (col) #3=2) -> (element #1=w3723:dbl, element #2=w3722:dbl, element #3=w3721:dbl)
            }
            frame 3 {
              n490 = Index Array(array=w3728, index (row) #1=w3732, index (col) #1=0, index (row) #2=w3732, index (col) #2=1, index (row) #3=w3732, index (col) #3=2) -> (element #1=w3730:dbl, element #2=w3731:dbl, element #3=w3729:dbl)
            }
            frame 4 {
              n491 = Index Array(array=w3736, index (row) #1=w3740, index (col) #1=0, index (row) #2=w3740, index (col) #2=1, index (row) #3=w3740, index (col) #3=2) -> (element #1=w3737:dbl, element #2=w3739:dbl, element #3=w3738:dbl)
            }
            frame 5 {
              n492 = Index Array(array=w3744, index (row) #1=w3745, index (col) #1=0, index (row) #2=w3745, index (col) #2=1, index (row) #3=w3745, index (col) #3=2) -> (element #1=w3746:dbl, element #2=w3747:dbl, element #3=w3748:dbl)
            }
            frame 6 {
              n493 = Index Array(array=w3752, index (row) #1=w3756, index (col) #1=0, index (row) #2=w3756, index (col) #2=1, index (row) #3=w3756, index (col) #3=2) -> (element #1=w3753:dbl, element #2=w3755:dbl, element #3=w3754:dbl)
            }
            frame 7 {
              n494 = Index Array(array=w3760, index (row) #1=w3761, index (col) #1=0, index (row) #2=w3761, index (col) #2=1, index (row) #3=w3761, index (col) #3=2) -> (element #1=w3762:dbl, element #2=w3764:dbl, element #3=w3763:dbl)
            }
          }
        }
        frame "South west" {
          w3772 = 0
          n495 = case shown="2" w3772 {
            tunnel: [w3776 w3782 w3790 w3798 w3806 w3815 w3822 w3831] -> w3770
            tunnel: [w3778 w3784 w3792 w3799 w3808 w3817 w3824 w3833] -> w3769
            tunnel: [w3777 w3783 w3791 w3800 w3807 w3816 w3823 w3832] -> w3768
            tunnel: w3772 -> [w3780 w3785 w3793 w3801 w3809 w3814 w3825 w3830]
            tunnel: w3771 -> [w3773 w3781 w3789 w3797 w3805 w3813 w3821 w3829]
            frame 0, Default {
              n496 = Index Array(array=w3773, index (row) #1=w3780, index (col) #1=0, index (row) #2=w3780, index (col) #2=1, index (row) #3=w3780, index (col) #3=2) -> (element #1=w3778:dbl, element #2=w3777:dbl, element #3=w3776:dbl)
            }
            frame 1 {
              n497 = Index Array(array=w3781, index (row) #1=w3785, index (col) #1=0, index (row) #2=w3785, index (col) #2=1, index (row) #3=w3785, index (col) #3=2) -> (element #1=w3784:dbl, element #2=w3783:dbl, element #3=w3782:dbl)
            }
            frame 2 {
              n498 = Index Array(array=w3789, index (row) #1=w3793, index (col) #1=0, index (row) #2=w3793, index (col) #2=1, index (row) #3=w3793, index (col) #3=2) -> (element #1=w3792:dbl, element #2=w3791:dbl, element #3=w3790:dbl)
            }
            frame 3 {
              n499 = Index Array(array=w3797, index (row) #1=w3801, index (col) #1=0, index (row) #2=w3801, index (col) #2=1, index (row) #3=w3801, index (col) #3=2) -> (element #1=w3799:dbl, element #2=w3800:dbl, element #3=w3798:dbl)
            }
            frame 4 {
              n500 = Index Array(array=w3805, index (row) #1=w3809, index (col) #1=0, index (row) #2=w3809, index (col) #2=1, index (row) #3=w3809, index (col) #3=2) -> (element #1=w3806:dbl, element #2=w3808:dbl, element #3=w3807:dbl)
            }
            frame 5 {
              n501 = Index Array(array=w3813, index (row) #1=w3814, index (col) #1=0, index (row) #2=w3814, index (col) #2=1, index (row) #3=w3814, index (col) #3=2) -> (element #1=w3815:dbl, element #2=w3816:dbl, element #3=w3817:dbl)
            }
            frame 6 {
              n502 = Index Array(array=w3821, index (row) #1=w3825, index (col) #1=0, index (row) #2=w3825, index (col) #2=1, index (row) #3=w3825, index (col) #3=2) -> (element #1=w3822:dbl, element #2=w3824:dbl, element #3=w3823:dbl)
            }
            frame 7 {
              n503 = Index Array(array=w3829, index (row) #1=w3830, index (col) #1=0, index (row) #2=w3830, index (col) #2=1, index (row) #3=w3830, index (col) #3=2) -> (element #1=w3831:dbl, element #2=w3833:dbl, element #3=w3832:dbl)
            }
          }
        }
        frame "South east" {
          w3841 = 3
          n504 = case shown="2" w3841 {
            tunnel: [w3845 w3851 w3859 w3867 w3875 w3884 w3891 w3900] -> w3840
            tunnel: [w3847 w3853 w3861 w3868 w3877 w3886 w3893 w3902] -> w3839
            tunnel: [w3846 w3852 w3860 w3869 w3876 w3885 w3892 w3901] -> w3838
            tunnel: w3841 -> [w3849 w3854 w3862 w3870 w3878 w3883 w3894 w3899]
            tunnel: w3837 -> [w3842 w3850 w3858 w3866 w3874 w3882 w3890 w3898]
            frame 0, Default {
              n505 = Index Array(array=w3842, index (row) #1=w3849, index (col) #1=0, index (row) #2=w3849, index (col) #2=1, index (row) #3=w3849, index (col) #3=2) -> (element #1=w3847:dbl, element #2=w3846:dbl, element #3=w3845:dbl)
            }
            frame 1 {
              n506 = Index Array(array=w3850, index (row) #1=w3854, index (col) #1=0, index (row) #2=w3854, index (col) #2=1, index (row) #3=w3854, index (col) #3=2) -> (element #1=w3853:dbl, element #2=w3852:dbl, element #3=w3851:dbl)
            }
            frame 2 {
              n507 = Index Array(array=w3858, index (row) #1=w3862, index (col) #1=0, index (row) #2=w3862, index (col) #2=1, index (row) #3=w3862, index (col) #3=2) -> (element #1=w3861:dbl, element #2=w3860:dbl, element #3=w3859:dbl)
            }
            frame 3 {
              n508 = Index Array(array=w3866, index (row) #1=w3870, index (col) #1=0, index (row) #2=w3870, index (col) #2=1, index (row) #3=w3870, index (col) #3=2) -> (element #1=w3868:dbl, element #2=w3869:dbl, element #3=w3867:dbl)
            }
            frame 4 {
              n509 = Index Array(array=w3874, index (row) #1=w3878, index (col) #1=0, index (row) #2=w3878, index (col) #2=1, index (row) #3=w3878, index (col) #3=2) -> (element #1=w3875:dbl, element #2=w3877:dbl, element #3=w3876:dbl)
            }
            frame 5 {
              n510 = Index Array(array=w3882, index (row) #1=w3883, index (col) #1=0, index (row) #2=w3883, index (col) #2=1, index (row) #3=w3883, index (col) #3=2) -> (element #1=w3884:dbl, element #2=w3885:dbl, element #3=w3886:dbl)
            }
            frame 6 {
              n511 = Index Array(array=w3890, index (row) #1=w3894, index (col) #1=0, index (row) #2=w3894, index (col) #2=1, index (row) #3=w3894, index (col) #3=2) -> (element #1=w3891:dbl, element #2=w3893:dbl, element #3=w3892:dbl)
            }
            frame 7 {
              n512 = Index Array(array=w3898, index (row) #1=w3899, index (col) #1=0, index (row) #2=w3899, index (col) #2=1, index (row) #3=w3899, index (col) #3=2) -> (element #1=w3900:dbl, element #2=w3902:dbl, element #3=w3901:dbl)
            }
          }
        }
      }
    }
    frame "South east" {
      n513 = case shown="\"North\", Default" w3907 {
        tunnel: [w3914 w3984 w4052 w4119 w4189 w4259 w4327 w4397] -> w3910
        tunnel: [w3913 w3983 w4051 w4120 w4188 w4257 w4326 w4396] -> w3909
        tunnel: [w3912 w3982 w4050 w4118 w4187 w4256 w4325 w4395] -> w3908
        tunnel: w3906 -> [w3911 w3980 w4049 w4121 w4190 w4258 w4328 w4394]
        frame "North", Default {
          w3915 = 5
          n514 = case shown="2" w3915 {
            tunnel: [w3919 w3925 w3933 w3941 w3949 w3958 w3965 w3974] -> w3914
            tunnel: [w3921 w3927 w3935 w3942 w3951 w3960 w3967 w3976] -> w3913
            tunnel: [w3920 w3926 w3934 w3943 w3950 w3959 w3966 w3975] -> w3912
            tunnel: w3915 -> [w3923 w3928 w3936 w3944 w3952 w3957 w3968 w3973]
            tunnel: w3911 -> [w3916 w3924 w3932 w3940 w3948 w3956 w3964 w3972]
            frame 0, Default {
              n515 = Index Array(array=w3916, index (row) #1=w3923, index (col) #1=0, index (row) #2=w3923, index (col) #2=1, index (row) #3=w3923, index (col) #3=2) -> (element #1=w3921:dbl, element #2=w3920:dbl, element #3=w3919:dbl)
            }
            frame 1 {
              n516 = Index Array(array=w3924, index (row) #1=w3928, index (col) #1=0, index (row) #2=w3928, index (col) #2=1, index (row) #3=w3928, index (col) #3=2) -> (element #1=w3927:dbl, element #2=w3926:dbl, element #3=w3925:dbl)
            }
            frame 2 {
              n517 = Index Array(array=w3932, index (row) #1=w3936, index (col) #1=0, index (row) #2=w3936, index (col) #2=1, index (row) #3=w3936, index (col) #3=2) -> (element #1=w3935:dbl, element #2=w3934:dbl, element #3=w3933:dbl)
            }
            frame 3 {
              n518 = Index Array(array=w3940, index (row) #1=w3944, index (col) #1=0, index (row) #2=w3944, index (col) #2=1, index (row) #3=w3944, index (col) #3=2) -> (element #1=w3942:dbl, element #2=w3943:dbl, element #3=w3941:dbl)
            }
            frame 4 {
              n519 = Index Array(array=w3948, index (row) #1=w3952, index (col) #1=0, index (row) #2=w3952, index (col) #2=1, index (row) #3=w3952, index (col) #3=2) -> (element #1=w3949:dbl, element #2=w3951:dbl, element #3=w3950:dbl)
            }
            frame 5 {
              n520 = Index Array(array=w3956, index (row) #1=w3957, index (col) #1=0, index (row) #2=w3957, index (col) #2=1, index (row) #3=w3957, index (col) #3=2) -> (element #1=w3958:dbl, element #2=w3959:dbl, element #3=w3960:dbl)
            }
            frame 6 {
              n521 = Index Array(array=w3964, index (row) #1=w3968, index (col) #1=0, index (row) #2=w3968, index (col) #2=1, index (row) #3=w3968, index (col) #3=2) -> (element #1=w3965:dbl, element #2=w3967:dbl, element #3=w3966:dbl)
            }
            frame 7 {
              n522 = Index Array(array=w3972, index (row) #1=w3973, index (col) #1=0, index (row) #2=w3973, index (col) #2=1, index (row) #3=w3973, index (col) #3=2) -> (element #1=w3974:dbl, element #2=w3976:dbl, element #3=w3975:dbl)
            }
          }
        }
        frame "North east" {
          w3981 = 3
          n523 = case shown="2" w3981 {
            tunnel: [w3988 w3994 w4002 w4010 w4018 w4027 w4034 w4043] -> w3984
            tunnel: [w3990 w3996 w4004 w4011 w4020 w4029 w4036 w4045] -> w3983
            tunnel: [w3989 w3995 w4003 w4012 w4019 w4028 w4035 w4044] -> w3982
            tunnel: w3981 -> [w3992 w3997 w4005 w4013 w4021 w4026 w4037 w4042]
            tunnel: w3980 -> [w3985 w3993 w4001 w4009 w4017 w4025 w4033 w4041]
            frame 0, Default {
              n524 = Index Array(array=w3985, index (row) #1=w3992, index (col) #1=0, index (row) #2=w3992, index (col) #2=1, index (row) #3=w3992, index (col) #3=2) -> (element #1=w3990:dbl, element #2=w3989:dbl, element #3=w3988:dbl)
            }
            frame 1 {
              n525 = Index Array(array=w3993, index (row) #1=w3997, index (col) #1=0, index (row) #2=w3997, index (col) #2=1, index (row) #3=w3997, index (col) #3=2) -> (element #1=w3996:dbl, element #2=w3995:dbl, element #3=w3994:dbl)
            }
            frame 2 {
              n526 = Index Array(array=w4001, index (row) #1=w4005, index (col) #1=0, index (row) #2=w4005, index (col) #2=1, index (row) #3=w4005, index (col) #3=2) -> (element #1=w4004:dbl, element #2=w4003:dbl, element #3=w4002:dbl)
            }
            frame 3 {
              n527 = Index Array(array=w4009, index (row) #1=w4013, index (col) #1=0, index (row) #2=w4013, index (col) #2=1, index (row) #3=w4013, index (col) #3=2) -> (element #1=w4011:dbl, element #2=w4012:dbl, element #3=w4010:dbl)
            }
            frame 4 {
              n528 = Index Array(array=w4017, index (row) #1=w4021, index (col) #1=0, index (row) #2=w4021, index (col) #2=1, index (row) #3=w4021, index (col) #3=2) -> (element #1=w4018:dbl, element #2=w4020:dbl, element #3=w4019:dbl)
            }
            frame 5 {
              n529 = Index Array(array=w4025, index (row) #1=w4026, index (col) #1=0, index (row) #2=w4026, index (col) #2=1, index (row) #3=w4026, index (col) #3=2) -> (element #1=w4027:dbl, element #2=w4028:dbl, element #3=w4029:dbl)
            }
            frame 6 {
              n530 = Index Array(array=w4033, index (row) #1=w4037, index (col) #1=0, index (row) #2=w4037, index (col) #2=1, index (row) #3=w4037, index (col) #3=2) -> (element #1=w4034:dbl, element #2=w4036:dbl, element #3=w4035:dbl)
            }
            frame 7 {
              n531 = Index Array(array=w4041, index (row) #1=w4042, index (col) #1=0, index (row) #2=w4042, index (col) #2=1, index (row) #3=w4042, index (col) #3=2) -> (element #1=w4043:dbl, element #2=w4045:dbl, element #3=w4044:dbl)
            }
          }
        }
        frame "North west" {
          w4053 = 7
          n532 = case shown="2" w4053 {
            tunnel: [w4057 w4063 w4071 w4079 w4087 w4096 w4103 w4112] -> w4052
            tunnel: [w4059 w4065 w4073 w4080 w4089 w4098 w4105 w4114] -> w4051
            tunnel: [w4058 w4064 w4072 w4081 w4088 w4097 w4104 w4113] -> w4050
            tunnel: w4053 -> [w4061 w4066 w4074 w4082 w4090 w4095 w4106 w4111]
            tunnel: w4049 -> [w4054 w4062 w4070 w4078 w4086 w4094 w4102 w4110]
            frame 0, Default {
              n533 = Index Array(array=w4054, index (row) #1=w4061, index (col) #1=0, index (row) #2=w4061, index (col) #2=1, index (row) #3=w4061, index (col) #3=2) -> (element #1=w4059:dbl, element #2=w4058:dbl, element #3=w4057:dbl)
            }
            frame 1 {
              n534 = Index Array(array=w4062, index (row) #1=w4066, index (col) #1=0, index (row) #2=w4066, index (col) #2=1, index (row) #3=w4066, index (col) #3=2) -> (element #1=w4065:dbl, element #2=w4064:dbl, element #3=w4063:dbl)
            }
            frame 2 {
              n535 = Index Array(array=w4070, index (row) #1=w4074, index (col) #1=0, index (row) #2=w4074, index (col) #2=1, index (row) #3=w4074, index (col) #3=2) -> (element #1=w4073:dbl, element #2=w4072:dbl, element #3=w4071:dbl)
            }
            frame 3 {
              n536 = Index Array(array=w4078, index (row) #1=w4082, index (col) #1=0, index (row) #2=w4082, index (col) #2=1, index (row) #3=w4082, index (col) #3=2) -> (element #1=w4080:dbl, element #2=w4081:dbl, element #3=w4079:dbl)
            }
            frame 4 {
              n537 = Index Array(array=w4086, index (row) #1=w4090, index (col) #1=0, index (row) #2=w4090, index (col) #2=1, index (row) #3=w4090, index (col) #3=2) -> (element #1=w4087:dbl, element #2=w4089:dbl, element #3=w4088:dbl)
            }
            frame 5 {
              n538 = Index Array(array=w4094, index (row) #1=w4095, index (col) #1=0, index (row) #2=w4095, index (col) #2=1, index (row) #3=w4095, index (col) #3=2) -> (element #1=w4096:dbl, element #2=w4097:dbl, element #3=w4098:dbl)
            }
            frame 6 {
              n539 = Index Array(array=w4102, index (row) #1=w4106, index (col) #1=0, index (row) #2=w4106, index (col) #2=1, index (row) #3=w4106, index (col) #3=2) -> (element #1=w4103:dbl, element #2=w4105:dbl, element #3=w4104:dbl)
            }
            frame 7 {
              n540 = Index Array(array=w4110, index (row) #1=w4111, index (col) #1=0, index (row) #2=w4111, index (col) #2=1, index (row) #3=w4111, index (col) #3=2) -> (element #1=w4112:dbl, element #2=w4114:dbl, element #3=w4113:dbl)
            }
          }
        }
        frame "West" {
          w4122 = 6
          n541 = case shown="2" w4122 {
            tunnel: [w4126 w4132 w4140 w4148 w4156 w4165 w4172 w4181] -> w4119
            tunnel: [w4128 w4134 w4142 w4149 w4158 w4167 w4174 w4183] -> w4120
            tunnel: [w4127 w4133 w4141 w4150 w4157 w4166 w4173 w4182] -> w4118
            tunnel: w4122 -> [w4130 w4135 w4143 w4151 w4159 w4164 w4175 w4180]
            tunnel: w4121 -> [w4123 w4131 w4139 w4147 w4155 w4163 w4171 w4179]
            frame 0, Default {
              n542 = Index Array(array=w4123, index (row) #1=w4130, index (col) #1=0, index (row) #2=w4130, index (col) #2=1, index (row) #3=w4130, index (col) #3=2) -> (element #1=w4128:dbl, element #2=w4127:dbl, element #3=w4126:dbl)
            }
            frame 1 {
              n543 = Index Array(array=w4131, index (row) #1=w4135, index (col) #1=0, index (row) #2=w4135, index (col) #2=1, index (row) #3=w4135, index (col) #3=2) -> (element #1=w4134:dbl, element #2=w4133:dbl, element #3=w4132:dbl)
            }
            frame 2 {
              n544 = Index Array(array=w4139, index (row) #1=w4143, index (col) #1=0, index (row) #2=w4143, index (col) #2=1, index (row) #3=w4143, index (col) #3=2) -> (element #1=w4142:dbl, element #2=w4141:dbl, element #3=w4140:dbl)
            }
            frame 3 {
              n545 = Index Array(array=w4147, index (row) #1=w4151, index (col) #1=0, index (row) #2=w4151, index (col) #2=1, index (row) #3=w4151, index (col) #3=2) -> (element #1=w4149:dbl, element #2=w4150:dbl, element #3=w4148:dbl)
            }
            frame 4 {
              n546 = Index Array(array=w4155, index (row) #1=w4159, index (col) #1=0, index (row) #2=w4159, index (col) #2=1, index (row) #3=w4159, index (col) #3=2) -> (element #1=w4156:dbl, element #2=w4158:dbl, element #3=w4157:dbl)
            }
            frame 5 {
              n547 = Index Array(array=w4163, index (row) #1=w4164, index (col) #1=0, index (row) #2=w4164, index (col) #2=1, index (row) #3=w4164, index (col) #3=2) -> (element #1=w4165:dbl, element #2=w4166:dbl, element #3=w4167:dbl)
            }
            frame 6 {
              n548 = Index Array(array=w4171, index (row) #1=w4175, index (col) #1=0, index (row) #2=w4175, index (col) #2=1, index (row) #3=w4175, index (col) #3=2) -> (element #1=w4172:dbl, element #2=w4174:dbl, element #3=w4173:dbl)
            }
            frame 7 {
              n549 = Index Array(array=w4179, index (row) #1=w4180, index (col) #1=0, index (row) #2=w4180, index (col) #2=1, index (row) #3=w4180, index (col) #3=2) -> (element #1=w4181:dbl, element #2=w4183:dbl, element #3=w4182:dbl)
            }
          }
        }
        frame "East" {
          w4191 = 1
          n550 = case shown="2" w4191 {
            tunnel: [w4195 w4201 w4209 w4217 w4225 w4234 w4241 w4250] -> w4189
            tunnel: [w4197 w4203 w4211 w4218 w4227 w4236 w4243 w4252] -> w4188
            tunnel: [w4196 w4202 w4210 w4219 w4226 w4235 w4242 w4251] -> w4187
            tunnel: w4191 -> [w4199 w4204 w4212 w4220 w4228 w4233 w4244 w4249]
            tunnel: w4190 -> [w4192 w4200 w4208 w4216 w4224 w4232 w4240 w4248]
            frame 0, Default {
              n551 = Index Array(array=w4192, index (row) #1=w4199, index (col) #1=0, index (row) #2=w4199, index (col) #2=1, index (row) #3=w4199, index (col) #3=2) -> (element #1=w4197:dbl, element #2=w4196:dbl, element #3=w4195:dbl)
            }
            frame 1 {
              n552 = Index Array(array=w4200, index (row) #1=w4204, index (col) #1=0, index (row) #2=w4204, index (col) #2=1, index (row) #3=w4204, index (col) #3=2) -> (element #1=w4203:dbl, element #2=w4202:dbl, element #3=w4201:dbl)
            }
            frame 2 {
              n553 = Index Array(array=w4208, index (row) #1=w4212, index (col) #1=0, index (row) #2=w4212, index (col) #2=1, index (row) #3=w4212, index (col) #3=2) -> (element #1=w4211:dbl, element #2=w4210:dbl, element #3=w4209:dbl)
            }
            frame 3 {
              n554 = Index Array(array=w4216, index (row) #1=w4220, index (col) #1=0, index (row) #2=w4220, index (col) #2=1, index (row) #3=w4220, index (col) #3=2) -> (element #1=w4218:dbl, element #2=w4219:dbl, element #3=w4217:dbl)
            }
            frame 4 {
              n555 = Index Array(array=w4224, index (row) #1=w4228, index (col) #1=0, index (row) #2=w4228, index (col) #2=1, index (row) #3=w4228, index (col) #3=2) -> (element #1=w4225:dbl, element #2=w4227:dbl, element #3=w4226:dbl)
            }
            frame 5 {
              n556 = Index Array(array=w4232, index (row) #1=w4233, index (col) #1=0, index (row) #2=w4233, index (col) #2=1, index (row) #3=w4233, index (col) #3=2) -> (element #1=w4234:dbl, element #2=w4235:dbl, element #3=w4236:dbl)
            }
            frame 6 {
              n557 = Index Array(array=w4240, index (row) #1=w4244, index (col) #1=0, index (row) #2=w4244, index (col) #2=1, index (row) #3=w4244, index (col) #3=2) -> (element #1=w4241:dbl, element #2=w4243:dbl, element #3=w4242:dbl)
            }
            frame 7 {
              n558 = Index Array(array=w4248, index (row) #1=w4249, index (col) #1=0, index (row) #2=w4249, index (col) #2=1, index (row) #3=w4249, index (col) #3=2) -> (element #1=w4250:dbl, element #2=w4252:dbl, element #3=w4251:dbl)
            }
          }
        }
        frame "South" {
          w4260 = 2
          n559 = case shown="2" w4260 {
            tunnel: [w4264 w4270 w4278 w4286 w4294 w4303 w4310 w4319] -> w4259
            tunnel: [w4266 w4272 w4280 w4287 w4296 w4305 w4312 w4321] -> w4257
            tunnel: [w4265 w4271 w4279 w4288 w4295 w4304 w4311 w4320] -> w4256
            tunnel: w4260 -> [w4268 w4273 w4281 w4289 w4297 w4302 w4313 w4318]
            tunnel: w4258 -> [w4261 w4269 w4277 w4285 w4293 w4301 w4309 w4317]
            frame 0, Default {
              n560 = Index Array(array=w4261, index (row) #1=w4268, index (col) #1=0, index (row) #2=w4268, index (col) #2=1, index (row) #3=w4268, index (col) #3=2) -> (element #1=w4266:dbl, element #2=w4265:dbl, element #3=w4264:dbl)
            }
            frame 1 {
              n561 = Index Array(array=w4269, index (row) #1=w4273, index (col) #1=0, index (row) #2=w4273, index (col) #2=1, index (row) #3=w4273, index (col) #3=2) -> (element #1=w4272:dbl, element #2=w4271:dbl, element #3=w4270:dbl)
            }
            frame 2 {
              n562 = Index Array(array=w4277, index (row) #1=w4281, index (col) #1=0, index (row) #2=w4281, index (col) #2=1, index (row) #3=w4281, index (col) #3=2) -> (element #1=w4280:dbl, element #2=w4279:dbl, element #3=w4278:dbl)
            }
            frame 3 {
              n563 = Index Array(array=w4285, index (row) #1=w4289, index (col) #1=0, index (row) #2=w4289, index (col) #2=1, index (row) #3=w4289, index (col) #3=2) -> (element #1=w4287:dbl, element #2=w4288:dbl, element #3=w4286:dbl)
            }
            frame 4 {
              n564 = Index Array(array=w4293, index (row) #1=w4297, index (col) #1=0, index (row) #2=w4297, index (col) #2=1, index (row) #3=w4297, index (col) #3=2) -> (element #1=w4294:dbl, element #2=w4296:dbl, element #3=w4295:dbl)
            }
            frame 5 {
              n565 = Index Array(array=w4301, index (row) #1=w4302, index (col) #1=0, index (row) #2=w4302, index (col) #2=1, index (row) #3=w4302, index (col) #3=2) -> (element #1=w4303:dbl, element #2=w4304:dbl, element #3=w4305:dbl)
            }
            frame 6 {
              n566 = Index Array(array=w4309, index (row) #1=w4313, index (col) #1=0, index (row) #2=w4313, index (col) #2=1, index (row) #3=w4313, index (col) #3=2) -> (element #1=w4310:dbl, element #2=w4312:dbl, element #3=w4311:dbl)
            }
            frame 7 {
              n567 = Index Array(array=w4317, index (row) #1=w4318, index (col) #1=0, index (row) #2=w4318, index (col) #2=1, index (row) #3=w4318, index (col) #3=2) -> (element #1=w4319:dbl, element #2=w4321:dbl, element #3=w4320:dbl)
            }
          }
        }
        frame "South west" {
          w4329 = 4
          n568 = case shown="2" w4329 {
            tunnel: [w4333 w4339 w4347 w4355 w4363 w4372 w4379 w4388] -> w4327
            tunnel: [w4335 w4341 w4349 w4356 w4365 w4374 w4381 w4390] -> w4326
            tunnel: [w4334 w4340 w4348 w4357 w4364 w4373 w4380 w4389] -> w4325
            tunnel: w4329 -> [w4337 w4342 w4350 w4358 w4366 w4371 w4382 w4387]
            tunnel: w4328 -> [w4330 w4338 w4346 w4354 w4362 w4370 w4378 w4386]
            frame 0, Default {
              n569 = Index Array(array=w4330, index (row) #1=w4337, index (col) #1=0, index (row) #2=w4337, index (col) #2=1, index (row) #3=w4337, index (col) #3=2) -> (element #1=w4335:dbl, element #2=w4334:dbl, element #3=w4333:dbl)
            }
            frame 1 {
              n570 = Index Array(array=w4338, index (row) #1=w4342, index (col) #1=0, index (row) #2=w4342, index (col) #2=1, index (row) #3=w4342, index (col) #3=2) -> (element #1=w4341:dbl, element #2=w4340:dbl, element #3=w4339:dbl)
            }
            frame 2 {
              n571 = Index Array(array=w4346, index (row) #1=w4350, index (col) #1=0, index (row) #2=w4350, index (col) #2=1, index (row) #3=w4350, index (col) #3=2) -> (element #1=w4349:dbl, element #2=w4348:dbl, element #3=w4347:dbl)
            }
            frame 3 {
              n572 = Index Array(array=w4354, index (row) #1=w4358, index (col) #1=0, index (row) #2=w4358, index (col) #2=1, index (row) #3=w4358, index (col) #3=2) -> (element #1=w4356:dbl, element #2=w4357:dbl, element #3=w4355:dbl)
            }
            frame 4 {
              n573 = Index Array(array=w4362, index (row) #1=w4366, index (col) #1=0, index (row) #2=w4366, index (col) #2=1, index (row) #3=w4366, index (col) #3=2) -> (element #1=w4363:dbl, element #2=w4365:dbl, element #3=w4364:dbl)
            }
            frame 5 {
              n574 = Index Array(array=w4370, index (row) #1=w4371, index (col) #1=0, index (row) #2=w4371, index (col) #2=1, index (row) #3=w4371, index (col) #3=2) -> (element #1=w4372:dbl, element #2=w4373:dbl, element #3=w4374:dbl)
            }
            frame 6 {
              n575 = Index Array(array=w4378, index (row) #1=w4382, index (col) #1=0, index (row) #2=w4382, index (col) #2=1, index (row) #3=w4382, index (col) #3=2) -> (element #1=w4379:dbl, element #2=w4381:dbl, element #3=w4380:dbl)
            }
            frame 7 {
              n576 = Index Array(array=w4386, index (row) #1=w4387, index (col) #1=0, index (row) #2=w4387, index (col) #2=1, index (row) #3=w4387, index (col) #3=2) -> (element #1=w4388:dbl, element #2=w4390:dbl, element #3=w4389:dbl)
            }
          }
        }
        frame "South east" {
          w4398 = 0
          n577 = case shown="2" w4398 {
            tunnel: [w4402 w4408 w4416 w4424 w4432 w4441 w4448 w4457] -> w4397
            tunnel: [w4404 w4410 w4418 w4425 w4434 w4443 w4450 w4459] -> w4396
            tunnel: [w4403 w4409 w4417 w4426 w4433 w4442 w4449 w4458] -> w4395
            tunnel: w4398 -> [w4406 w4411 w4419 w4427 w4435 w4440 w4451 w4456]
            tunnel: w4394 -> [w4399 w4407 w4415 w4423 w4431 w4439 w4447 w4455]
            frame 0, Default {
              n578 = Index Array(array=w4399, index (row) #1=w4406, index (col) #1=0, index (row) #2=w4406, index (col) #2=1, index (row) #3=w4406, index (col) #3=2) -> (element #1=w4404:dbl, element #2=w4403:dbl, element #3=w4402:dbl)
            }
            frame 1 {
              n579 = Index Array(array=w4407, index (row) #1=w4411, index (col) #1=0, index (row) #2=w4411, index (col) #2=1, index (row) #3=w4411, index (col) #3=2) -> (element #1=w4410:dbl, element #2=w4409:dbl, element #3=w4408:dbl)
            }
            frame 2 {
              n580 = Index Array(array=w4415, index (row) #1=w4419, index (col) #1=0, index (row) #2=w4419, index (col) #2=1, index (row) #3=w4419, index (col) #3=2) -> (element #1=w4418:dbl, element #2=w4417:dbl, element #3=w4416:dbl)
            }
            frame 3 {
              n581 = Index Array(array=w4423, index (row) #1=w4427, index (col) #1=0, index (row) #2=w4427, index (col) #2=1, index (row) #3=w4427, index (col) #3=2) -> (element #1=w4425:dbl, element #2=w4426:dbl, element #3=w4424:dbl)
            }
            frame 4 {
              n582 = Index Array(array=w4431, index (row) #1=w4435, index (col) #1=0, index (row) #2=w4435, index (col) #2=1, index (row) #3=w4435, index (col) #3=2) -> (element #1=w4432:dbl, element #2=w4434:dbl, element #3=w4433:dbl)
            }
            frame 5 {
              n583 = Index Array(array=w4439, index (row) #1=w4440, index (col) #1=0, index (row) #2=w4440, index (col) #2=1, index (row) #3=w4440, index (col) #3=2) -> (element #1=w4441:dbl, element #2=w4442:dbl, element #3=w4443:dbl)
            }
            frame 6 {
              n584 = Index Array(array=w4447, index (row) #1=w4451, index (col) #1=0, index (row) #2=w4451, index (col) #2=1, index (row) #3=w4451, index (col) #3=2) -> (element #1=w4448:dbl, element #2=w4450:dbl, element #3=w4449:dbl)
            }
            frame 7 {
              n585 = Index Array(array=w4455, index (row) #1=w4456, index (col) #1=0, index (row) #2=w4456, index (col) #2=1, index (row) #3=w4456, index (col) #3=2) -> (element #1=w4457:dbl, element #2=w4459:dbl, element #3=w4458:dbl)
            }
          }
        }
      }
    }
  }
  n586 = local write "chosen  distance"(w2) -> ()
  n587 = Equal?(x=w2, y=0) -> (x = y?=w3:bool)
  n588 = case shown="False" w3 {
    frame True {
    }
    frame False {
      n589 = flat-sequence {
        tunnel: u8 40 ("Slave Address (7-bit)") -> [w4473]
        tunnel: "error in (no error)" -> [w4474]
        tunnel: [w4474] -> w4464
        tunnel: [w4473] -> w4463
        tunnel: [w4476] -> w4472
        tunnel: [w4478] -> w4471
        tunnel: w4464 -> [w4477]
        tunnel: w4463 -> [w4478]
        tunnel: w4472 -> [w4483]
        tunnel: [w4483] -> w4470
        tunnel: w4471 -> [w4479]
        tunnel: [w4479] -> w4469
        tunnel: w4470 -> [w4486]
        tunnel: w4469 -> [w4485]
        tunnel: [w4484] -> w4468
        tunnel: [w4698] -> w4465
        tunnel: w4468 -> [w4698]
        frame #0 {
          n590 = call "new initialize.vi"() -> ()  [unwired: 12 in]
        }
        frame #1 {
          n591 = call "new imu.vi"("error in (no error)"=w4477) -> ("Numeric"=→"First location":dbl, "error out"=w4476:errorcluster)  [unwired: 9 in]
        }
        frame #2 {
          n592 = local read "First location"() -> (w4482:dbl)
          n593 = Add(x="chosen  distance", y=w4482) -> (x+y=→"Final location":dbl)
        }
        frame #3 {
          n594 = while {
            tunnel: w4486 -> [w4490]
            tunnel: [w4498] -> w4484
            tunnel: w4485 -> [w4497]
            stop <- w4496 stop-if-true
            n595 = flat-sequence {
              tunnel: [w4501] -> w4494
              tunnel: [w4500] -> w4491
              tunnel: w4497 -> [_]
              tunnel: w4490 -> [w4499]
              tunnel: w4494 -> [w4505]
              tunnel: [w4505] -> w4493
              tunnel: [w4504] -> w4492
              tunnel: w4491 -> [w4503]
              tunnel: w4493 -> [w4522]
              tunnel: [w4522] -> w4489
              tunnel: w4492 -> [w4519]
              tunnel: w4489 -> [w4530]
              tunnel: [w4529] -> w4496
              tunnel: [w4530] -> w4495
              tunnel: [w4527] -> w4488
              tunnel: [w4526] -> w4487
              tunnel: w4495 -> [w4627]
              tunnel: [w4627] -> w4498
              tunnel: w4488 -> [w4621]
              tunnel: w4487 -> [w4620]
              frame #0 {
                n596 = call "new imu.vi"("error in (no error)"=w4499) -> ("Numeric"=w4500:dbl, "error out"=w4501:errorcluster)  [unwired: 9 in]
              }
              frame #1 {
                n597 = local read "Final location"() -> (w4504:dbl)
                n598 = case shown="..0" w4504 {
                  tunnel: w4503 -> [w4506 w4513 w4518]
                  tunnel: [w4507 w4512 w4518] -> w4502
                  frame 360.. {
                    n599 = case shown="..89" w4506 {
                      tunnel: [w4508 w4510] -> w4507
                      tunnel: w4506 -> [w4508 w4509]
                      frame 90.., Default {
                      }
                      frame ..89 {
                        n600 = Add(x=360.0, y=w4509) -> (x+y=w4510:dbl)
                      }
                    }
                  }
                  frame ..0 {
                    n601 = case shown="90.., Default" w4513 {
                      tunnel: [w4516 w4517] -> w4512
                      tunnel: w4513 -> [w4515 w4517]
                      frame 90.., Default {
                        n602 = Subtract(x=w4515, y=360) -> (x-y=w4516:dbl)
                      }
                      frame ..89 {
                      }
                    }
                  }
                  frame 1..359, Default {
                  }
                }
                "Current location" <- w4502
              }
              frame #2 {
                n603 = local read "Current location"() -> (w4521:dbl)
                n604 = Subtract(x=w4519, y=w4521) -> (x-y=→"remainder":dbl)
              }
              frame #3 {
                n605 = local read "remainder"() -> (w4524:dbl)
                n606 = case shown="1.." w4524 {
                  tunnel: [TRUE FALSE FALSE] -> w4529
                  tunnel: [0.75 0.66 0.84] -> w4525
                  tunnel: w4524 -> [w4601 w4604 w4614]
                  tunnel: [w4601 w4605 w4612] -> w4523
                  frame 0, Default {
                  }
                  frame 1.. {
                    n607 = case shown="10..25" w4604 {
                      tunnel: [200.0 25.0 300.0] -> w4605
                      frame 10..25 {
                      }
                      frame 0, Default {
                      }
                      frame 26.. {
                      }
                    }
                  }
                  frame ..-1 {
                    n608 = Multiply(x=w4614, y=-1) -> (x*y=w4611:dbl)
                    n609 = case shown="10..25" w4611 {
                      tunnel: [200.0 35.0 300.0] -> w4612
                      frame 10..25 {
                      }
                      frame 0, Default {
                      }
                      frame 26.. {
                      }
                    }
                  }
                }
                n610 = xnode "PWM"("Duty Cycle"=w4525, "error in (no error)"="error in (no error) 2") -> ("error out"=w4527:errorcluster)
                n611 = xnode "PWM 2"("Duty Cycle"=w4525, "error in (no error)"="error in (no error) 2") -> ("error out"=w4526:errorcluster)
                n612 = Wait (ms)(milliseconds to wait=w4523) -> ()  [unwired: 1 out]
              }
              frame #4 {
                n613 = xnode "PWM 3"("Duty Cycle"=0.75, "error in (no error)"=w4620) -> ("error out"=→"error out 4":errorcluster)
                n614 = Wait (ms)(milliseconds to wait=50) -> ()  [unwired: 1 out]
                n615 = xnode "PWM 4"("Duty Cycle"=0.75, "error in (no error)"=w4621) -> ("error out"=→"error out 5":errorcluster)
              }
            }
          }
        }
        frame #4 {
        }
      }
      "error out" <- w4465
    }
  }
